vi "输出数据解析.vi"(0 "主板引用":refnum<vi>, 1 "错误代码":i32, 2 "BMU读取结果":refnum<vi>, 3 "命令序号":u8, 4 "输入数组":u8[](array[numeric]), 5 "命令":u8 format="%x", 6 "从板引用":refnum<vi>, 9 "进度引用":refnum<vi>, 10 "板选择":enum16{"主板", "从板"}(ring), 11 "从板个数":refnum<vi>, 12 "二维码信息":refnum<vi>, 13 "从板二维码信息":refnum<vi>, 15 "Socket":dbl) -> (14 "从板数":u8, 17 "写入超时":bool=TRUE, 18 "序号":u8, 19 "状态":bool)   [LabVIEW 2013]
panel:
  in  "从板个数 2":dbl=1.0
  out "子字符串之前":string
  out "从板信息":T1
  out "主板数据 2":T2
  out "充电控制参数":bool
  out "二级故障1 2":bool
  out "一级故障1 6":bool
  out "一级故障1 5":bool
  out "二级故障1":bool
  out "一级故障5":bool
  out "一级故障1 4":bool
  out "一级故障1 3":bool
  out "一级故障1 2":bool
  out "一级故障1":bool
  in  "Ctl引用句柄":refnum<vi>
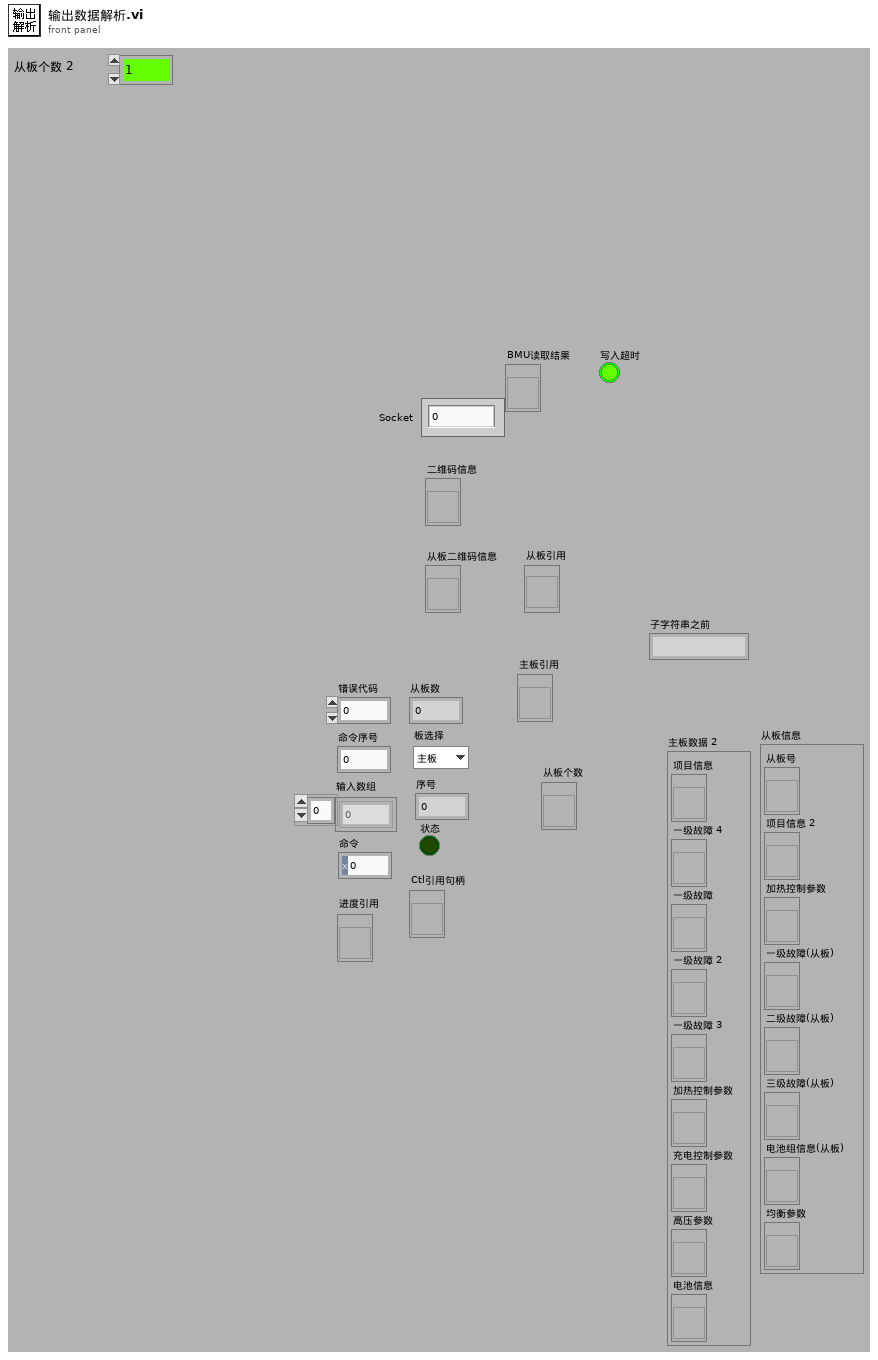
[diagram p1: front panel]
types:
  T1 = cluster{"从板号":refnum<vi>, "项目信息 2":refnum<vi>, "加热控制参数":refnum<vi>, "一级故障(从板)":refnum<vi>, "二级故障(从板)":refnum<vi>, "三级故障(从板)":refnum<vi>, "电池组信息(从板)":refnum<vi>, "均衡参数":refnum<vi>}
  T2 = cluster{"项目信息":refnum<vi>, "一级故障 4":refnum<vi>, "一级故障":refnum<vi>, "一级故障 2":refnum<vi>, "一级故障 3":refnum<vi>, "加热控制参数":refnum<vi>, "充电控制参数":refnum<vi>, "高压参数":refnum<vi>, "电池信息":refnum<vi>}
  T3 = cluster{"电池额定容量":dbl, "使用者":dbl, "电池实际容量":dbl, "车牌号":string, "配置文件版本":string, "SOH":dbl, "SOC":dbl, "产品编号":string, "系统时钟":string}
  T4 = cluster{"电池额定容量(A)":dbl, "使用者":dbl, "电池实际容量(A)":dbl, "车架(牌)号":string, "配置文件版本":string, "SOH(%)":dbl, "SOC(%)":dbl, "产品编号":string, "系统时钟":string}
  T5 = cluster{"总电压过高":dbl, "整组电压不均衡":dbl, "SOC过高":dbl, "单体电压过高":dbl, "总电压过低":dbl, "温度过高":dbl, "温度过低":dbl, "单组电压不均衡":dbl, "整组温度不均衡":dbl, "单组温度不均衡":dbl, "单体电压过低":dbl, "充电电流过高":dbl, "放电电流过高":dbl, "SOC过低":dbl, "内阻过大":dbl, "极柱温度过高":dbl, "SOH过低":dbl}
  T6 = cluster{"风机开启温度":dbl, "风机关闭温度":dbl, "加热开启温度":dbl, "加热关闭温度":dbl, "风机开启温差":dbl, "风机关闭温差":dbl, "加热关闭温差":dbl}
  T7 = cluster{"最大允许单体电压":dbl, "最大允许总电压":dbl, "最小允许单体电压":dbl, "最大允许充电电流":dbl, "最小允许充电电流":dbl, "最大允许充电温度":dbl, "最小允许充电温度":dbl, "电流步长":dbl}
  T8 = cluster{"充电能量阀值":dbl, "放电能量阀值":dbl, "电流增益":dbl, "平均电流":dbl, "电压增益":dbl, "平均电压":dbl}
  T9 = cluster{"电池串联":dbl, "电池并联":dbl, "累计放电总安时":dbl, "电池包额定容量":dbl, "电池包额定能量":dbl, "电池包额定总电压":dbl, "累计充电总安时":dbl, "电池充满次数":dbl, "电池放空次数":dbl, "电池充电次数":dbl, "电池生产日期":string, "电池厂家":string, "电池类型":string, "电池包组号":string, "电池包产权标识":string, "电池应用车型":string, "实际容量":dbl}
  T10 = cluster{"从板号":bool, "电压起始值":bool, "通道电压数":bool, "保险位置":bool, "温度起始值":bool, "一级故障":bool, "二级故障":bool, "三级故障":bool}
  T11 = cluster{"电压过高":dbl, "电压过低":dbl, "温度过高":dbl, "温度过低":dbl, "电压不均衡(V)":dbl, "温度不均衡":dbl, "SOC过低":dbl}
  T12 = cluster{"串联数":dbl, "并联数":dbl, "电池厂家":dbl, "电池类型":dbl, "额定能量":dbl, "额定容量":dbl, "实际容量":dbl, "额定总压":dbl, "产权标识":dbl, "应用车型":dbl, "电池包组号":dbl, "SOC":dbl, "充电总安时":dbl, "放电总这时":dbl, "放空次数":dbl, "充满次数":dbl, "充电次数":dbl, "车牌号":string, "生产日期":string, "最大允许单体电压":dbl, "最大允许总电压":dbl, "最大允许温度":dbl, "最小允许温度":dbl, "最大允许充电电流":dbl, "最小允许充电电流":dbl, "最小允许单体电压":dbl, "电流步长":dbl, "电池包序号":dbl}
  T13 = cluster{"充电结束电压(90%)":sgl, "充电结束电压(91%)":sgl, "充电结束电压(92%)":sgl, "充电结束电压(93%)":sgl, "充电结束电压(94%)":sgl, "均衡计算-电压高阀值1级":sgl, "均衡计算-电压高阀值2级":sgl, "均衡计算-电压低阀值1级":sgl, "均衡计算-电压低阀值2级":sgl, "均衡计算-最低电压阀值":sgl, "均衡停止-最低电压阀值":sgl, "均衡计算-电压极差阀值":sgl, "充电结束电压(95%)":sgl, "充电结束电压(96%)":sgl, "充电结束电压(97%)":sgl, "充电结束电压(98%)":sgl, "充电结束电压(99%)":sgl, "充电结束电压(100%)":sgl}
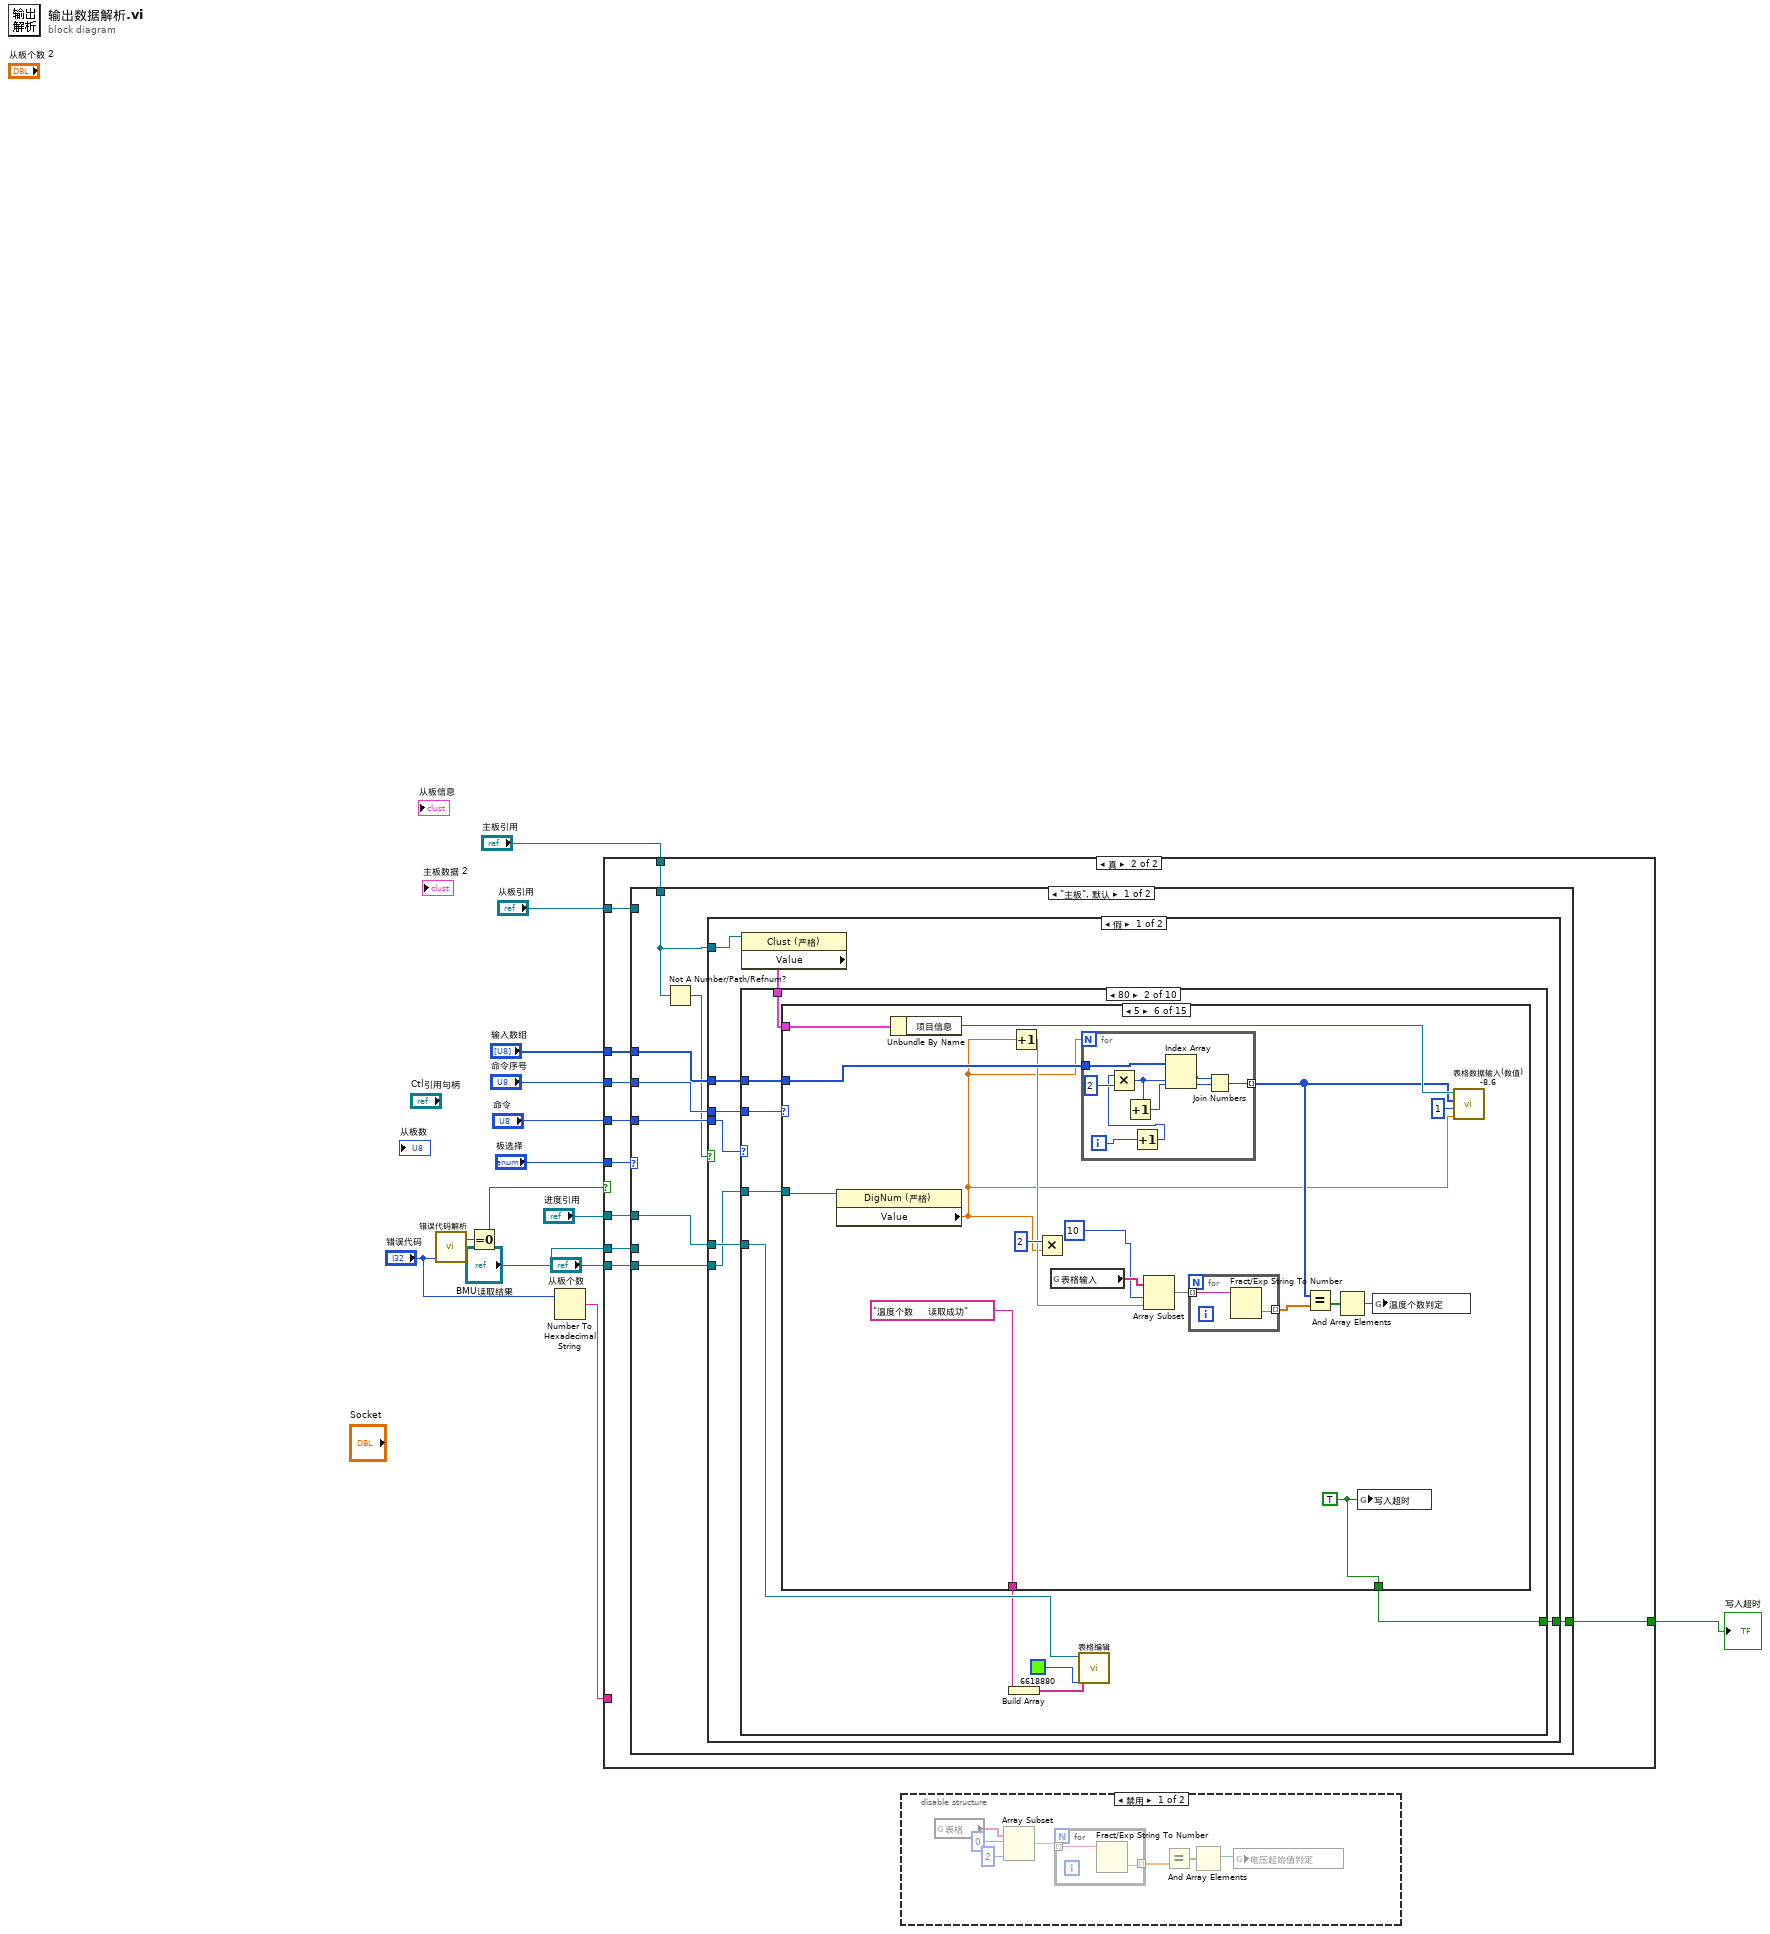
[diagram p0: block diagram]
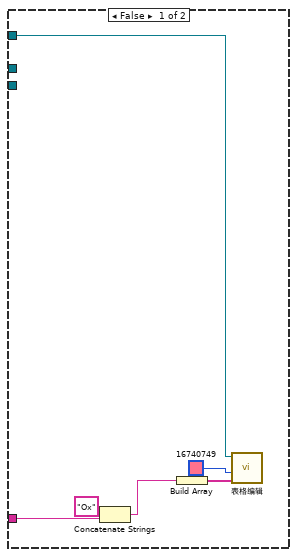
[diagram p3: hidden frame]
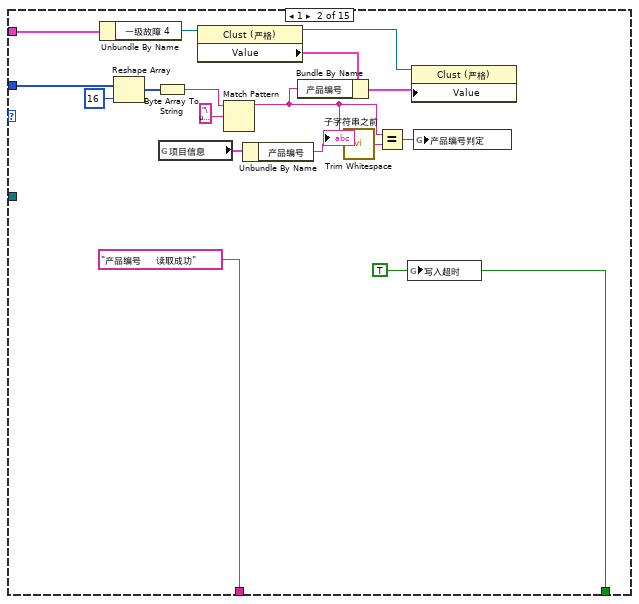
[diagram p6: hidden frame]
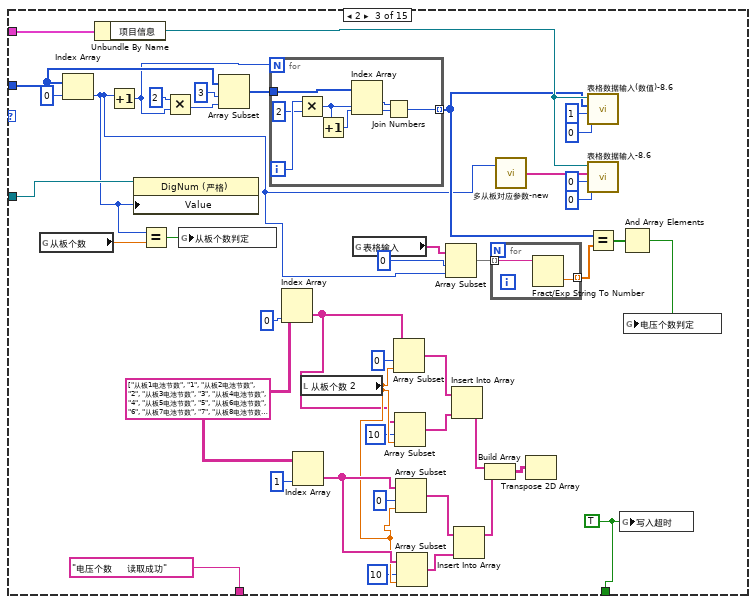
[diagram p7: hidden frame]
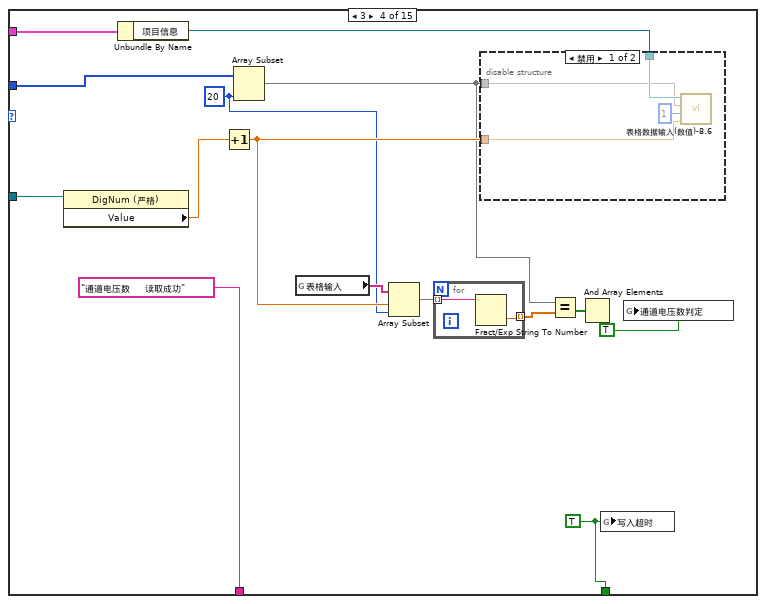
[diagram p8: hidden frame]
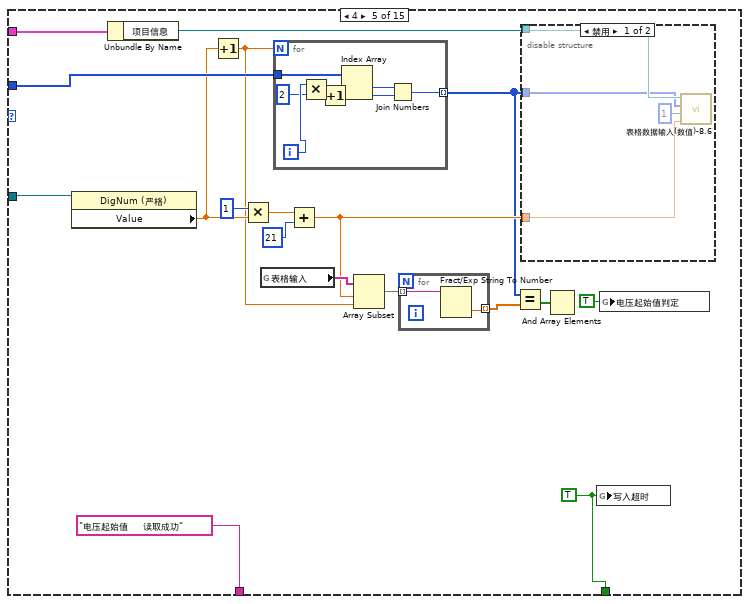
[diagram p10: hidden frame]
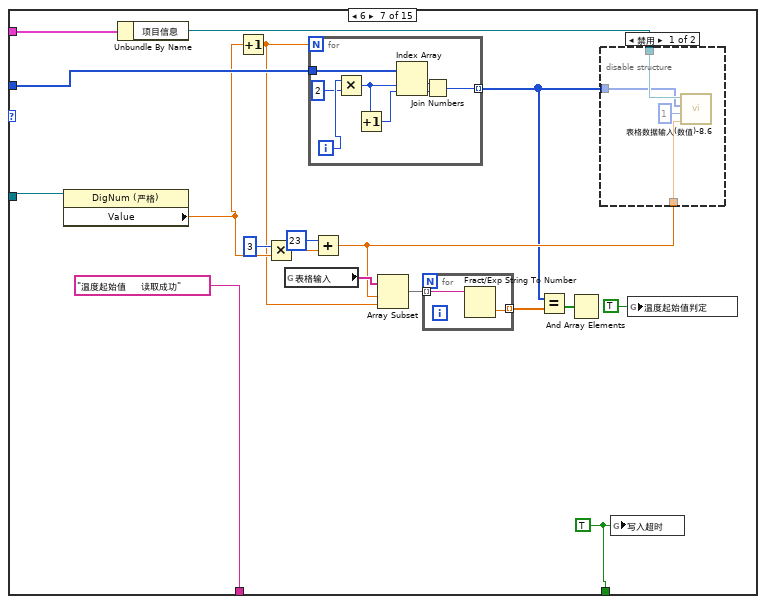
[diagram p12: hidden frame]
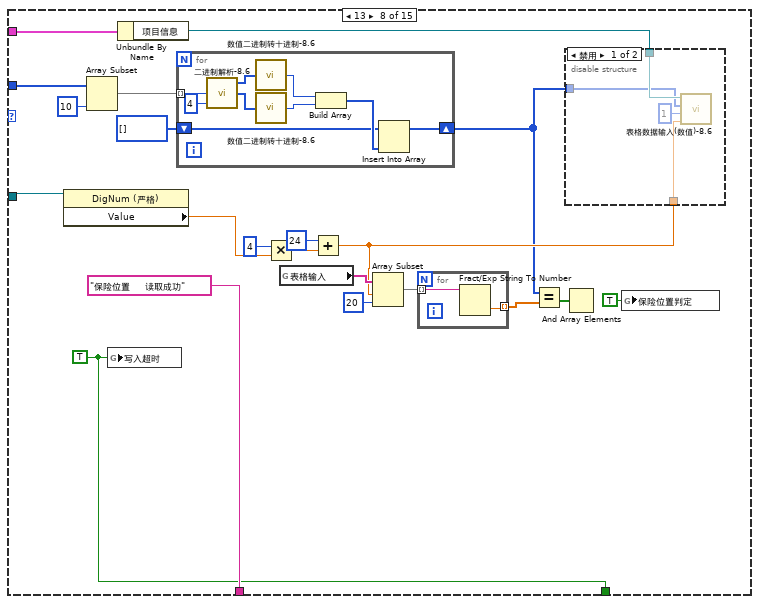
[diagram p14: hidden frame]
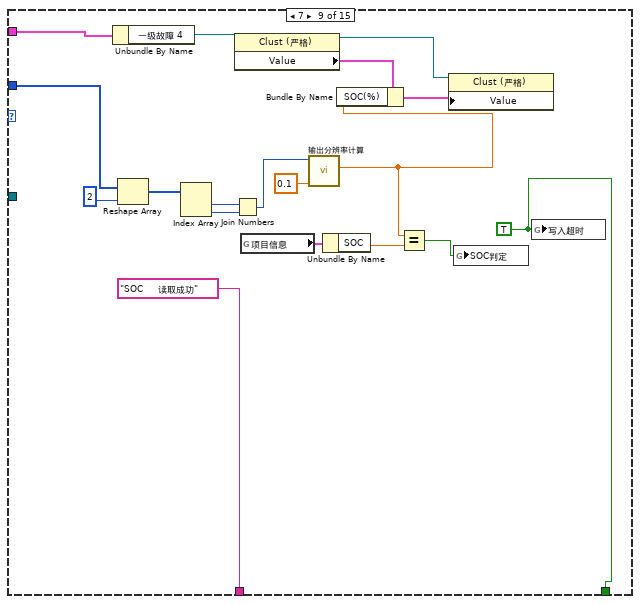
[diagram p16: hidden frame]
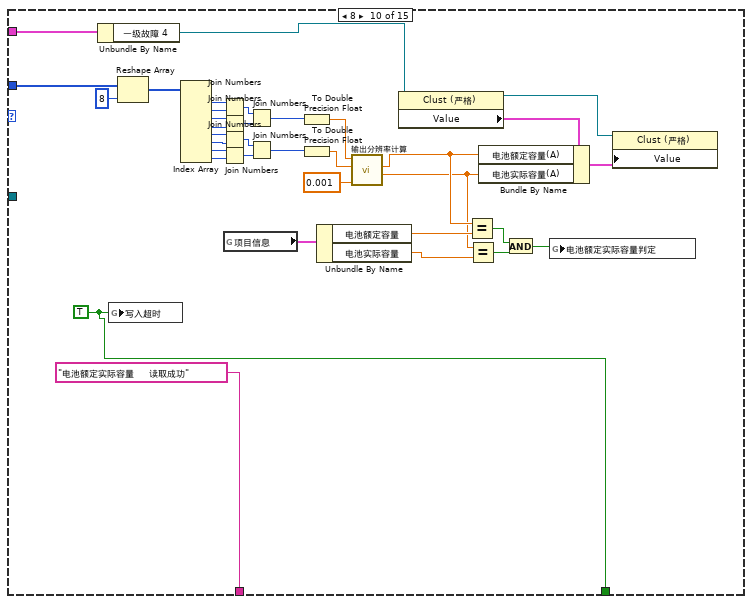
[diagram p17: hidden frame]
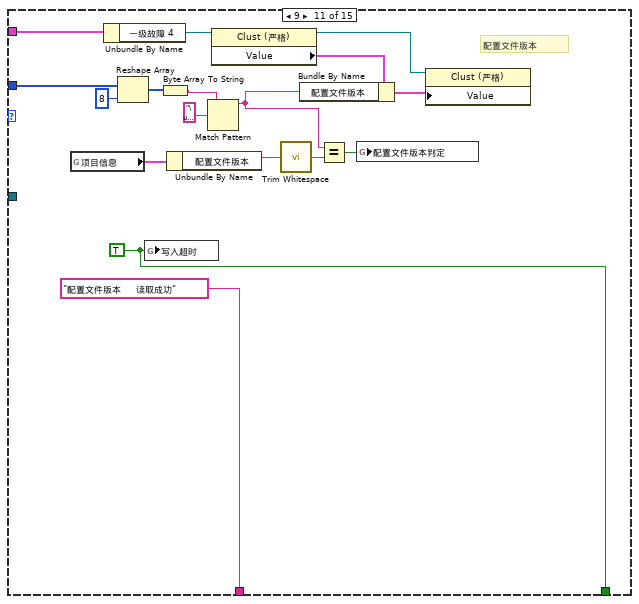
[diagram p18: hidden frame]
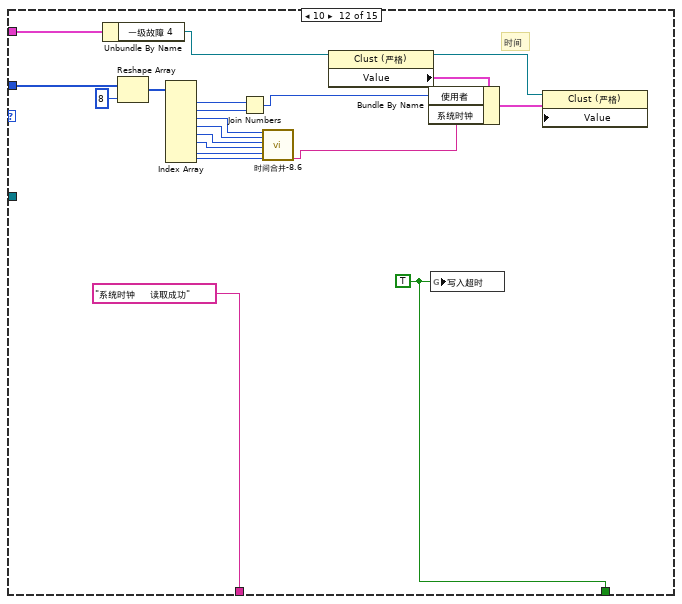
[diagram p19: hidden frame]
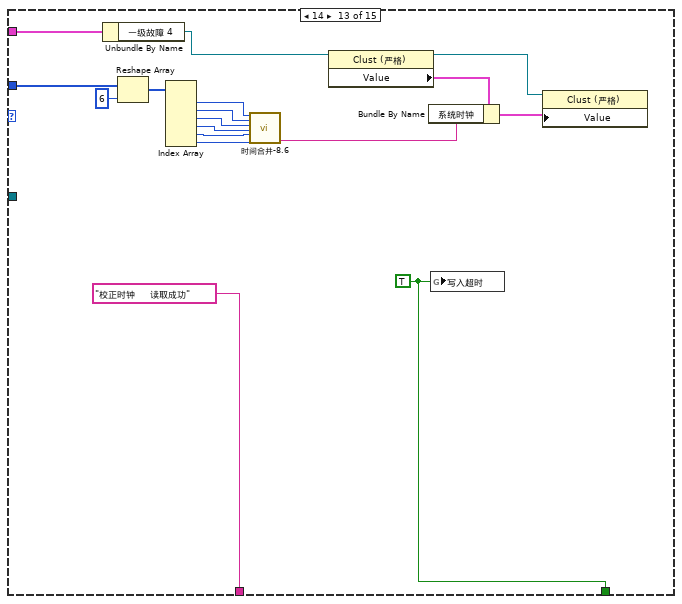
[diagram p20: hidden frame]
diagram:
  n1 = call "错误代码解析.vi"("错误代码"="错误代码") -> ("错误代码"=w14:i32)  [unwired: 2 out]
  n2 = Equal To 0?(x=w14) -> (x = 0?=w13:bool)
  n3 = Number To Hexadecimal String(2:"错误代码") -> (0:w4:string)  [unwired: 1 out]
  n4 = case shown="真" w13 {
    tunnel: "命令" -> [_ w30]
    tunnel: "命令序号" -> [_ w29]
    tunnel: "输入数组" -> [_ w28]
    tunnel: "板选择" -> [_ w27]
    tunnel: "主板引用" -> [_ w26]
    tunnel: "从板引用" -> [_ w25]
    tunnel: "进度引用" -> [w16 w24]
    tunnel: w4 -> [w19 _]
    tunnel: "从板个数" -> [_ w23]
    tunnel: [_ w22] -> w2
    tunnel: "BMU读取结果" -> [_ w21]
    frame False {
      n5 = Concatenate Strings("Ox" ("字符串"), w19) -> (w18:string)
      n6 = Build Array(w18) -> (w17:string[])
      n7 = call "表格编辑.vi"("新元素/子数组"=w17, "活动单元格:单元格背景色"=u32 16740749, "MCListbox引用句柄"=w16) -> ()  [unwired: 9 out]
    }
    frame True {
      n8 = case shown="\"主板\", 默认" w27 {
        tunnel: w30 -> [w38 w1802]
        tunnel: w29 -> [w37 w1801]
        tunnel: w28 -> [w36 w1800]
        tunnel: w26 -> [w33 _]
        tunnel: w25 -> [_ w1798]
        tunnel: w24 -> [w35 w1799]
        tunnel: w23 -> [w32 _]
        tunnel: [w31 w1796] -> w22
        tunnel: w21 -> [_ w1795]
        frame "主板", Default {
          n9 = Not A Number/Path/Refnum?(number/path/refnum=w33) -> (NaN/Path/Refnum?=w34:bool)
          n10 = case shown="假" w34 {
            tunnel: w38 -> [w46 _]
            tunnel: w37 -> [w45 _]
            tunnel: w36 -> [w44 _]
            tunnel: w33 -> [w43 _]
            tunnel: w35 -> [w41 _]
            tunnel: w32 -> [w40 _]
            tunnel: [w39 _] -> w31
            frame False {
              n11 = property class="Clust (严格)"(reference=w43) -> ("Value"=w42:T2)  [unwired: 1 in, 2 out]
              n12 = case shown="80" w46 {
                tunnel: w45 -> [_ w55 w422 w1125 w1311 w1358 w1400 w1573 _ _]
                tunnel: w44 -> [_ w54 w421 w1124 w1310 w1357 w1399 w1572 w1782 w1793]
                tunnel: w42 -> [_ w53 w420 w1123 w1309 w1356 _ w1571 _ _]
                tunnel: w41 -> [_ w51 w419 w1122 w1308 w1355 _ w1568 _ w1787]
                tunnel: w40 -> [_ w49 _ _ _ _ _ _ _ _]
                tunnel: [_ w47 w418 w1121 w1307 w1354 _ w1566 _ w1783] -> w39
                frame 0, Default {
                }
                frame 128 {
                  n13 = case shown="5" w55 {
                    tunnel: w54 -> [_ w72 w108 w141 w160 w192 w220 w252 w293 w328 w345 w365 w382 w399 w415]
                    tunnel: w53 -> [_ w69 w110 w140 w163 w194 w223 w258 w290 w325 w342 w359 w376 w393 w410]
                    tunnel: w49 -> [_ _ w104 w138 w159 w191 w219 w255 _ _ _ _ _ _ _]
                    tunnel: [_ "产品编号     读取成功" ("字符串") "电压个数     读取成功" ("字符串") "通道电压数     读取成功" ("字符串") "电压起始值     读取成功" ("字符串") "温度个数     读取成功" ("字符串") "温度起始值     读取成功" ("字符串") "保险位置     读取成功" ("字符串") "SOC     读取成功" ("字符串") "电池额定实际容量     读取成功" ("字符串") "配置文件版本     读取成功" ("字符串") "系统时钟     读取成功" ("字符串") "校正时钟     读取成功" ("字符串") "车牌号     读取成功" ("字符串") "SOH     读取成功" ("字符串")] -> w48
                    tunnel: [_ w56 w73 w127 w148 w180 w208 w240 w276 w294 w329 w346 w366 w383 w400] -> w47
                    frame 0, Default {
                    }
                    frame 1 {
                      w56 = TRUE ("写入超时")
                      n14 = Unbundle By Name(w69) -> ("一级故障 4"=w68:refnum<vi>)
                      n15 = Reshape Array(w72, 16 ("维数大小")) -> (w71:u8[])
                      n16 = Byte Array To String(unsigned byte array=w71) -> (string=w58:string)
                      n17 = global read "读配置文件全局.vi" "项目信息"() -> (w64:T3)
                      n18 = property class="Clust (严格)"(reference=w68) -> (reference out=w66:refnum<vi>, "Value"=w67:T4)  [unwired: 1 in, 1 out]
                      n19 = Match Pattern(string=w58, regular expression="\u0000" ("trimmed string")) -> (before substring=w57:string)  [unwired: 1 in, 3 out]
                      "子字符串之前" <- w57
                      n20 = Unbundle By Name(w64) -> ("产品编号"=w62:string)
                      n21 = Bundle By Name(cluster=w67, "产品编号"=w57) -> (w63:T4)
                      n22 = call <vilib>:"Trim Whitespace.vi"("string"=w62) -> ("trimmed string"=w60:string)  [unwired: 1 in]
                      n23 = Equal?(x=w57, y=w60) -> (x = y?=w61:bool)
                      n24 = global write "EV05全局变量1.vi" "写入超时"(w56) -> ()
                      n25 = property class="Clust (严格)"(reference=w66, "Value"=w63) -> ()  [unwired: 1 in, 2 out]
                      n26 = global write "读配置文件全局.vi" "产品编号判定"(w61) -> ()
                    }
                    frame 2 {
                      w80 = string[][] [["从板1电池节数", "1"], ["从板2电池节数", "2"], ["从板3电池节数", "3"], ["从板4电池节数", "4"], ["从板5电池节数", "5"], ["从板6电池节数", "6"], ["从板7电池节数", "7"], ["从板8电池节数", "8"], ["从板9电池节数", "9"], ["从板10电池节数", "10"], ["从板1温度个数", "1"], ["从板2温度个数", "2"], ["从板3温度个数", "3"], ["从板4温度个数", "4"], ["从板5温度个数", "5"], ["从板6温度个数", "6"], ["从板7温度个数", "7"], ["从板8温度个数", "8"], ["从板9温度个数", "9"], ["从板10温度个数", "10"]] ("项目信息")
                      w73 = TRUE ("写入超时")
                      n27 = global read "读配置文件全局.vi" "从板个数"() -> (w102:dbl)
                      n28 = Index Array(array=w108, index=0 ("索引")) -> (element=w91:u8)
                      n29 = Unbundle By Name(w110) -> ("项目信息"=w109:refnum<vi>)
                      n30 = Increment(x=w91) -> (x+1=w92:u8)
                      n31 = property class="DigNum (严格)"(reference=w104, "Value"=w91) -> ()  [unwired: 1 in, 2 out]
                      n32 = Equal?(x=w91, y=w102) -> (x = y?=w101:bool)
                      n33 = Multiply(x=u8 2, y=w92) -> (x*y=w93:u8)
                      n34 = global write "读配置文件全局.vi" "从板个数判定"(w101) -> ()
                      n35 = Array Subset(array=w108, index=3 ("索引"), length=w93) -> (w106:u8[])
                      n36 = for {
                        N: w92 -> [_]
                        tunnel: w106 -> [w126]
                        tunnel: [w119] -> w96 mode=indexing
                        i -> [w125]
                        n37 = Multiply(x=w125, y=2) -> (x*y=w123:i32)
                        n38 = Increment(x=w123) -> (x+1=w122:i32)
                        n39 = Index Array(array=w126, index #1=w123, index #2=w122) -> (element #1=w120:u8, element #2=w121:u8)
                        n40 = Join Numbers(hi=w120, lo=w121) -> ((hi.lo)=w119:u16)
                      }
                      n41 = Index Array(array=w80, index (col)=0 ("索引 (行)")) -> (element=w77:string[])  [unwired: 1 in]
                      n42 = Index Array(array=w80, index (col)=1 ("禁用的索引 (列)")) -> (element=w87:string[])  [unwired: 1 in]
                      n43 = local read "从板个数 2"() -> (w85:dbl)
                      n44 = global read "读配置文件全局.vi" "表格输入"() -> (w100:string[])
                      n45 = Array Subset(array=w77, index=0 ("索引"), length=w85) -> (w78:string[])
                      n46 = Array Subset(array=w77, index=10 ("索引"), length=w85) -> (w79:string[])
                      n47 = Array Subset(array=w87, index=0 ("索引"), length=w85) -> (w81:string[])
                      n48 = Array Subset(array=w87, index=10 ("索引"), length=w85) -> (w86:string[])
                      n49 = Array Subset(array=w100, index=0 ("索引"), length=w91) -> (w98:string[])
                      n50 = Insert Into Array(array=w78, new element=w79) -> (w88:string[])  [unwired: 1 in]
                      n51 = Insert Into Array(array=w81, new element=w86) -> (w89:string[])  [unwired: 1 in]
                      n52 = Build Array(w88, w89) -> (w90:string[][])
                      n53 = for {
                        tunnel: w98 -> [w118] mode=indexing
                        tunnel: [w117] -> w97 mode=indexing
                        n54 = Fract/Exp String To Number(string=w118) -> (number=w117:dbl)  [unwired: 4 out]
                      }
                      n55 = call "多从板对应参数-new.vi"("从板个数"=w91) -> ("输出数组"=w113:string[])  [unwired: 1 in]
                      n56 = Transpose 2D Array(2D array=w90) -> ()  [unwired: 1 out]
                      n57 = call "表格数据输入(数值)-8.6.vi"("行数"=u32 0, "列数"=u32 1, "数值数组"=w96, "表格引用"=w109) -> ()  [unwired: 8 out]
                      n58 = call "表格数据输入-8.6.vi"("行数"=u32 0, "列数"=u32 0, "字符串数组"=w113, "表格引用"=w109) -> ()  [unwired: 8 out]
                      n59 = Equal?(x=w96, y=w97) -> (x = y?=w95:bool[])
                      n60 = global write "EV05全局变量1.vi" "写入超时"(w73) -> ()
                      n61 = And Array Elements(Boolean array=w95) -> (logical AND=w94:bool)
                      n62 = global write "读配置文件全局.vi" "电压个数判定"(w94) -> ()
                    }
                    frame 3 {
                      w127 = TRUE ("写入超时")
                      w132 = 20 ("长度")
                      n63 = property class="DigNum (严格)"(reference=w138) -> ("Value"=w137:dbl)  [unwired: 1 in, 2 out]
                      n64 = Unbundle By Name(w140) -> ("项目信息"=w139:refnum<vi>)
                      n65 = Increment(x=w137) -> (x+1=w133:dbl)
                      n66 = Array Subset(array=w141, length=w132) -> (w130:u8[])  [unwired: 1 in]
                      n67 = global read "读配置文件全局.vi" "表格输入"() -> (w135:string[])
                      n68 = Array Subset(array=w135, index=w133, length=w132) -> (w134:string[])
                      n69 = for {
                        tunnel: w134 -> [w147] mode=indexing
                        tunnel: [w146] -> w131 mode=indexing
                        n70 = Fract/Exp String To Number(string=w147) -> (number=w146:dbl)  [unwired: 4 out]
                      }
                      n71 = disable-structure shown="禁用" {
                        disable-tunnel: w139 -> [w144 _]
                        disable-tunnel: w133 -> [w143 _]
                        disable-tunnel: w130 -> [w142 _]
                        frame Disabled {
                          n72 = call "表格数据输入(数值)-8.6.vi"("行数"=w143, "列数"=u32 1, "数值数组"=w142, "表格引用"=w144) -> ()  [unwired: 8 out]
                        }
                        frame Enabled {
                        }
                      }
                      n73 = Equal?(x=w130, y=w131) -> (x = y?=w129:bool[])
                      n74 = And Array Elements(Boolean array=w129) -> ()  [unwired: 1 out]
                      n75 = global write "EV05全局变量1.vi" "写入超时"(w127) -> ()
                      n76 = global write "读配置文件全局.vi" "通道电压数判定"(TRUE ("通道电压数判定")) -> ()
                    }
                    frame 4 {
                      w148 = TRUE ("写入超时")
                      n77 = property class="DigNum (严格)"(reference=w159) -> ("Value"=w158:dbl)  [unwired: 1 in, 2 out]
                      n78 = Unbundle By Name(w163) -> ("项目信息"=w162:refnum<vi>)
                      n79 = Increment(x=w158) -> (x+1=w151:dbl)
                      n80 = Multiply(x=u8 1, y=w158) -> (x*y=w164:dbl)
                      n81 = global read "读配置文件全局.vi" "表格输入"() -> (w156:string[])
                      n82 = for {
                        N: w151 -> [_]
                        tunnel: w160 -> [w179]
                        tunnel: [w172] -> w150 mode=indexing
                        i -> [w178]
                        n83 = Multiply(x=w178, y=2) -> (x*y=w176:i32)
                        n84 = Increment(x=w176) -> (x+1=w175:i32)
                        n85 = Index Array(array=w179, index #1=w176, index #2=w175) -> (element #1=w173:u8, element #2=w174:u8)
                        n86 = Join Numbers(hi=w173, lo=w174) -> ((hi.lo)=w172:u16)
                      }
                      n87 = Add(x=w164, y=u8 21) -> (x+y=w152:dbl)
                      n88 = Array Subset(array=w156, index=w152, length=w151) -> (w155:string[])
                      n89 = for {
                        tunnel: w155 -> [w171] mode=indexing
                        tunnel: [w170] -> w154 mode=indexing
                        n90 = Fract/Exp String To Number(string=w171) -> (number=w170:dbl)  [unwired: 4 out]
                      }
                      n91 = Equal?(x=w150, y=w154) -> (x = y?=w153:bool[])
                      n92 = disable-structure shown="禁用" {
                        disable-tunnel: w162 -> [w168 _]
                        disable-tunnel: w152 -> [w167 _]
                        disable-tunnel: w150 -> [w166 _]
                        frame Disabled {
                          n93 = call "表格数据输入(数值)-8.6.vi"("行数"=w167, "列数"=u32 1, "数值数组"=w166, "表格引用"=w168) -> ()  [unwired: 8 out]
                        }
                        frame Enabled {
                        }
                      }
                      n94 = And Array Elements(Boolean array=w153) -> ()  [unwired: 1 out]
                      n95 = global write "EV05全局变量1.vi" "写入超时"(w148) -> ()
                      n96 = global write "读配置文件全局.vi" "电压起始值判定"(TRUE ("电压起始值判定")) -> ()
                    }
                    frame 5 {
                      w180 = TRUE ("写入超时")
                      n97 = property class="DigNum (严格)"(reference=w191) -> ("Value"=w182:dbl)  [unwired: 1 in, 2 out]
                      n98 = Unbundle By Name(w194) -> ("项目信息"=w193:refnum<vi>)
                      n99 = Increment(x=w182) -> (x+1=w184:dbl)
                      n100 = Multiply(x=u8 2, y=w182) -> ()  [unwired: 1 out]
                      n101 = global read "读配置文件全局.vi" "表格输入"() -> (w189:string[])
                      n102 = for {
                        N: w182 -> [_]
                        tunnel: w192 -> [w207]
                        tunnel: [w201] -> w183 mode=indexing
                        i -> [w200]
                        n103 = Increment(x=w200) -> (x+1=w199:i32)
                        n104 = Multiply(x=w199, y=2) -> (x*y=w205:i32)
                        n105 = Increment(x=w205) -> (x+1=w204:i32)
                        n106 = Index Array(array=w207, index #1=w205, index #2=w204) -> (element #1=w202:u8, element #2=w203:u8)
                        n107 = Join Numbers(hi=w202, lo=w203) -> ((hi.lo)=w201:u16)
                      }
                      n108 = Array Subset(array=w189, index=u8 10 ("x"), length=w184) -> (w188:string[])
                      n109 = for {
                        tunnel: w188 -> [w198] mode=indexing
                        tunnel: [w197] -> w187 mode=indexing
                        n110 = Fract/Exp String To Number(string=w198) -> (number=w197:dbl)  [unwired: 4 out]
                      }
                      n111 = Equal?(x=w183, y=w187) -> (x = y?=w186:bool[])
                      n112 = And Array Elements(Boolean array=w186) -> (logical AND=w185:bool)
                      n113 = global write "EV05全局变量1.vi" "写入超时"(w180) -> ()
                      n114 = global write "读配置文件全局.vi" "温度个数判定"(w185) -> ()
                      n115 = call "表格数据输入(数值)-8.6.vi"("行数"=w182, "列数"=u32 1, "数值数组"=w183, "表格引用"=w193) -> ()  [unwired: 8 out]
                    }
                    frame 6 {
                      w208 = TRUE ("写入超时")
                      n116 = property class="DigNum (严格)"(reference=w219) -> ("Value"=w218:dbl)  [unwired: 1 in, 2 out]
                      n117 = Unbundle By Name(w223) -> ("项目信息"=w222:refnum<vi>)
                      n118 = Increment(x=w218) -> (x+1=w211:dbl)
                      n119 = Multiply(x=u8 3, y=w218) -> (x*y=w224:dbl)
                      n120 = global read "读配置文件全局.vi" "表格输入"() -> (w216:string[])
                      n121 = for {
                        N: w211 -> [_]
                        tunnel: w220 -> [w239]
                        tunnel: [w232] -> w210 mode=indexing
                        i -> [w238]
                        n122 = Multiply(x=w238, y=2) -> (x*y=w236:i32)
                        n123 = Increment(x=w236) -> (x+1=w235:i32)
                        n124 = Index Array(array=w239, index #1=w236, index #2=w235) -> (element #1=w233:u8, element #2=w234:u8)
                        n125 = Join Numbers(hi=w233, lo=w234) -> ((hi.lo)=w232:u16)
                      }
                      n126 = Add(x=u8 23, y=w224) -> (x+y=w212:dbl)
                      n127 = Array Subset(array=w216, index=w212, length=w211) -> (w215:string[])
                      n128 = for {
                        tunnel: w215 -> [w231] mode=indexing
                        tunnel: [w230] -> w214 mode=indexing
                        n129 = Fract/Exp String To Number(string=w231) -> (number=w230:dbl)  [unwired: 4 out]
                      }
                      n130 = Equal?(x=w210, y=w214) -> (x = y?=w213:bool[])
                      n131 = And Array Elements(Boolean array=w213) -> ()  [unwired: 1 out]
                      n132 = disable-structure shown="禁用" {
                        disable-tunnel: w222 -> [w228 _]
                        disable-tunnel: w212 -> [w227 _]
                        disable-tunnel: w210 -> [w226 _]
                        frame Disabled {
                          n133 = call "表格数据输入(数值)-8.6.vi"("行数"=w227, "列数"=u32 1, "数值数组"=w226, "表格引用"=w228) -> ()  [unwired: 8 out]
                        }
                        frame Enabled {
                        }
                      }
                      n134 = global write "EV05全局变量1.vi" "写入超时"(w208) -> ()
                      n135 = global write "读配置文件全局.vi" "温度起始值判定"(TRUE ("温度起始值判定")) -> ()
                    }
                    frame 13 {
                      w240 = TRUE ("写入超时")
                      n136 = property class="DigNum (严格)"(reference=w255) -> ("Value"=w254:dbl)  [unwired: 1 in, 2 out]
                      n137 = Array Subset(array=w252, length=10 ("长度")) -> (w244:u8[])  [unwired: 1 in]
                      n138 = global write "EV05全局变量1.vi" "写入超时"(w240) -> ()
                      n139 = Unbundle By Name(w258) -> ("项目信息"=w257:refnum<vi>)
                      n140 = for {
                        tunnel: w244 -> [w273] mode=indexing
                        shift-right: [w266] -> w243
                        shift-left: i32[] [] -> [w265]
                        n141 = call "二进制解析-8.6.vi"("索引"=4, "数值"=w273) -> ("低位子数组"=w271:i32[], "高位子数组"=w270:i32[])  [unwired: 1 in, 1 out]
                        n142 = call "数值二进制转十进制-8.6.vi"("子数组"=w270) -> ("十进制数值"=w269:i32)  [unwired: 4 in]
                        n143 = call "数值二进制转十进制-8.6.vi"("子数组"=w271) -> ("十进制数值"=w268:i32)  [unwired: 4 in]
                        n144 = Build Array(w269, w268) -> (w267:i32[])
                        n145 = Insert Into Array(array=w265, new element=w267) -> (w266:i32[])  [unwired: 1 in]
                      }
                      n146 = Multiply(x=u8 4, y=w254) -> (x*y=w259:dbl)
                      n147 = global read "读配置文件全局.vi" "表格输入"() -> (w250:string[])
                      n148 = Add(x=u8 24, y=w259) -> (x+y=w246:dbl)
                      n149 = Array Subset(array=w250, index=w246, length=20 ("长度")) -> (w249:string[])
                      n150 = for {
                        tunnel: w249 -> [w275] mode=indexing
                        tunnel: [w274] -> w248 mode=indexing
                        n151 = Fract/Exp String To Number(string=w275) -> (number=w274:dbl)  [unwired: 4 out]
                      }
                      n152 = Equal?(x=w243, y=w248) -> (x = y?=w247:bool[])
                      n153 = disable-structure shown="禁用" {
                        disable-tunnel: w257 -> [w263 _]
                        disable-tunnel: w246 -> [w262 _]
                        disable-tunnel: w243 -> [w261 _]
                        frame Disabled {
                          n154 = call "表格数据输入(数值)-8.6.vi"("行数"=w262, "列数"=u32 1, "数值数组"=w261, "表格引用"=w263) -> ()  [unwired: 8 out]
                        }
                        frame Enabled {
                        }
                      }
                      n155 = And Array Elements(Boolean array=w247) -> ()  [unwired: 1 out]
                      n156 = global write "读配置文件全局.vi" "保险位置判定"(TRUE ("保险位置判定")) -> ()
                    }
                    frame 7 {
                      w276 = TRUE ("写入超时")
                      n157 = Unbundle By Name(w290) -> ("一级故障 4"=w286:refnum<vi>)
                      n158 = Reshape Array(w293, 2 ("维数大小")) -> (w291:u8[])
                      n159 = Index Array(array=w291) -> (element #1=w283:u8, element #2=w282:u8)  [unwired: 2 in]
                      n160 = Join Numbers(hi=w283, lo=w282) -> ((hi.lo)=w281:u16)
                      n161 = property class="Clust (严格)"(reference=w286) -> (reference out=w288:refnum<vi>, "Value"=w289:T4)  [unwired: 1 in, 1 out]
                      n162 = global read "读配置文件全局.vi" "项目信息"() -> (w280:T3)
                      n163 = call "输出分辨率计算.vi"("分辨率"=0.1, "数值 2"=w281) -> ("输出2"=w278:dbl)  [unwired: 4 in, 5 out]
                      n164 = Unbundle By Name(w280) -> ("SOC"=w279:dbl)
                      n165 = Bundle By Name(cluster=w289, "SOC(%)"=w278) -> (w287:T4)
                      n166 = Equal?(x=w278, y=w279) -> (x = y?=w277:bool)
                      n167 = property class="Clust (严格)"(reference=w288, "Value"=w287) -> ()  [unwired: 1 in, 2 out]
                      n168 = global write "读配置文件全局.vi" "SOC判定"(w277) -> ()
                      n169 = global write "EV05全局变量1.vi" "写入超时"(w276) -> ()
                    }
                    frame 8 {
                      w294 = TRUE ("写入超时")
                      n170 = Unbundle By Name(w325) -> ("一级故障 4"=w321:refnum<vi>)
                      n171 = global write "EV05全局变量1.vi" "写入超时"(w294) -> ()
                      n172 = Reshape Array(w328, 8 ("维数大小")) -> (w326:u8[])
                      n173 = Index Array(array=w326) -> (element #1=w316:u8, element #2=w317:u8, element #3=w315:u8, element #4=w314:u8, element #5=w307:u8, element #6=w306:u8, element #7=w305:u8, element #8=w304:u8)  [unwired: 8 in]
                      n174 = Join Numbers(hi=w316, lo=w317) -> ((hi.lo)=w312:u16)
                      n175 = Join Numbers(hi=w315, lo=w314) -> ((hi.lo)=w313:u16)
                      n176 = Join Numbers(hi=w307, lo=w306) -> ((hi.lo)=w309:u16)
                      n177 = Join Numbers(hi=w305, lo=w304) -> ((hi.lo)=w308:u16)
                      n178 = global read "读配置文件全局.vi" "项目信息"() -> (w302:T3)
                      n179 = Join Numbers(hi=w312, lo=w313) -> ((hi.lo)=w311:u32)
                      n180 = Join Numbers(hi=w309, lo=w308) -> ((hi.lo)=w310:u32)
                      n181 = To Double Precision Float(number=w311) -> (double precision float=w318:dbl)
                      n182 = To Double Precision Float(number=w310) -> (double precision float=w303:dbl)
                      n183 = Unbundle By Name(w302) -> ("电池额定容量"=w300:dbl, "电池实际容量"=w298:dbl)
                      n184 = call "输出分辨率计算.vi"("分辨率"=0.001, "数值 3"=w303, "数值 2"=w318) -> ("输出3"=w299:dbl, "输出2"=w301:dbl)  [unwired: 3 in, 4 out]
                      n185 = property class="Clust (严格)"(reference=w321) -> (reference out=w323:refnum<vi>, "Value"=w324:T4)  [unwired: 1 in, 1 out]
                      n186 = Equal?(x=w301, y=w300) -> (x = y?=w296:bool)
                      n187 = Equal?(x=w299, y=w298) -> (x = y?=w297:bool)
                      n188 = Bundle By Name(cluster=w324, "电池额定容量(A)"=w301, "电池实际容量(A)"=w299) -> (w322:T4)
                      n189 = And(x=w296, y=w297) -> (x .and. y?=w295:bool)
                      n190 = global write "读配置文件全局.vi" "电池额定实际容量判定"(w295) -> ()
                      n191 = property class="Clust (严格)"(reference=w323, "Value"=w322) -> ()  [unwired: 1 in, 2 out]
                    }
                    frame 9 {
                      w329 = TRUE ("写入超时")
                      # "配置文件版本"
                      n192 = global read "读配置文件全局.vi" "项目信息"() -> (w336:T3)
                      n193 = Unbundle By Name(w342) -> ("一级故障 4"=w338:refnum<vi>)
                      n194 = Reshape Array(w345, 8 ("维数大小")) -> (w343:u8[])
                      n195 = global write "EV05全局变量1.vi" "写入超时"(w329) -> ()
                      n196 = Byte Array To String(unsigned byte array=w343) -> (string=w331:string)
                      n197 = Unbundle By Name(w336) -> ("配置文件版本"=w335:string)
                      n198 = Match Pattern(string=w331, regular expression="\u0000" ("trimmed string")) -> (before substring=w330:string)  [unwired: 1 in, 3 out]
                      n199 = property class="Clust (严格)"(reference=w338) -> (reference out=w340:refnum<vi>, "Value"=w341:T4)  [unwired: 1 in, 1 out]
                      n200 = call <vilib>:"Trim Whitespace.vi"("string"=w335) -> ("trimmed string"=w334:string)  [unwired: 1 in]
                      n201 = Bundle By Name(cluster=w341, "配置文件版本"=w330) -> (w339:T4)
                      n202 = Equal?(x=w330, y=w334) -> (x = y?=w333:bool)
                      n203 = global write "读配置文件全局.vi" "配置文件版本判定"(w333) -> ()
                      n204 = property class="Clust (严格)"(reference=w340, "Value"=w339) -> ()  [unwired: 1 in, 2 out]
                    }
                    frame 10 {
                      w346 = TRUE ("写入超时")
                      # "时间"
                      n205 = Unbundle By Name(w359) -> ("一级故障 4"=w358:refnum<vi>)
                      n206 = Reshape Array(w365, 8 ("维数大小")) -> (w363:u8[])
                      n207 = Index Array(array=w363) -> (element #1=w349:u8, element #2=w350:u8, element #3=w351:u8, element #4=w352:u8, element #5=w353:u8, element #6=w354:u8, element #7=w355:u8, element #8=w356:u8)  [unwired: 8 in]
                      n208 = Join Numbers(hi=w349, lo=w350) -> ((hi.lo)=w348:u16)
                      n209 = call "时间合并-8.6.vi"("年"=w351, "月"=w352, "日"=w353, "时"=w354, "分"=w355, "秒"=w356) -> ("时间"=w357:string)  [unwired: 13 out]
                      n210 = property class="Clust (严格)"(reference=w358) -> (reference out=w361:refnum<vi>, "Value"=w362:T4)  [unwired: 1 in, 1 out]
                      n211 = Bundle By Name(cluster=w362, "使用者"=w348, "系统时钟"=w357) -> (w360:T4)
                      n212 = global write "EV05全局变量1.vi" "写入超时"(w346) -> ()
                      n213 = property class="Clust (严格)"(reference=w361, "Value"=w360) -> ()  [unwired: 1 in, 2 out]
                    }
                    frame 14 {
                      w366 = TRUE ("写入超时")
                      n214 = Unbundle By Name(w376) -> ("一级故障 4"=w375:refnum<vi>)
                      n215 = Reshape Array(w382, 6 ("维数大小")) -> (w380:u8[])
                      n216 = Index Array(array=w380) -> (element #1=w372:u8, element #2=w371:u8, element #3=w370:u8, element #4=w369:u8, element #5=w368:u8, element #6=w367:u8)  [unwired: 6 in]
                      n217 = call "时间合并-8.6.vi"("年"=w372, "月"=w371, "日"=w370, "时"=w369, "分"=w368, "秒"=w367) -> ("时间"=w374:string)  [unwired: 13 out]
                      n218 = property class="Clust (严格)"(reference=w375) -> (reference out=w378:refnum<vi>, "Value"=w379:T4)  [unwired: 1 in, 1 out]
                      n219 = Bundle By Name(cluster=w379, "系统时钟"=w374) -> (w377:T4)
                      n220 = global write "EV05全局变量1.vi" "写入超时"(w366) -> ()
                      n221 = property class="Clust (严格)"(reference=w378, "Value"=w377) -> ()  [unwired: 1 in, 2 out]
                    }
                    frame 11 {
                      w383 = TRUE ("写入超时")
                      # "车牌号"
                      n222 = Unbundle By Name(w393) -> ("一级故障 4"=w392:refnum<vi>)
                      n223 = Reshape Array(w399, 8 ("维数大小")) -> (w397:u8[])
                      n224 = global read "读配置文件全局.vi" "项目信息"() -> (w390:T3)
                      n225 = Byte Array To String(unsigned byte array=w397) -> (string=w385:string)
                      n226 = property class="Clust (严格)"(reference=w392) -> (reference out=w395:refnum<vi>, "Value"=w396:T4)  [unwired: 1 in, 1 out]
                      n227 = Unbundle By Name(w390) -> ("车牌号"=w389:string)
                      n228 = Match Pattern(string=w385, regular expression="\u0000" ("trimmed string")) -> (before substring=w384:string)  [unwired: 1 in, 3 out]
                      n229 = call <vilib>:"Trim Whitespace.vi"("string"=w389) -> ("trimmed string"=w388:string)  [unwired: 1 in]
                      n230 = Bundle By Name(cluster=w396, "车架(牌)号"=w384) -> (w394:T4)
                      n231 = Equal?(x=w384, y=w388) -> (x = y?=w387:bool)
                      n232 = global write "读配置文件全局.vi" "车牌号判定"(w387) -> ()
                      n233 = global write "EV05全局变量1.vi" "写入超时"(w383) -> ()
                      n234 = property class="Clust (严格)"(reference=w395, "Value"=w394) -> ()  [unwired: 1 in, 2 out]
                    }
                    frame 12 {
                      w400 = TRUE ("写入超时")
                      # "SOH"
                      n235 = Unbundle By Name(w410) -> ("一级故障 4"=w409:refnum<vi>)
                      n236 = Reshape Array(w415, 2 ("维数大小")) -> (w416:u8[])
                      n237 = Index Array(array=w416) -> (element #1=w407:u8, element #2=w408:u8)  [unwired: 2 in]
                      n238 = Join Numbers(hi=w407, lo=w408) -> ((hi.lo)=w406:u16)
                      n239 = property class="Clust (严格)"(reference=w409) -> (reference out=w412:refnum<vi>, "Value"=w413:T4)  [unwired: 1 in, 1 out]
                      n240 = global read "读配置文件全局.vi" "项目信息"() -> (w404:T3)
                      n241 = Unbundle By Name(w404) -> ("SOH"=w402:dbl)
                      n242 = call "输出分辨率计算.vi"("分辨率"=0.1, "数值 2"=w406) -> ("输出2"=w403:dbl)  [unwired: 4 in, 5 out]
                      n243 = Equal?(x=w403, y=w402) -> (x = y?=w401:bool)
                      n244 = Bundle By Name(cluster=w413, "SOH(%)"=w403) -> (w411:T4)
                      n245 = global write "读配置文件全局.vi" "SOH判定"(w401) -> ()
                      n246 = property class="Clust (严格)"(reference=w412, "Value"=w411) -> ()  [unwired: 1 in, 2 out]
                      n247 = global write "EV05全局变量1.vi" "写入超时"(w400) -> ()
                    }
                  }
                  n248 = Build Array(w48) -> (w52:string[])
                  n249 = call "表格编辑.vi"("新元素/子数组"=w52, "活动单元格:单元格背景色"=u32 6618880, "MCListbox引用句柄"=w51) -> ()  [unwired: 9 out]
                }
                frame 129 {
                  n250 = case shown="1" w422 {
                    tunnel: w421 -> [_ w433 w667 w899]
                    tunnel: w420 -> [_ w429 w663 w895]
                    tunnel: w419 -> [_ w424 w659 w890]
                    tunnel: [_ w423 w657 w889] -> w418
                    frame 0, Default {
                    }
                    frame 1 {
                      w423 = TRUE ("写入超时")
                      n251 = Unbundle By Name(w429) -> ("一级故障"=w428:refnum<vi>)
                      n252 = Reshape Array(w433, 28 ("维数大小")) -> (w430:u8[])
                      n253 = for {
                        N: 4 -> [_]
                        tunnel: w430 -> [w455]
                        tunnel: w428 -> [w438]
                        i -> [w452]
                        n254 = case shown="0, 默认" w452 {
                          tunnel: [0 7 15 24] -> w451
                          tunnel: [1 8 16 25] -> w450
                          tunnel: [2 9 17 26] -> w449
                          tunnel: [3 10 18 27] -> w448
                          tunnel: [4 11 19 _] -> w447
                          tunnel: [5 12 20 27] -> w446
                          tunnel: [6 13 21 _] -> w445
                          tunnel: [w456 w464 22 _] -> w437
                          tunnel: [w456 w464 23 _] -> w436
                          frame 0, Default {
                            w456 = 0
                          }
                          frame 1 {
                            w464 = 14
                          }
                          frame 2 {
                          }
                          frame 3 {
                          }
                        }
                        n255 = global write "EV05全局变量1.vi" "写入超时"(TRUE ("写入超时")) -> ()
                        n256 = Index Array(array=w455, index #1=w451, index #2=w450, index #3=w449, index #4=w448, index #5=w447, index #6=w446, index #7=w445, index #8=w437, index #9=w436) -> (element #1=w454:u8, element #2=w453:u8, element #3=w444:u8, element #4=w443:u8, element #5=w442:u8, element #6=w441:u8, element #7=w440:u8, element #8=w439:u8, element #9=w435:u8)
                        n257 = case shown="0, 默认" w452 {
                          tunnel: w454 -> [w528 w572 w619 w645]
                          tunnel: w453 -> [w525 w571 w618 w651]
                          tunnel: w444 -> [w524 w569 w617 w648]
                          tunnel: w443 -> [w523 w568 w616 w647]
                          tunnel: w442 -> [w519 w567 w582 _]
                          tunnel: w441 -> [w518 w566 w609 _]
                          tunnel: w440 -> [w496 w565 w608 _]
                          tunnel: w439 -> [_ w564 w607 _]
                          tunnel: w438 -> [w514 w558 w612 w652]
                          tunnel: w435 -> [_ _ w606 _]
                          frame 0, Default {
                            n258 = global read "读配置文件全局.vi" "一级故障"() -> (w513:sgl[])
                            n259 = Join Numbers(hi=w528, lo=w525) -> ((hi.lo)=w527:u16)
                            n260 = Join Numbers(hi=w524, lo=w523) -> ((hi.lo)=w522:u16)
                            n261 = call "输出分辨率计算.vi"("偏移量"=sgl -40.0, "分辨率"=1.0, "数值 3"=w518, "数值 2"=w519) -> ("输出3"=w505:dbl, "输出2"=w507:dbl)  [unwired: 2 in, 4 out]
                            n262 = call "输出分辨率计算.vi"("分辨率"=0.1, "数值 3"=w522, "数值 2"=w527) -> ("输出3"=w509:dbl, "输出2"=w511:dbl)  [unwired: 3 in, 4 out]
                            n263 = Index Array(array=w513, index #5=6 ("索引")) -> (element #1=w510:sgl, element #2=w508:sgl, element #3=w506:sgl, element #4=w504:sgl, element #5=w503:sgl)  [unwired: 4 in]
                            n264 = To Single Precision Float(number=w511) -> (single precision float=w487:sgl)
                            n265 = To Single Precision Float(number=w510) -> (single precision float=w488:sgl)
                            n266 = To Single Precision Float(number=w509) -> (single precision float=w489:sgl)
                            n267 = To Single Precision Float(number=w508) -> (single precision float=w490:sgl)
                            n268 = To Single Precision Float(number=w507) -> (single precision float=w491:sgl)
                            n269 = To Single Precision Float(number=w506) -> (single precision float=w492:sgl)
                            n270 = To Single Precision Float(number=w505) -> (single precision float=w493:sgl)
                            n271 = To Single Precision Float(number=w504) -> (single precision float=w494:sgl)
                            n272 = To Single Precision Float(number=w496) -> (single precision float=w486:sgl)
                            n273 = To Single Precision Float(number=w503) -> (single precision float=w495:sgl)
                            n274 = property class="Clust (严格)"(reference=w514) -> (reference out=w516:refnum<vi>, "Value"=w517:T5)  [unwired: 1 in, 1 out]
                            n275 = Bundle By Name(cluster=w517, "总电压过高"=w511, "总电压过低"=w509, "温度过高"=w507, "温度过低"=w505, "整组温度不均衡"=w496) -> (w515:T5)
                            n276 = Equal?(x=w487, y=w488) -> (x = y?=w502:bool)
                            n277 = Equal?(x=w489, y=w490) -> (x = y?=w501:bool)
                            n278 = Equal?(x=w491, y=w492) -> (x = y?=w500:bool)
                            n279 = Equal?(x=w493, y=w494) -> (x = y?=w499:bool)
                            n280 = Equal?(x=w486, y=w495) -> (x = y?=w498:bool)
                            n281 = Compound Arithmetic op=AND(w502, w501, w500, w499, w498) -> (→"一级故障1":bool)
                            n282 = property class="Clust (严格)"(reference=w516, "Value"=w515) -> ()  [unwired: 1 in, 2 out]
                          }
                          frame 1 {
                            n283 = Join Numbers(hi=w572, lo=w571) -> ((hi.lo)=w557:u16)
                            n284 = Join Numbers(hi=w569, lo=w568) -> ((hi.lo)=w556:u16)
                            n285 = Join Numbers(hi=w567, lo=w566) -> ((hi.lo)=w563:u16)
                            n286 = Join Numbers(hi=w565, lo=w564) -> ((hi.lo)=w562:u16)
                            n287 = global read "读配置文件全局.vi" "一级故障"() -> (w554:sgl[])
                            n288 = call "输出分辨率计算.vi"("分辨率"=0.001, "数值 3"=w562, "数值 2"=w563) -> ("输出3"=w538:dbl, "输出2"=w539:dbl)  [unwired: 3 in, 4 out]
                            n289 = call "输出分辨率计算.vi"("分辨率"=0.001, "数值 3"=w556, "数值 2"=w557) -> ("输出3"=w540:dbl, "输出2"=w541:dbl)  [unwired: 3 in, 4 out]
                            n290 = Index Array(array=w554, index #1=4 ("索引"), index #2=5 ("索引"), index #3=8 ("索引"), index #4=9 ("索引")) -> (element #1=w553:sgl, element #2=w552:sgl, element #3=w551:sgl, element #4=w550:sgl)
                            n291 = property class="Clust (严格)"(reference=w558) -> (reference out=w560:refnum<vi>, "Value"=w561:T5)  [unwired: 1 in, 1 out]
                            n292 = Bundle By Name(cluster=w561, "单组电压不均衡"=w541, "整组电压不均衡"=w540, "单体电压过高"=w539, "单体电压过低"=w538) -> (w559:T5)
                            n293 = To Single Precision Float(number=w539) -> (single precision float=w533:sgl)
                            n294 = To Single Precision Float(number=w538) -> (single precision float=w535:sgl)
                            n295 = To Single Precision Float(number=w551) -> (single precision float=w534:sgl)
                            n296 = To Single Precision Float(number=w550) -> (single precision float=w536:sgl)
                            n297 = To Single Precision Float(number=w552) -> (single precision float=w532:sgl)
                            n298 = To Single Precision Float(number=w540) -> (single precision float=w531:sgl)
                            n299 = To Single Precision Float(number=w541) -> (single precision float=w529:sgl)
                            n300 = To Single Precision Float(number=w553) -> (single precision float=w530:sgl)
                            n301 = property class="Clust (严格)"(reference=w560, "Value"=w559) -> ()  [unwired: 1 in, 2 out]
                            n302 = Equal?(x=w529, y=w530) -> (x = y?=w549:bool)
                            n303 = Equal?(x=w531, y=w532) -> (x = y?=w548:bool)
                            n304 = Equal?(x=w533, y=w534) -> (x = y?=w547:bool)
                            n305 = Equal?(x=w535, y=w536) -> (x = y?=w546:bool)
                            n306 = Compound Arithmetic op=AND(w549, w548, w547, w546) -> (→"一级故障1 2":bool)
                          }
                          frame 2 {
                            n307 = Join Numbers(hi=w619, lo=w618) -> ((hi.lo)=w611:u16)
                            n308 = Join Numbers(hi=w617, lo=w616) -> ((hi.lo)=w610:u16)
                            n309 = global read "读配置文件全局.vi" "一级故障"() -> (w603:sgl[])
                            n310 = Join Numbers(hi=w609, lo=w608) -> ((hi.lo)=w605:u16)
                            n311 = Join Numbers(hi=w607, lo=w606) -> ((hi.lo)=w604:u16)
                            n312 = Index Array(array=w603, index #1=10 ("索引"), index #2=11 ("索引"), index #3=7 ("索引"), index #4=12 ("索引"), index #5=13 ("索引")) -> (element #1=w602:sgl, element #2=w601:sgl, element #3=w600:sgl, element #4=w599:sgl, element #5=w586:sgl)
                            n313 = call "输出分辨率计算.vi"("偏移量"=sgl 0.0, "数值1"=w611, "分辨率"=0.1, "数值 4"=w604, "数值 3"=w605, "数值 2"=w610) -> ("输出4"=w585:dbl, "输出3"=w587:dbl, "输出2"=w588:dbl, "输出1"=w589:dbl)  [unwired: 2 out]
                            n314 = To Single Precision Float(number=w586) -> (single precision float=w581:sgl)
                            n315 = To Single Precision Float(number=w599) -> (single precision float=w579:sgl)
                            n316 = To Single Precision Float(number=w585) -> (single precision float=w580:sgl)
                            n317 = To Single Precision Float(number=w587) -> (single precision float=w578:sgl)
                            n318 = To Single Precision Float(number=w600) -> (single precision float=w577:sgl)
                            n319 = To Single Precision Float(number=w601) -> (single precision float=w576:sgl)
                            n320 = To Single Precision Float(number=w602) -> (single precision float=w574:sgl)
                            n321 = To Single Precision Float(number=w588) -> (single precision float=w575:sgl)
                            n322 = To Single Precision Float(number=w589) -> (single precision float=w573:sgl)
                            n323 = property class="Clust (严格)"(reference=w612) -> (reference out=w614:refnum<vi>, "Value"=w615:T5)  [unwired: 1 in, 1 out]
                            n324 = Bundle By Name(cluster=w615, "充电电流过高"=w589, "放电电流过高"=w588, "单组温度不均衡"=w582, "SOC过高"=w587, "SOC过低"=w585) -> (w613:T5)
                            n325 = Equal?(x=w573, y=w574) -> (x = y?=w598:bool)
                            n326 = Equal?(x=w575, y=w576) -> (x = y?=w597:bool)
                            n327 = Equal?(x=w582, y=w577) -> (x = y?=w596:bool)
                            n328 = Equal?(x=w578, y=w579) -> (x = y?=w595:bool)
                            n329 = Equal?(x=w581, y=w580) -> (x = y?=w584:bool)
                            n330 = property class="Clust (严格)"(reference=w614, "Value"=w613) -> ()  [unwired: 1 in, 2 out]
                            n331 = Compound Arithmetic op=AND(w598, w597, w596, w595, w584) -> (→"一级故障5":bool)
                          }
                          frame 3 {
                            n332 = Join Numbers(hi=w648, lo=w647) -> ((hi.lo)=w646:u16)
                            n333 = global read "读配置文件全局.vi" "一级故障"() -> (w644:sgl[])
                            n334 = local read "一级故障1 2"() -> (w630:bool)
                            n335 = local read "一级故障1"() -> (w631:bool)
                            n336 = local read "一级故障5"() -> (w629:bool)
                            n337 = Index Array(array=w644, index #1=14 ("索引"), index #2=15 ("索引"), index #3=16 ("索引")) -> (element #1=w640:sgl, element #2=w639:sgl, element #3=w638:sgl)
                            n338 = call "输出分辨率计算.vi"("偏移量"=sgl -40.0, "分辨率"=1.0, "数值 3"=w651) -> ("输出3"=w636:dbl)  [unwired: 3 in, 5 out]
                            n339 = call "输出分辨率计算.vi"("数值1"=w645, "分辨率"=0.1, "数值 2"=w646) -> ("输出2"=w635:dbl, "输出1"=w637:dbl)  [unwired: 3 in, 4 out]
                            n340 = To Single Precision Float(number=w635) -> (single precision float=w627:sgl)
                            n341 = To Single Precision Float(number=w638) -> (single precision float=w626:sgl)
                            n342 = To Single Precision Float(number=w636) -> (single precision float=w625:sgl)
                            n343 = To Single Precision Float(number=w639) -> (single precision float=w624:sgl)
                            n344 = To Single Precision Float(number=w637) -> (single precision float=w623:sgl)
                            n345 = To Single Precision Float(number=w640) -> (single precision float=w622:sgl)
                            n346 = property class="Clust (严格)"(reference=w652) -> (reference out=w654:refnum<vi>, "Value"=w655:T5)  [unwired: 1 in, 1 out]
                            n347 = Equal?(x=w622, y=w623) -> (x = y?=w634:bool)
                            n348 = Equal?(x=w624, y=w625) -> (x = y?=w633:bool)
                            n349 = Equal?(x=w626, y=w627) -> (x = y?=w632:bool)
                            n350 = Bundle By Name(cluster=w655, "内阻过大"=w637, "极柱温度过高"=w636, "SOH过低"=w635) -> (w653:T5)
                            n351 = Compound Arithmetic op=AND(w634, w633, w632, w631, w630, w629) -> (w628:bool)
                            n352 = property class="Clust (严格)"(reference=w654, "Value"=w653) -> ()  [unwired: 1 in, 2 out]
                            n353 = global write "读配置文件全局.vi" "一级故障判定"(w628) -> ()
                          }
                        }
                      }
                      n354 = Build Array("一级故障阀值     读取成功" ("字符串")) -> (w427:string[])
                      n355 = call "表格编辑.vi"("新元素/子数组"=w427, "活动单元格:单元格背景色"=u32 6618880, "MCListbox引用句柄"=w424) -> ()  [unwired: 9 out]
                      n356 = global write "EV05全局变量1.vi" "写入超时"(w423) -> ()
                    }
                    frame 2 {
                      w657 = TRUE ("写入超时")
                      n357 = Unbundle By Name(w663) -> ("一级故障 2"=w662:refnum<vi>)
                      n358 = Reshape Array(w667, 28 ("维数大小")) -> (w664:u8[])
                      n359 = for {
                        N: 4 -> [_]
                        tunnel: w664 -> [w689]
                        tunnel: w662 -> [w671]
                        i -> [w686]
                        n360 = case shown="2" w686 {
                          tunnel: [0 7 15 24] -> w685
                          tunnel: [1 8 16 25] -> w684
                          tunnel: [2 9 17 26] -> w683
                          tunnel: [3 10 18 27] -> w682
                          tunnel: [4 11 19 _] -> w681
                          tunnel: [5 12 20 _] -> w680
                          tunnel: [6 13 21 _] -> w679
                          tunnel: [0 14 22 _] -> w678
                          tunnel: [_ _ 23 _] -> w670
                          frame 0, Default {
                          }
                          frame 1 {
                          }
                          frame 2 {
                          }
                          frame 3 {
                          }
                        }
                        n361 = global write "EV05全局变量1.vi" "写入超时"(TRUE ("写入超时")) -> ()
                        n362 = Index Array(array=w689, index #1=w685, index #2=w684, index #3=w683, index #4=w682, index #5=w681, index #6=w680, index #7=w679, index #8=w678, index #9=w670) -> (element #1=w688:u8, element #2=w687:u8, element #3=w677:u8, element #4=w676:u8, element #5=w675:u8, element #6=w674:u8, element #7=w673:u8, element #8=w672:u8, element #9=w669:u8)
                        n363 = case shown="2" w686 {
                          tunnel: w688 -> [w760 w804 w851 w877]
                          tunnel: w687 -> [w757 w803 w850 w883]
                          tunnel: w677 -> [w756 w801 w849 w879]
                          tunnel: w676 -> [w755 w800 w848 w880]
                          tunnel: w675 -> [w751 w799 w814 _]
                          tunnel: w674 -> [w750 w798 w841 _]
                          tunnel: w673 -> [w729 w797 w840 _]
                          tunnel: w672 -> [_ w796 w839 _]
                          tunnel: w671 -> [w746 w790 w844 w884]
                          tunnel: w669 -> [_ _ w838 _]
                          frame 0, Default {
                            n364 = global read "读配置文件全局.vi" "二级故障"() -> (w745:sgl[])
                            n365 = Join Numbers(hi=w760, lo=w757) -> ((hi.lo)=w759:u16)
                            n366 = Join Numbers(hi=w756, lo=w755) -> ((hi.lo)=w754:u16)
                            n367 = call "输出分辨率计算.vi"("偏移量"=sgl -40.0, "分辨率"=1.0, "数值 3"=w750, "数值 2"=w751) -> ("输出3"=w730:dbl, "输出2"=w731:dbl)  [unwired: 2 in, 4 out]
                            n368 = call "输出分辨率计算.vi"("分辨率"=0.1, "数值 3"=w754, "数值 2"=w759) -> ("输出3"=w732:dbl, "输出2"=w733:dbl)  [unwired: 3 in, 4 out]
                            n369 = Index Array(array=w745, index #5=6 ("索引")) -> (element #1=w743:sgl, element #2=w742:sgl, element #3=w741:sgl, element #4=w740:sgl, element #5=w720:sgl)  [unwired: 4 in]
                            n370 = To Single Precision Float(number=w729) -> (single precision float=w719:sgl)
                            n371 = To Single Precision Float(number=w740) -> (single precision float=w728:sgl)
                            n372 = To Single Precision Float(number=w741) -> (single precision float=w726:sgl)
                            n373 = To Single Precision Float(number=w731) -> (single precision float=w725:sgl)
                            n374 = To Single Precision Float(number=w743) -> (single precision float=w722:sgl)
                            n375 = To Single Precision Float(number=w730) -> (single precision float=w727:sgl)
                            n376 = To Single Precision Float(number=w732) -> (single precision float=w723:sgl)
                            n377 = To Single Precision Float(number=w742) -> (single precision float=w724:sgl)
                            n378 = To Single Precision Float(number=w733) -> (single precision float=w721:sgl)
                            n379 = property class="Clust (严格)"(reference=w746) -> (reference out=w748:refnum<vi>, "Value"=w749:T5)  [unwired: 1 in, 1 out]
                            n380 = Bundle By Name(cluster=w749, "总电压过高"=w733, "总电压过低"=w732, "温度过高"=w731, "温度过低"=w730, "整组温度不均衡"=w729) -> (w747:T5)
                            n381 = Equal?(x=w721, y=w722) -> (x = y?=w739:bool)
                            n382 = Equal?(x=w723, y=w724) -> (x = y?=w738:bool)
                            n383 = Equal?(x=w725, y=w726) -> (x = y?=w737:bool)
                            n384 = Equal?(x=w727, y=w728) -> (x = y?=w736:bool)
                            n385 = Equal?(x=w719, y=w720) -> (x = y?=w735:bool)
                            n386 = property class="Clust (严格)"(reference=w748, "Value"=w747) -> ()  [unwired: 1 in, 2 out]
                            n387 = Compound Arithmetic op=AND(w739, w738, w737, w736, w735) -> (→"一级故障1 3":bool)
                          }
                          frame 1 {
                            n388 = global read "读配置文件全局.vi" "二级故障"() -> (w786:sgl[])
                            n389 = Join Numbers(hi=w804, lo=w803) -> ((hi.lo)=w789:u16)
                            n390 = Join Numbers(hi=w801, lo=w800) -> ((hi.lo)=w788:u16)
                            n391 = Join Numbers(hi=w799, lo=w798) -> ((hi.lo)=w795:u16)
                            n392 = Join Numbers(hi=w797, lo=w796) -> ((hi.lo)=w794:u16)
                            n393 = call "输出分辨率计算.vi"("分辨率"=0.001, "数值 3"=w794, "数值 2"=w795) -> ("输出3"=w771:dbl, "输出2"=w774:dbl)  [unwired: 3 in, 4 out]
                            n394 = call "输出分辨率计算.vi"("分辨率"=0.001, "数值 3"=w788, "数值 2"=w789) -> ("输出3"=w775:dbl, "输出2"=w776:dbl)  [unwired: 3 in, 4 out]
                            n395 = Index Array(array=w786, index #1=4 ("索引"), index #2=5 ("索引"), index #3=8 ("索引"), index #4=9 ("索引")) -> (element #1=w785:sgl, element #2=w784:sgl, element #3=w767:sgl, element #4=w770:sgl)
                            n396 = To Single Precision Float(number=w785) -> (single precision float=w763:sgl)
                            n397 = To Single Precision Float(number=w784) -> (single precision float=w764:sgl)
                            n398 = To Single Precision Float(number=w770) -> (single precision float=w768:sgl)
                            n399 = To Single Precision Float(number=w771) -> (single precision float=w769:sgl)
                            n400 = To Single Precision Float(number=w767) -> (single precision float=w765:sgl)
                            n401 = To Single Precision Float(number=w774) -> (single precision float=w766:sgl)
                            n402 = To Single Precision Float(number=w775) -> (single precision float=w762:sgl)
                            n403 = To Single Precision Float(number=w776) -> (single precision float=w761:sgl)
                            n404 = property class="Clust (严格)"(reference=w790) -> (reference out=w792:refnum<vi>, "Value"=w793:T5)  [unwired: 1 in, 1 out]
                            n405 = Bundle By Name(cluster=w793, "单组电压不均衡"=w776, "整组电压不均衡"=w775, "单体电压过高"=w774, "单体电压过低"=w771) -> (w791:T5)
                            n406 = Equal?(x=w761, y=w763) -> (x = y?=w783:bool)
                            n407 = Equal?(x=w762, y=w764) -> (x = y?=w782:bool)
                            n408 = Equal?(x=w766, y=w765) -> (x = y?=w773:bool)
                            n409 = Equal?(x=w769, y=w768) -> (x = y?=w772:bool)
                            n410 = property class="Clust (严格)"(reference=w792, "Value"=w791) -> ()  [unwired: 1 in, 2 out]
                            n411 = Compound Arithmetic op=AND(w783, w782, w773, w772) -> (→"一级故障1 4":bool)
                          }
                          frame 2 {
                            n412 = global read "读配置文件全局.vi" "二级故障"() -> (w835:sgl[])
                            n413 = Join Numbers(hi=w851, lo=w850) -> ((hi.lo)=w843:u16)
                            n414 = Join Numbers(hi=w849, lo=w848) -> ((hi.lo)=w842:u16)
                            n415 = Join Numbers(hi=w841, lo=w840) -> ((hi.lo)=w836:u16)
                            n416 = Join Numbers(hi=w839, lo=w838) -> ((hi.lo)=w837:u16)
                            n417 = Index Array(array=w835, index #1=10 ("索引"), index #2=11 ("索引"), index #3=7 ("索引"), index #4=12 ("索引"), index #5=13 ("索引")) -> (element #1=w834:sgl, element #2=w833:sgl, element #3=w832:sgl, element #4=w831:sgl, element #5=w821:sgl)
                            n418 = call "输出分辨率计算.vi"("偏移量"=sgl 0.0, "数值1"=w843, "分辨率"=0.1, "数值 4"=w837, "数值 3"=w836, "数值 2"=w842) -> ("输出4"=w817:dbl, "输出3"=w818:dbl, "输出2"=w819:dbl, "输出1"=w820:dbl)  [unwired: 2 out]
                            n419 = To Single Precision Float(number=w817) -> (single precision float=w813:sgl)
                            n420 = To Single Precision Float(number=w821) -> (single precision float=w812:sgl)
                            n421 = To Single Precision Float(number=w820) -> (single precision float=w805:sgl)
                            n422 = To Single Precision Float(number=w818) -> (single precision float=w810:sgl)
                            n423 = To Single Precision Float(number=w831) -> (single precision float=w811:sgl)
                            n424 = To Single Precision Float(number=w834) -> (single precision float=w806:sgl)
                            n425 = To Single Precision Float(number=w819) -> (single precision float=w807:sgl)
                            n426 = To Single Precision Float(number=w833) -> (single precision float=w808:sgl)
                            n427 = To Single Precision Float(number=w832) -> (single precision float=w809:sgl)
                            n428 = property class="Clust (严格)"(reference=w844) -> (reference out=w846:refnum<vi>, "Value"=w847:T5)  [unwired: 1 in, 1 out]
                            n429 = Bundle By Name(cluster=w847, "充电电流过高"=w820, "放电电流过高"=w819, "单组温度不均衡"=w814, "SOC过高"=w818, "SOC过低"=w817) -> (w845:T5)
                            n430 = Equal?(x=w805, y=w806) -> (x = y?=w830:bool)
                            n431 = Equal?(x=w807, y=w808) -> (x = y?=w829:bool)
                            n432 = Equal?(x=w814, y=w809) -> (x = y?=w828:bool)
                            n433 = Equal?(x=w810, y=w811) -> (x = y?=w827:bool)
                            n434 = Equal?(x=w812, y=w813) -> (x = y?=w816:bool)
                            n435 = property class="Clust (严格)"(reference=w846, "Value"=w845) -> ()  [unwired: 1 in, 2 out]
                            n436 = Compound Arithmetic op=AND(w830, w829, w828, w827, w816) -> (→"二级故障1":bool)
                          }
                          frame 3 {
                            n437 = Join Numbers(hi=w879, lo=w880) -> ((hi.lo)=w878:u16)
                            n438 = global read "读配置文件全局.vi" "二级故障"() -> (w876:sgl[])
                            n439 = local read "一级故障1 3"() -> (w863:bool)
                            n440 = local read "一级故障1 4"() -> (w862:bool)
                            n441 = local read "二级故障1"() -> (w861:bool)
                            n442 = call "输出分辨率计算.vi"("数值1"=w877, "分辨率"=0.1, "数值 2"=w878) -> ("输出2"=w864:dbl, "输出1"=w866:dbl)  [unwired: 3 in, 4 out]
                            n443 = Index Array(array=w876, index #1=14 ("索引"), index #2=15 ("索引"), index #3=16 ("索引")) -> (element #1=w872:sgl, element #2=w871:sgl, element #3=w870:sgl)
                            n444 = call "输出分辨率计算.vi"("偏移量"=sgl -40.0, "分辨率"=1.0, "数值 3"=w883) -> ("输出3"=w865:dbl)  [unwired: 3 in, 5 out]
                            n445 = To Single Precision Float(number=w870) -> (single precision float=w858:sgl)
                            n446 = To Single Precision Float(number=w865) -> (single precision float=w857:sgl)
                            n447 = To Single Precision Float(number=w871) -> (single precision float=w856:sgl)
                            n448 = To Single Precision Float(number=w864) -> (single precision float=w859:sgl)
                            n449 = To Single Precision Float(number=w872) -> (single precision float=w854:sgl)
                            n450 = To Single Precision Float(number=w866) -> (single precision float=w855:sgl)
                            n451 = Equal?(x=w854, y=w855) -> (x = y?=w869:bool)
                            n452 = Equal?(x=w856, y=w857) -> (x = y?=w868:bool)
                            n453 = Equal?(x=w858, y=w859) -> (x = y?=w867:bool)
                            n454 = property class="Clust (严格)"(reference=w884) -> (reference out=w886:refnum<vi>, "Value"=w887:T5)  [unwired: 1 in, 1 out]
                            n455 = Bundle By Name(cluster=w887, "内阻过大"=w866, "极柱温度过高"=w865, "SOH过低"=w864) -> (w885:T5)
                            n456 = Compound Arithmetic op=AND(w869, w868, w867, w863, w862, w861) -> (w860:bool)
                            n457 = property class="Clust (严格)"(reference=w886, "Value"=w885) -> ()  [unwired: 1 in, 2 out]
                            n458 = global write "读配置文件全局.vi" "二级故障判定"(w860) -> ()
                          }
                        }
                      }
                      n459 = Build Array("二级故障阀值     读取成功" ("字符串")) -> (w661:string[])
                      n460 = call "表格编辑.vi"("新元素/子数组"=w661, "活动单元格:单元格背景色"=u32 6618880, "MCListbox引用句柄"=w659) -> ()  [unwired: 9 out]
                      n461 = global write "EV05全局变量1.vi" "写入超时"(w657) -> ()
                    }
                    frame 3 {
                      w889 = TRUE ("写入超时")
                      n462 = Unbundle By Name(w895) -> ("一级故障 3"=w894:refnum<vi>)
                      n463 = Reshape Array(w899, 28 ("维数大小")) -> (w896:u8[])
                      n464 = for {
                        N: 4 -> [_]
                        tunnel: w896 -> [w920]
                        tunnel: w894 -> [w902]
                        i -> [w917]
                        n465 = case shown="0, 默认" w917 {
                          tunnel: [0 7 15 24] -> w916
                          tunnel: [1 8 16 25] -> w915
                          tunnel: [2 9 17 26] -> w914
                          tunnel: [3 10 18 27] -> w913
                          tunnel: [4 11 19 _] -> w912
                          tunnel: [5 12 20 _] -> w911
                          tunnel: [6 13 21 _] -> w910
                          tunnel: [0 14 22 _] -> w909
                          tunnel: [_ _ 23 _] -> w901
                          frame 0, Default {
                          }
                          frame 1 {
                          }
                          frame 2 {
                          }
                          frame 3 {
                          }
                        }
                        n466 = Index Array(array=w920, index #1=w916, index #2=w915, index #3=w914, index #4=w913, index #5=w912, index #6=w911, index #7=w910, index #8=w909, index #9=w901) -> (element #1=w919:u8, element #2=w918:u8, element #3=w908:u8, element #4=w907:u8, element #5=w906:u8, element #6=w905:u8, element #7=w904:u8, element #8=w903:u8, element #9=w900:u8)
                        n467 = case shown="0, 默认" w917 {
                          tunnel: w919 -> [w992 w1036 w1083 w1109]
                          tunnel: w918 -> [w989 w1035 w1082 w1115]
                          tunnel: w908 -> [w988 w1033 w1081 w1112]
                          tunnel: w907 -> [w987 w1032 w1080 w1111]
                          tunnel: w906 -> [w983 w1031 w1046 _]
                          tunnel: w905 -> [w982 w1030 w1071 _]
                          tunnel: w904 -> [w960 w1029 w1070 _]
                          tunnel: w903 -> [_ w1028 w1073 _]
                          tunnel: w902 -> [w978 w1022 w1076 w1116]
                          tunnel: w900 -> [_ _ w1072 _]
                          frame 0, Default {
                            n468 = global read "读配置文件全局.vi" "三级故障"() -> (w977:sgl[])
                            n469 = Join Numbers(hi=w992, lo=w989) -> ((hi.lo)=w991:u16)
                            n470 = Join Numbers(hi=w988, lo=w987) -> ((hi.lo)=w986:u16)
                            n471 = call "输出分辨率计算.vi"("偏移量"=sgl -40.0, "分辨率"=1.0, "数值 3"=w982, "数值 2"=w983) -> ("输出3"=w962:dbl, "输出2"=w963:dbl)  [unwired: 2 in, 4 out]
                            n472 = call "输出分辨率计算.vi"("分辨率"=0.1, "数值 3"=w986, "数值 2"=w991) -> ("输出3"=w964:dbl, "输出2"=w965:dbl)  [unwired: 3 in, 4 out]
                            n473 = Index Array(array=w977, index #5=6 ("索引")) -> (element #1=w975:sgl, element #2=w974:sgl, element #3=w973:sgl, element #4=w972:sgl, element #5=w961:sgl)  [unwired: 4 in]
                            n474 = To Single Precision Float(number=w962) -> (single precision float=w957:sgl)
                            n475 = To Single Precision Float(number=w972) -> (single precision float=w958:sgl)
                            n476 = To Single Precision Float(number=w965) -> (single precision float=w951:sgl)
                            n477 = To Single Precision Float(number=w973) -> (single precision float=w956:sgl)
                            n478 = To Single Precision Float(number=w960) -> (single precision float=w950:sgl)
                            n479 = To Single Precision Float(number=w974) -> (single precision float=w954:sgl)
                            n480 = To Single Precision Float(number=w963) -> (single precision float=w955:sgl)
                            n481 = To Single Precision Float(number=w961) -> (single precision float=w959:sgl)
                            n482 = To Single Precision Float(number=w975) -> (single precision float=w952:sgl)
                            n483 = To Single Precision Float(number=w964) -> (single precision float=w953:sgl)
                            n484 = property class="Clust (严格)"(reference=w978) -> (reference out=w980:refnum<vi>, "Value"=w981:T5)  [unwired: 1 in, 1 out]
                            n485 = Bundle By Name(cluster=w981, "总电压过高"=w965, "总电压过低"=w964, "温度过高"=w963, "温度过低"=w962, "整组温度不均衡"=w960) -> (w979:T5)
                            n486 = Equal?(x=w951, y=w952) -> (x = y?=w971:bool)
                            n487 = Equal?(x=w953, y=w954) -> (x = y?=w970:bool)
                            n488 = Equal?(x=w955, y=w956) -> (x = y?=w969:bool)
                            n489 = Equal?(x=w957, y=w958) -> (x = y?=w968:bool)
                            n490 = Equal?(x=w950, y=w959) -> (x = y?=w967:bool)
                            n491 = property class="Clust (严格)"(reference=w980, "Value"=w979) -> ()  [unwired: 1 in, 2 out]
                            n492 = Compound Arithmetic op=AND(w971, w970, w969, w968, w967) -> (→"一级故障1 5":bool)
                          }
                          frame 1 {
                            n493 = global read "读配置文件全局.vi" "三级故障"() -> (w1018:sgl[])
                            n494 = Join Numbers(hi=w1036, lo=w1035) -> ((hi.lo)=w1021:u16)
                            n495 = Join Numbers(hi=w1033, lo=w1032) -> ((hi.lo)=w1020:u16)
                            n496 = Join Numbers(hi=w1031, lo=w1030) -> ((hi.lo)=w1027:u16)
                            n497 = Join Numbers(hi=w1029, lo=w1028) -> ((hi.lo)=w1026:u16)
                            n498 = call "输出分辨率计算.vi"("分辨率"=0.001, "数值 3"=w1026, "数值 2"=w1027) -> ("输出3"=w1001:dbl, "输出2"=w1002:dbl)  [unwired: 3 in, 4 out]
                            n499 = call "输出分辨率计算.vi"("分辨率"=0.001, "数值 3"=w1020, "数值 2"=w1021) -> ("输出3"=w1003:dbl, "输出2"=w1004:dbl)  [unwired: 3 in, 4 out]
                            n500 = Index Array(array=w1018, index #1=4 ("索引"), index #2=5 ("索引"), index #3=8 ("索引"), index #4=9 ("索引")) -> (element #1=w1017:sgl, element #2=w1016:sgl, element #3=w1015:sgl, element #4=w1014:sgl)
                            n501 = To Single Precision Float(number=w1015) -> (single precision float=w995:sgl)
                            n502 = To Single Precision Float(number=w1002) -> (single precision float=w996:sgl)
                            n503 = To Single Precision Float(number=w1014) -> (single precision float=w993:sgl)
                            n504 = property class="Clust (严格)"(reference=w1022) -> (reference out=w1024:refnum<vi>, "Value"=w1025:T5)  [unwired: 1 in, 1 out]
                            n505 = Bundle By Name(cluster=w1025, "单组电压不均衡"=w1004, "整组电压不均衡"=w1003, "单体电压过高"=w1002, "单体电压过低"=w1001) -> (w1023:T5)
                            n506 = To Single Precision Float(number=w1001) -> (single precision float=w994:sgl)
                            n507 = To Single Precision Float(number=w1016) -> (single precision float=w997:sgl)
                            n508 = To Single Precision Float(number=w1004) -> (single precision float=w1000:sgl)
                            n509 = To Single Precision Float(number=w1017) -> (single precision float=w999:sgl)
                            n510 = To Single Precision Float(number=w1003) -> (single precision float=w998:sgl)
                            n511 = Equal?(x=w1000, y=w999) -> (x = y?=w1013:bool)
                            n512 = Equal?(x=w998, y=w997) -> (x = y?=w1012:bool)
                            n513 = Equal?(x=w996, y=w995) -> (x = y?=w1011:bool)
                            n514 = Equal?(x=w994, y=w993) -> (x = y?=w1010:bool)
                            n515 = property class="Clust (严格)"(reference=w1024, "Value"=w1023) -> ()  [unwired: 1 in, 2 out]
                            n516 = Compound Arithmetic op=AND(w1013, w1012, w1011, w1010) -> (→"一级故障1 6":bool)
                          }
                          frame 2 {
                            n517 = Join Numbers(hi=w1083, lo=w1082) -> ((hi.lo)=w1075:u16)
                            n518 = Join Numbers(hi=w1081, lo=w1080) -> ((hi.lo)=w1074:u16)
                            n519 = Join Numbers(hi=w1071, lo=w1070) -> ((hi.lo)=w1069:u16)
                            n520 = Join Numbers(hi=w1073, lo=w1072) -> ((hi.lo)=w1068:u16)
                            n521 = global read "读配置文件全局.vi" "三级故障"() -> (w1067:sgl[])
                            n522 = Index Array(array=w1067, index #1=10 ("索引"), index #2=11 ("索引"), index #3=7 ("索引"), index #4=12 ("索引"), index #5=13 ("索引")) -> (element #1=w1066:sgl, element #2=w1065:sgl, element #3=w1064:sgl, element #4=w1063:sgl, element #5=w1053:sgl)
                            n523 = call "输出分辨率计算.vi"("偏移量"=sgl 0.0, "数值1"=w1075, "分辨率"=0.1, "数值 4"=w1068, "数值 3"=w1069, "数值 2"=w1074) -> ("输出4"=w1047:dbl, "输出3"=w1048:dbl, "输出2"=w1049:dbl, "输出1"=w1050:dbl)  [unwired: 2 out]
                            n524 = To Single Precision Float(number=w1063) -> (single precision float=w1043:sgl)
                            n525 = To Single Precision Float(number=w1053) -> (single precision float=w1045:sgl)
                            n526 = To Single Precision Float(number=w1064) -> (single precision float=w1041:sgl)
                            n527 = To Single Precision Float(number=w1065) -> (single precision float=w1040:sgl)
                            n528 = To Single Precision Float(number=w1048) -> (single precision float=w1042:sgl)
                            n529 = To Single Precision Float(number=w1047) -> (single precision float=w1044:sgl)
                            n530 = To Single Precision Float(number=w1049) -> (single precision float=w1039:sgl)
                            n531 = To Single Precision Float(number=w1066) -> (single precision float=w1038:sgl)
                            n532 = To Single Precision Float(number=w1050) -> (single precision float=w1037:sgl)
                            n533 = Equal?(x=w1037, y=w1038) -> (x = y?=w1062:bool)
                            n534 = Equal?(x=w1039, y=w1040) -> (x = y?=w1061:bool)
                            n535 = Equal?(x=w1046, y=w1041) -> (x = y?=w1060:bool)
                            n536 = Equal?(x=w1042, y=w1043) -> (x = y?=w1059:bool)
                            n537 = Equal?(x=w1045, y=w1044) -> (x = y?=w1052:bool)
                            n538 = property class="Clust (严格)"(reference=w1076) -> (reference out=w1078:refnum<vi>, "Value"=w1079:T5)  [unwired: 1 in, 1 out]
                            n539 = Bundle By Name(cluster=w1079, "充电电流过高"=w1050, "放电电流过高"=w1049, "单组温度不均衡"=w1046, "SOC过高"=w1048, "SOC过低"=w1047) -> (w1077:T5)
                            n540 = Compound Arithmetic op=AND(w1062, w1061, w1060, w1059, w1052) -> (→"二级故障1 2":bool)
                            n541 = property class="Clust (严格)"(reference=w1078, "Value"=w1077) -> ()  [unwired: 1 in, 2 out]
                          }
                          frame 3 {
                            n542 = global read "读配置文件全局.vi" "三级故障"() -> (w1108:sgl[])
                            n543 = local read "二级故障1 2"() -> (w1092:bool)
                            n544 = local read "一级故障1 5"() -> (w1094:bool)
                            n545 = local read "一级故障1 6"() -> (w1093:bool)
                            n546 = Join Numbers(hi=w1112, lo=w1111) -> ((hi.lo)=w1110:u16)
                            n547 = Index Array(array=w1108, index #1=14 ("索引"), index #2=15 ("索引"), index #3=16 ("索引")) -> (element #1=w1104:sgl, element #2=w1103:sgl, element #3=w1097:sgl)
                            n548 = call "输出分辨率计算.vi"("偏移量"=sgl -40.0, "分辨率"=1.0, "数值 3"=w1115) -> ("输出3"=w1098:dbl)  [unwired: 3 in, 5 out]
                            n549 = call "输出分辨率计算.vi"("数值1"=w1109, "分辨率"=0.1, "数值 2"=w1110) -> ("输出2"=w1096:dbl, "输出1"=w1099:dbl)  [unwired: 3 in, 4 out]
                            n550 = To Single Precision Float(number=w1103) -> (single precision float=w1089:sgl)
                            n551 = To Single Precision Float(number=w1098) -> (single precision float=w1088:sgl)
                            n552 = To Single Precision Float(number=w1097) -> (single precision float=w1087:sgl)
                            n553 = To Single Precision Float(number=w1096) -> (single precision float=w1086:sgl)
                            n554 = To Single Precision Float(number=w1099) -> (single precision float=w1090:sgl)
                            n555 = To Single Precision Float(number=w1104) -> (single precision float=w1091:sgl)
                            n556 = Equal?(x=w1091, y=w1090) -> (x = y?=w1102:bool)
                            n557 = Equal?(x=w1089, y=w1088) -> (x = y?=w1101:bool)
                            n558 = Equal?(x=w1087, y=w1086) -> (x = y?=w1100:bool)
                            n559 = property class="Clust (严格)"(reference=w1116) -> (reference out=w1118:refnum<vi>, "Value"=w1119:T5)  [unwired: 1 in, 1 out]
                            n560 = Bundle By Name(cluster=w1119, "内阻过大"=w1099, "极柱温度过高"=w1098, "SOH过低"=w1096) -> (w1117:T5)
                            n561 = Compound Arithmetic op=AND(w1102, w1101, w1100, w1094, w1093, w1092) -> (w1095:bool)
                            n562 = property class="Clust (严格)"(reference=w1118, "Value"=w1117) -> ()  [unwired: 1 in, 2 out]
                            n563 = global write "读配置文件全局.vi" "三级故障判定"(w1095) -> ()
                          }
                        }
                      }
                      n564 = Build Array("三级故障阀值     读取成功" ("字符串")) -> (w891:string[])
                      n565 = call "表格编辑.vi"("新元素/子数组"=w891, "活动单元格:单元格背景色"=u32 6618880, "MCListbox引用句柄"=w890) -> ()  [unwired: 9 out]
                      n566 = global write "EV05全局变量1.vi" "写入超时"(w889) -> ()
                    }
                  }
                }
                frame 130 {
                  n567 = case shown="0, 默认" w1125 {
                    tunnel: w1124 -> [_ w1167 w1178]
                    tunnel: w1123 -> [_ w1162 w1174]
                    tunnel: w1122 -> [_ w1152 w1170]
                    tunnel: [_ w1126 w1168] -> w1121
                    frame 0, Default {
                    }
                    frame 1 {
                      w1126 = TRUE ("写入超时")
                      n568 = Unbundle By Name(w1162) -> ("加热控制参数"=w1161:refnum<vi>)
                      n569 = global read "读配置文件全局.vi" "加热控制参数"() -> (w1151:dbl[])
                      n570 = Reshape Array(w1167, 7 ("维数大小")) -> (w1158:u8[])
                      n571 = Index Array(array=w1158) -> (element #1=w1157:u8, element #2=w1156:u8, element #3=w1131:u8, element #4=w1130:u8, element #5=w1133:u8, element #6=w1132:u8, element #7=w1127:u8)  [unwired: 7 in]
                      n572 = Index Array(array=w1151) -> (element #1=w1150:dbl, element #2=w1149:dbl, element #3=w1148:dbl, element #4=w1147:dbl, element #5=w1141:dbl, element #6=w1146:dbl, element #7=w1129:dbl)  [unwired: 7 in]
                      n573 = call "输出分辨率计算.vi"("偏移量"=sgl -40.0, "数值1"=w1157, "分辨率"=1.0, "数值 4"=w1132, "数值 3"=w1133, "数值 2"=w1156) -> ("输出4"=w1142:dbl, "输出3"=w1143:dbl, "输出2"=w1144:dbl, "输出1"=w1145:dbl)  [unwired: 2 out]
                      n574 = Equal?(x=w1127, y=w1129) -> (x = y?=w1128:bool)
                      n575 = Equal?(x=w1150, y=w1145) -> (x = y?=w1140:bool)
                      n576 = Equal?(x=w1149, y=w1144) -> (x = y?=w1139:bool)
                      n577 = Equal?(x=w1148, y=w1143) -> (x = y?=w1138:bool)
                      n578 = Equal?(x=w1147, y=w1142) -> (x = y?=w1137:bool)
                      n579 = Equal?(x=w1141, y=w1131) -> (x = y?=w1136:bool)
                      n580 = Equal?(x=w1146, y=w1130) -> (x = y?=w1135:bool)
                      n581 = Build Array("加热控制参数     读取成功" ("字符串")) -> (w1155:string[])
                      n582 = Compound Arithmetic op=AND(w1140, w1139, w1138, w1137, w1136, w1135, w1128) -> (w1134:bool)
                      n583 = global write "读配置文件全局.vi" "加热控制参数判定"(w1134) -> ()
                      n584 = call "表格编辑.vi"("新元素/子数组"=w1155, "活动单元格:单元格背景色"=u32 6618880, "MCListbox引用句柄"=w1152) -> ()  [unwired: 9 out]
                      n585 = property class="Clust (严格)"(reference=w1161) -> (reference out=w1164:refnum<vi>, "Value"=w1165:T6)  [unwired: 1 in, 1 out]
                      n586 = Bundle By Name(cluster=w1165, "风机开启温度"=w1145, "风机关闭温度"=w1144, "加热开启温度"=w1143, "加热关闭温度"=w1142, "风机开启温差"=w1131, "风机关闭温差"=w1130, "加热关闭温差"=w1127) -> (w1163:T6)
                      n587 = global write "EV05全局变量1.vi" "写入超时"(w1126) -> ()
                      n588 = property class="Clust (严格)"(reference=w1164, "Value"=w1163) -> ()  [unwired: 1 in, 2 out]
                    }
                    frame 2 {
                      w1168 = TRUE ("写入超时")
                      n589 = Unbundle By Name(w1174) -> ("充电控制参数"=w1173:refnum<vi>)
                      n590 = Reshape Array(w1178, 14 ("维数大小")) -> (w1175:u8[])
                      n591 = for {
                        N: 2 -> [_]
                        tunnel: w1175 -> [w1195]
                        tunnel: w1173 -> [w1179]
                        i -> [w1187]
                        n592 = case shown="0, 默认" w1187 {
                          tunnel: [0 7 14] -> w1194
                          tunnel: [1 8 15] -> w1193
                          tunnel: [2 9 16] -> w1192
                          tunnel: [3 10 10] -> w1191
                          tunnel: [4 11 11] -> w1190
                          tunnel: [5 12 12] -> w1189
                          tunnel: [6 13 13] -> w1188
                          frame 0, Default {
                          }
                          frame 1 {
                          }
                          frame 2 {
                          }
                        }
                        n593 = Index Array(array=w1195, index #1=w1194, index #2=w1193, index #3=w1192, index #4=w1191, index #5=w1190, index #6=w1189, index #7=w1188) -> (element #1=w1185:u8, element #2=w1186:u8, element #3=w1184:u8, element #4=w1183:u8, element #5=w1182:u8, element #6=w1181:u8, element #7=w1180:u8)
                        n594 = case shown="1" w1187 {
                          tunnel: w1186 -> [w1239 w1285]
                          tunnel: w1185 -> [w1238 w1284]
                          tunnel: w1184 -> [w1237 w1283]
                          tunnel: w1183 -> [w1236 w1282]
                          tunnel: w1182 -> [w1235 w1281]
                          tunnel: w1181 -> [w1234 w1280]
                          tunnel: w1180 -> [w1226 w1274]
                          tunnel: w1179 -> [w1220 w1268]
                          frame 0, Default {
                            n595 = Join Numbers(hi=w1235, lo=w1234) -> ((hi.lo)=w1231:u16)
                            n596 = Join Numbers(hi=w1238, lo=w1239) -> ((hi.lo)=w1233:u16)
                            n597 = Join Numbers(hi=w1237, lo=w1236) -> ((hi.lo)=w1232:u16)
                            n598 = global read "读配置文件全局.vi" "充电控制参数"() -> (w1219:dbl[])
                            n599 = call "输出分辨率计算.vi"("分辨率"=0.1, "数值 2"=w1232) -> ("输出2"=w1211:dbl)  [unwired: 4 in, 5 out]
                            n600 = call "输出分辨率计算.vi"("偏移量"=sgl 0.0, "分辨率"=0.1, "数值 2"=w1231) -> ("输出2"=w1210:dbl)  [unwired: 3 in, 5 out]
                            n601 = call "输出分辨率计算.vi"("分辨率"=0.001, "数值 2"=w1233) -> ("输出2"=w1212:dbl)  [unwired: 4 in, 5 out]
                            n602 = call "输出分辨率计算.vi"("偏移量"=sgl -40.0, "分辨率"=1.0, "数值 2"=w1226) -> ("输出2"=w1209:dbl)  [unwired: 3 in, 5 out]
                            n603 = Index Array(array=w1219, index #3=3 ("索引"), index #4=6 ("索引")) -> (element #1=w1216:dbl, element #2=w1215:dbl, element #3=w1214:dbl, element #4=w1213:dbl)  [unwired: 2 in]
                            n604 = To Single Precision Float(number=w1212) -> (single precision float=w1202:sgl)
                            n605 = To Single Precision Float(number=w1216) -> (single precision float=w1203:sgl)
                            n606 = To Single Precision Float(number=w1213) -> (single precision float=w1197:sgl)
                            n607 = To Single Precision Float(number=w1209) -> (single precision float=w1196:sgl)
                            n608 = To Single Precision Float(number=w1211) -> (single precision float=w1200:sgl)
                            n609 = To Single Precision Float(number=w1210) -> (single precision float=w1198:sgl)
                            n610 = To Single Precision Float(number=w1214) -> (single precision float=w1199:sgl)
                            n611 = To Single Precision Float(number=w1215) -> (single precision float=w1201:sgl)
                            n612 = property class="Clust (严格)"(reference=w1220) -> (reference out=w1222:refnum<vi>, "Value"=w1223:T7)  [unwired: 1 in, 1 out]
                            n613 = Bundle By Name(cluster=w1223, "最大允许单体电压"=w1212, "最大允许总电压"=w1211, "最大允许充电电流"=w1210, "最小允许充电温度"=w1209) -> (w1221:T7)
                            n614 = Equal?(x=w1203, y=w1202) -> (x = y?=w1208:bool)
                            n615 = Equal?(x=w1201, y=w1200) -> (x = y?=w1207:bool)
                            n616 = Equal?(x=w1199, y=w1198) -> (x = y?=w1206:bool)
                            n617 = Equal?(x=w1197, y=w1196) -> (x = y?=w1205:bool)
                            n618 = Compound Arithmetic op=AND(w1208, w1207, w1206, w1205) -> (→"充电控制参数":bool)
                            n619 = property class="Clust (严格)"(reference=w1222, "Value"=w1221) -> ()  [unwired: 1 in, 2 out]
                          }
                          frame 1 {
                            n620 = Join Numbers(hi=w1281, lo=w1280) -> ((hi.lo)=w1278:u16)
                            n621 = Join Numbers(hi=w1284, lo=w1285) -> ((hi.lo)=w1279:u16)
                            n622 = Join Numbers(hi=w1283, lo=w1282) -> ((hi.lo)=w1247:u16)
                            n623 = global read "读配置文件全局.vi" "充电控制参数"() -> (w1267:dbl[])
                            n624 = call "输出分辨率计算.vi"("偏移量"=sgl 0.0, "分辨率"=0.1, "数值 3"=w1247, "数值 2"=w1279) -> ("输出3"=w1246:dbl, "输出2"=w1259:dbl)  [unwired: 2 in, 4 out]
                            n625 = call "输出分辨率计算.vi"("分辨率"=0.001, "数值 2"=w1278) -> ("输出2"=w1252:dbl)  [unwired: 4 in, 5 out]
                            n626 = call "输出分辨率计算.vi"("偏移量"=sgl -40.0, "分辨率"=1.0, "数值 2"=w1274) -> ("输出2"=w1258:dbl)  [unwired: 3 in, 5 out]
                            n627 = Index Array(array=w1267, index #1=4 ("索引"), index #2=7 ("索引"), index #3=2 ("索引"), index #4=5 ("索引")) -> (element #1=w1266:dbl, element #2=w1265:dbl, element #3=w1251:dbl, element #4=w1264:dbl)
                            n628 = local read "充电控制参数"() -> (w1257:bool)
                            n629 = To Single Precision Float(number=w1264) -> (single precision float=w1241:sgl)
                            n630 = To Single Precision Float(number=w1258) -> (single precision float=w1240:sgl)
                            n631 = To Single Precision Float(number=w1265) -> (single precision float=w1243:sgl)
                            n632 = property class="Clust (严格)"(reference=w1268) -> (reference out=w1270:refnum<vi>, "Value"=w1271:T7)  [unwired: 1 in, 1 out]
                            n633 = Bundle By Name(cluster=w1271, "最小允许充电电流"=w1259, "电流步长"=w1246, "最小允许单体电压"=w1252, "最大允许充电温度"=w1258) -> (w1269:T7)
                            n634 = To Single Precision Float(number=w1246) -> (single precision float=w1242:sgl)
                            n635 = To Single Precision Float(number=w1259) -> (single precision float=w1244:sgl)
                            n636 = To Single Precision Float(number=w1252) -> (single precision float=w1249:sgl)
                            n637 = To Single Precision Float(number=w1266) -> (single precision float=w1245:sgl)
                            n638 = To Single Precision Float(number=w1251) -> (single precision float=w1248:sgl)
                            n639 = Equal?(x=w1241, y=w1240) -> (x = y?=w1254:bool)
                            n640 = Equal?(x=w1245, y=w1244) -> (x = y?=w1256:bool)
                            n641 = Equal?(x=w1243, y=w1242) -> (x = y?=w1255:bool)
                            n642 = Equal?(x=w1249, y=w1248) -> (x = y?=w1250:bool)
                            n643 = property class="Clust (严格)"(reference=w1270, "Value"=w1269) -> ()  [unwired: 1 in, 2 out]
                            n644 = Compound Arithmetic op=AND(w1256, w1255, w1250, w1254, w1257) -> (w1253:bool)
                            n645 = global write "读配置文件全局.vi" "充电控制参数判定"(w1253) -> ()
                          }
                        }
                      }
                      n646 = Build Array("充电控制参数     读取成功" ("字符串")) -> (w1172:string[])
                      n647 = call "表格编辑.vi"("新元素/子数组"=w1172, "活动单元格:单元格背景色"=u32 6618880, "MCListbox引用句柄"=w1170) -> ()  [unwired: 9 out]
                      n648 = global write "EV05全局变量1.vi" "写入超时"(w1168) -> ()
                    }
                  }
                }
                frame 98 {
                  n649 = case shown="0, 默认" w1311 {
                    tunnel: w1310 -> [_ w1332 w1353]
                    tunnel: w1309 -> [_ w1327 w1348]
                    tunnel: w1308 -> [_ w1320 w1341]
                    tunnel: [_ w1312 w1333] -> w1307
                    frame 0, Default {
                    }
                    frame 5 {
                      w1312 = TRUE ("写入超时")
                      n650 = Reshape Array(w1332, 4 ("维数大小")) -> (w1324:u8[])
                      n651 = Unbundle By Name(w1327) -> ("高压参数"=w1326:refnum<vi>)
                      n652 = Index Array(array=w1324) -> (element #1=w1318:u8, element #2=w1319:u8, element #3=w1315:u8, element #4=w1316:u8)  [unwired: 4 in]
                      n653 = Join Numbers(hi=w1315, lo=w1316) -> ((hi.lo)=w1314:u16)
                      n654 = Join Numbers(hi=w1318, lo=w1319) -> ((hi.lo)=w1317:u16)
                      n655 = call "输出分辨率计算.vi"("分辨率"=0.1, "数值 2"=w1314) -> ("输出2"=w1313:dbl)  [unwired: 4 in, 5 out]
                      n656 = Build Array("电流增益     读取成功" ("字符串")) -> (w1323:string[])
                      n657 = call "表格编辑.vi"("新元素/子数组"=w1323, "活动单元格:单元格背景色"=u32 6618880, "MCListbox引用句柄"=w1320) -> ()  [unwired: 9 out]
                      n658 = property class="Clust (严格)"(reference=w1326) -> (reference out=w1329:refnum<vi>, "Value"=w1330:T8)  [unwired: 1 in, 1 out]
                      n659 = Bundle By Name(cluster=w1330, "电流增益"=w1317, "平均电流"=w1313) -> (w1328:T8)
                      n660 = global write "EV05全局变量1.vi" "写入超时"(w1312) -> ()
                      n661 = property class="Clust (严格)"(reference=w1329, "Value"=w1328) -> ()  [unwired: 1 in, 2 out]
                    }
                    frame 6 {
                      w1333 = TRUE ("写入超时")
                      n662 = Reshape Array(w1353, 4 ("维数大小")) -> (w1345:u8[])
                      n663 = Unbundle By Name(w1348) -> ("高压参数"=w1347:refnum<vi>)
                      n664 = Index Array(array=w1345) -> (element #1=w1339:u8, element #2=w1340:u8, element #3=w1336:u8, element #4=w1337:u8)  [unwired: 4 in]
                      n665 = Join Numbers(hi=w1336, lo=w1337) -> ((hi.lo)=w1335:u16)
                      n666 = Join Numbers(hi=w1339, lo=w1340) -> ((hi.lo)=w1338:u16)
                      n667 = call "输出分辨率计算.vi"("分辨率"=0.1, "数值 2"=w1335) -> ("输出2"=w1334:dbl)  [unwired: 4 in, 5 out]
                      n668 = Build Array("电压增益     读取成功" ("字符串")) -> (w1344:string[])
                      n669 = call "表格编辑.vi"("新元素/子数组"=w1344, "活动单元格:单元格背景色"=u32 6618880, "MCListbox引用句柄"=w1341) -> ()  [unwired: 9 out]
                      n670 = property class="Clust (严格)"(reference=w1347) -> (reference out=w1350:refnum<vi>, "Value"=w1351:T8)  [unwired: 1 in, 1 out]
                      n671 = Bundle By Name(cluster=w1351, "电压增益"=w1338, "平均电压"=w1334) -> (w1349:T8)
                      n672 = global write "EV05全局变量1.vi" "写入超时"(w1333) -> ()
                      n673 = property class="Clust (严格)"(reference=w1350, "Value"=w1349) -> ()  [unwired: 1 in, 2 out]
                    }
                  }
                }
                frame 99 {
                  n674 = case shown="0, 默认" w1358 {
                    tunnel: w1357 -> [_ w1378 w1398]
                    tunnel: w1356 -> [_ w1373 w1393]
                    tunnel: w1355 -> [_ w1367 w1387]
                    tunnel: [_ w1359 w1379] -> w1354
                    frame 0, Default {
                    }
                    frame 4 {
                      w1359 = TRUE ("写入超时")
                      n675 = Reshape Array(w1378, 4 ("维数大小")) -> (w1371:u8[])
                      n676 = Unbundle By Name(w1373) -> ("高压参数"=w1372:refnum<vi>)
                      n677 = Index Array(array=w1371) -> (element #1=w1365:u8, element #2=w1366:u8, element #3=w1363:u8, element #4=w1364:u8)  [unwired: 4 in]
                      n678 = Join Numbers(hi=w1363, lo=w1364) -> ((hi.lo)=w1361:u16)
                      n679 = Join Numbers(hi=w1365, lo=w1366) -> ((hi.lo)=w1362:u16)
                      n680 = Join Numbers(hi=w1362, lo=w1361) -> ((hi.lo)=w1360:u32)
                      n681 = Build Array("充电能量阀值     读取成功" ("字符串")) -> (w1370:string[])
                      n682 = call "表格编辑.vi"("新元素/子数组"=w1370, "活动单元格:单元格背景色"=u32 6618880, "MCListbox引用句柄"=w1367) -> ()  [unwired: 9 out]
                      n683 = property class="Clust (严格)"(reference=w1372) -> (reference out=w1375:refnum<vi>, "Value"=w1376:T8)  [unwired: 1 in, 1 out]
                      n684 = Bundle By Name(cluster=w1376, "充电能量阀值"=w1360) -> (w1374:T8)
                      n685 = global write "EV05全局变量1.vi" "写入超时"(w1359) -> ()
                      n686 = property class="Clust (严格)"(reference=w1375, "Value"=w1374) -> ()  [unwired: 1 in, 2 out]
                    }
                    frame 5 {
                      w1379 = TRUE ("写入超时")
                      n687 = Reshape Array(w1398, 4 ("维数大小")) -> (w1391:u8[])
                      n688 = Unbundle By Name(w1393) -> ("高压参数"=w1392:refnum<vi>)
                      n689 = Index Array(array=w1391) -> (element #1=w1385:u8, element #2=w1386:u8, element #3=w1383:u8, element #4=w1384:u8)  [unwired: 4 in]
                      n690 = Join Numbers(hi=w1383, lo=w1384) -> ((hi.lo)=w1381:u16)
                      n691 = Join Numbers(hi=w1385, lo=w1386) -> ((hi.lo)=w1382:u16)
                      n692 = Join Numbers(hi=w1382, lo=w1381) -> ((hi.lo)=w1380:u32)
                      n693 = Build Array("放电能量阀值     读取成功" ("字符串")) -> (w1390:string[])
                      n694 = call "表格编辑.vi"("新元素/子数组"=w1390, "活动单元格:单元格背景色"=u32 6618880, "MCListbox引用句柄"=w1387) -> ()  [unwired: 9 out]
                      n695 = property class="Clust (严格)"(reference=w1392) -> (reference out=w1395:refnum<vi>, "Value"=w1396:T8)  [unwired: 1 in, 1 out]
                      n696 = Bundle By Name(cluster=w1396, "放电能量阀值"=w1380) -> (w1394:T8)
                      n697 = global write "EV05全局变量1.vi" "写入超时"(w1379) -> ()
                      n698 = property class="Clust (严格)"(reference=w1395, "Value"=w1394) -> ()  [unwired: 1 in, 2 out]
                    }
                  }
                }
                frame 131 {
                  n699 = disable-structure shown="禁用" {
                    disable-tunnel: w1400 -> [w1403 _]
                    disable-tunnel: w1399 -> [w1402 _]
                    disable-tunnel: _ -> [w1401 _]
                    frame Disabled {
                      n700 = case shown="2" w1403 {
                        tunnel: w1402 -> [_ w1416 w1460 w1502 w1539]
                        tunnel: w1401 -> [_ w1415 w1459 w1501 w1538]
                        tunnel: _ -> [_ w1411 w1455 w1497 w1534]
                        frame 0, Default {
                        }
                        frame 1 {
                          n701 = Reshape Array(w1416, 14 ("维数大小")) -> (w1405:u8[])
                          n702 = for {
                            N: 7 ("维数大小") -> [_]
                            tunnel: w1415 -> [w1447]
                            tunnel: [w1447] -> w1408 mode=indexing
                          }
                          n703 = for {
                            N: 7 -> [_]
                            tunnel: w1405 -> [w1425]
                            tunnel: [w1417] -> w1404 mode=indexing
                            i -> [w1421]
                            n704 = Multiply(x=w1421, y=2) -> (x*y=w1423:i32)
                            n705 = Increment(x=w1423) -> (x+1=w1422:i32)
                            n706 = Index Array(array=w1425, index #1=w1423, index #2=w1422) -> (element #1=w1420:u8, element #2=w1419:u8)
                            n707 = Join Numbers(hi=w1420, lo=w1419) -> ((hi.lo)=w1418:u16)
                            n708 = case shown="6" w1421 {
                              tunnel: w1418 -> [w1428 w1431 w1434 w1437 w1440 w1443 w1446]
                              tunnel: [w1426 w1429 w1432 w1435 w1438 w1441 w1444] -> w1417
                              frame 0, Default {
                                n709 = call "输出分辨率计算.vi"("分辨率"=0.001, "数值 2"=w1428) -> ("输出2"=w1426:dbl)  [unwired: 4 in, 5 out]
                              }
                              frame 1 {
                                n710 = call "输出分辨率计算.vi"("分辨率"=0.001, "数值 2"=w1431) -> ("输出2"=w1429:dbl)  [unwired: 4 in, 5 out]
                              }
                              frame 2 {
                                n711 = call "输出分辨率计算.vi"("分辨率"=1.0, "数值 2"=w1434) -> ("输出2"=w1432:dbl)  [unwired: 4 in, 5 out]
                              }
                              frame 3 {
                                n712 = call "输出分辨率计算.vi"("分辨率"=0.001, "数值 2"=w1437) -> ("输出2"=w1435:dbl)  [unwired: 4 in, 5 out]
                              }
                              frame 4 {
                                n713 = call "输出分辨率计算.vi"("分辨率"=0.001, "数值 2"=w1440) -> ("输出2"=w1438:dbl)  [unwired: 4 in, 5 out]
                              }
                              frame 5 {
                                n714 = call "输出分辨率计算.vi"("分辨率"=0.1, "数值 2"=w1443) -> ("输出2"=w1441:dbl)  [unwired: 4 in, 5 out]
                              }
                              frame 6 {
                                n715 = call "输出分辨率计算.vi"("分辨率"=0.1, "数值 2"=w1446) -> ("输出2"=w1444:dbl)  [unwired: 4 in, 5 out]
                              }
                            }
                          }
                          n716 = call "表格数据输入(数值)-8.6.vi"("行数"=u32 1, "列数"=u32 17, "数值数组"=w1404, "表格引用"=w1411) -> ()  [unwired: 8 out]
                          n717 = call "表格颜色-8.6.vi"("颜色类型"=w1408, "列数"=17, "行数"=1, "表格引用"=w1411) -> ()  [unwired: 1 in, 7 out]
                        }
                        frame 3 {
                          n718 = Reshape Array(w1460, 12 ("维数大小")) -> (w1449:u8[])
                          n719 = for {
                            N: 6 ("维数大小") -> [_]
                            tunnel: w1459 -> [w1489]
                            tunnel: [w1489] -> w1452 mode=indexing
                          }
                          n720 = for {
                            N: 6 -> [_]
                            tunnel: w1449 -> [w1469]
                            tunnel: [w1461] -> w1448 mode=indexing
                            i -> [w1465]
                            n721 = Multiply(x=w1465, y=2) -> (x*y=w1467:i32)
                            n722 = Increment(x=w1467) -> (x+1=w1466:i32)
                            n723 = Index Array(array=w1469, index #1=w1467, index #2=w1466) -> (element #1=w1464:u8, element #2=w1463:u8)
                            n724 = Join Numbers(hi=w1464, lo=w1463) -> ((hi.lo)=w1462:u16)
                            n725 = case shown="4, 5" w1465 {
                              tunnel: w1462 -> [w1473 w1477 w1481 w1485 w1488]
                              tunnel: [w1471 w1475 w1479 w1483 w1486] -> w1461
                              frame 0, Default {
                                n726 = call "输出分辨率计算.vi"("偏移量"=sgl -300.0, "分辨率"=0.01, "数值 2"=w1473) -> ("输出2"=w1471:dbl)  [unwired: 3 in, 5 out]
                              }
                              frame 1 {
                                n727 = call "输出分辨率计算.vi"("偏移量"=sgl -300.0, "分辨率"=0.01, "数值 2"=w1477) -> ("输出2"=w1475:dbl)  [unwired: 3 in, 5 out]
                              }
                              frame 2 {
                                n728 = call "输出分辨率计算.vi"("偏移量"=sgl -3000.0, "分辨率"=0.1, "数值 2"=w1481) -> ("输出2"=w1479:dbl)  [unwired: 3 in, 5 out]
                              }
                              frame 3 {
                                n729 = call "输出分辨率计算.vi"("偏移量"=sgl -3000.0, "分辨率"=0.1, "数值 2"=w1485) -> ("输出2"=w1483:dbl)  [unwired: 3 in, 5 out]
                              }
                              frame 4, 5 {
                                n730 = call "输出分辨率计算.vi"("分辨率"=1.0, "数值 2"=w1488) -> ("输出2"=w1486:dbl)  [unwired: 4 in, 5 out]
                              }
                            }
                          }
                          n731 = call "表格数据输入(数值)-8.6.vi"("行数"=u32 17, "列数"=u32 17, "数值数组"=w1448, "表格引用"=w1455) -> ()  [unwired: 8 out]
                          n732 = call "表格颜色-8.6.vi"("颜色类型"=w1452, "列数"=17, "行数"=17, "表格引用"=w1455) -> ()  [unwired: 1 in, 7 out]
                        }
                        frame 4 {
                          n733 = Reshape Array(w1502, 12 ("维数大小")) -> (w1491:u8[])
                          n734 = for {
                            N: 3 ("维数大小") -> [_]
                            tunnel: w1501 -> [w1527]
                            tunnel: [w1527] -> w1494 mode=indexing
                          }
                          n735 = for {
                            N: 3 -> [_]
                            tunnel: w1491 -> [w1517]
                            tunnel: [w1511] -> w1490 mode=indexing
                            i -> [w1514]
                            n736 = Multiply(x=w1514, y=4) -> (x*y=w1515:i32)
                            n737 = Increment(x=w1515) -> (x+1=w1510:i32)
                            n738 = Increment(x=w1510) -> (x+1=w1509:i32)
                            n739 = Increment(x=w1509) -> (x+1=w1508:i32)
                            n740 = Index Array(array=w1517, index #1=w1515, index #2=w1510, index #3=w1509, index #4=w1508) -> (element #1=w1513:u8, element #2=w1512:u8, element #3=w1507:u8, element #4=w1506:u8)
                            n741 = Join Numbers(hi=w1513, lo=w1512) -> ((hi.lo)=w1504:u16)
                            n742 = Join Numbers(hi=w1507, lo=w1506) -> ((hi.lo)=w1505:u16)
                            n743 = Join Numbers(hi=w1504, lo=w1505) -> ((hi.lo)=w1503:u32)
                            n744 = case shown="0, 默认" w1514 {
                              tunnel: w1503 -> [w1520 w1523 w1526]
                              tunnel: [w1518 w1521 w1524] -> w1511
                              frame 0, Default {
                                n745 = call "输出分辨率计算.vi"("分辨率"=0.001, "数值 2"=w1520) -> ("输出2"=w1518:dbl)  [unwired: 4 in, 5 out]
                              }
                              frame 1 {
                                n746 = call "输出分辨率计算.vi"("分辨率"=0.001, "数值 2"=w1523) -> ("输出2"=w1521:dbl)  [unwired: 4 in, 5 out]
                              }
                              frame 2 {
                                n747 = call "输出分辨率计算.vi"("分辨率"=0.1, "数值 2"=w1526) -> ("输出2"=w1524:dbl)  [unwired: 4 in, 5 out]
                              }
                            }
                          }
                          n748 = call "表格数据输入(数值)-8.6.vi"("行数"=u32 23, "列数"=u32 17, "数值数组"=w1490, "表格引用"=w1497) -> ()  [unwired: 8 out]
                          n749 = call "表格颜色-8.6.vi"("颜色类型"=w1494, "列数"=17, "行数"=23, "表格引用"=w1497) -> ()  [unwired: 1 in, 7 out]
                        }
                        frame 2 {
                          n750 = Reshape Array(w1539, 9 ("维数大小")) -> (w1529:u8[])
                          n751 = for {
                            N: 9 ("维数大小") -> [_]
                            tunnel: w1538 -> [w1565]
                            tunnel: [w1565] -> w1531 mode=indexing
                          }
                          n752 = for {
                            tunnel: w1529 -> [w1540] mode=indexing
                            tunnel: [w1541] -> w1528 mode=indexing
                            i -> [w1542]
                            n753 = case shown="5..8" w1542 {
                              tunnel: w1540 -> [w1546 w1550 w1553 w1557 w1561 w1564]
                              tunnel: [w1544 w1548 w1551 w1555 w1559 w1562] -> w1541
                              frame 0, Default {
                                n754 = call "输出分辨率计算.vi"("偏移量"=sgl -40.0, "分辨率"=1.0, "数值 2"=w1546) -> ("输出2"=w1544:dbl)  [unwired: 3 in, 5 out]
                              }
                              frame 1 {
                                n755 = call "输出分辨率计算.vi"("偏移量"=sgl -40.0, "分辨率"=1.0, "数值 2"=w1550) -> ("输出2"=w1548:dbl)  [unwired: 3 in, 5 out]
                              }
                              frame 2 {
                                n756 = call "输出分辨率计算.vi"("分辨率"=1.0, "数值 2"=w1553) -> ("输出2"=w1551:dbl)  [unwired: 4 in, 5 out]
                              }
                              frame 3 {
                                n757 = call "输出分辨率计算.vi"("偏移量"=sgl -40.0, "分辨率"=1.0, "数值 2"=w1557) -> ("输出2"=w1555:dbl)  [unwired: 3 in, 5 out]
                              }
                              frame 4 {
                                n758 = call "输出分辨率计算.vi"("偏移量"=sgl -40.0, "分辨率"=1.0, "数值 2"=w1561) -> ("输出2"=w1559:dbl)  [unwired: 3 in, 5 out]
                              }
                              frame 5..8 {
                                n759 = call "输出分辨率计算.vi"("分辨率"=1.0, "数值 2"=w1564) -> ("输出2"=w1562:dbl)  [unwired: 4 in, 5 out]
                              }
                            }
                          }
                          n760 = call "表格数据输入(数值)-8.6.vi"("行数"=u32 8, "列数"=u32 17, "数值数组"=w1528, "表格引用"=w1534) -> ()  [unwired: 8 out]
                          n761 = call "表格颜色-8.6.vi"("颜色类型"=w1531, "列数"=17, "行数"=8, "表格引用"=w1534) -> ()  [unwired: 1 in, 7 out]
                        }
                      }
                    }
                    frame Enabled {
                    }
                  }
                }
                frame 132 {
                  n762 = case shown="2" w1573 {
                    tunnel: w1572 -> [_ w1665 w1715 w1735 w1778]
                    tunnel: w1571 -> [_ w1662 w1709 w1728 w1766]
                    tunnel: [_ "电池信息1     读取成功" ("字符串") "电池包组号     读取成功" ("字符串") "充放电安时     读取成功" ("字符串") "电池充放电次数     读取成功" ("字符串")] -> w1567
                    tunnel: [_ w1574 w1693 w1716 w1752] -> w1566
                    frame 0, Default {
                    }
                    frame 1 {
                      w1646 = ":" ("字符串")
                      w1574 = TRUE ("写入超时")
                      w1652 = "-" ("字符串")
                      n763 = Reshape Array(w1665, 30 ("维数大小")) -> (w1663:u8[])
                      n764 = Unbundle By Name(w1662) -> ("电池信息"=w1661:refnum<vi>)
                      n765 = global read "读配置文件全局.vi" "电池信息"() -> (w1615:T9)
                      n766 = Index Array(array=w1663) -> (element #1=w1658:u8, element #2=w1659:u8, element #3=w1611:u8, element #4=w1578:u8, element #5=w1577:u8, element #6=w1641:u8, element #7=w1640:u8, element #8=w1639:u8, element #9=w1638:u8, element #10=w1637:u8, element #11=w1636:u8, element #12=w1630:u8, element #13=w1629:u8, element #14=w1628:u8, element #15=w1627:u8, element #16=w1624:u8, element #17=w1623:u8, element #21=w1621:u8, element #22=w1620:u8, element #23=w1619:u8, element #24=w1618:u8, element #25=w1617:u8, element #26=w1616:u8)  [unwired: 26 in, 3 out]
                      n767 = Join Numbers(hi=w1637, lo=w1636) -> ((hi.lo)=w1635:u16)
                      n768 = Join Numbers(hi=w1658, lo=w1659) -> ((hi.lo)=w1613:u16)
                      n769 = Join Numbers(hi=w1628, lo=w1627) -> ((hi.lo)=w1631:u16)
                      n770 = Join Numbers(hi=w1624, lo=w1623) -> ((hi.lo)=w1622:u16)
                      n771 = Join Numbers(hi=w1639, lo=w1638) -> ((hi.lo)=w1634:u16)
                      n772 = Join Numbers(hi=w1641, lo=w1640) -> ((hi.lo)=w1596:u16)
                      n773 = Join Numbers(hi=w1630, lo=w1629) -> ((hi.lo)=w1626:u16)
                      n774 = Unbundle By Name(w1615) -> ("电池串联"=w1614:dbl, "电池并联"=w1612:dbl, "电池厂家"=w1590:string, "电池类型"=w1588:string, "电池包额定能量"=w1610:dbl, "电池包额定容量"=w1608:dbl, "实际容量"=w1607:dbl, "电池包额定总电压"=w1606:dbl)
                      n775 = Join Numbers(hi=w1634, lo=w1635) -> ((hi.lo)=w1633:u32)
                      n776 = Join Numbers(hi=w1626, lo=w1631) -> ((hi.lo)=w1632:u32)
                      n777 = To Double Precision Float(number=w1633) -> (double precision float=w1595:dbl)
                      n778 = To Double Precision Float(number=w1632) -> (double precision float=w1594:dbl)
                      n779 = Number To Decimal String(number=w1578) -> (decimal integer string=w1576:string)  [unwired: 1 in]
                      n780 = Number To Decimal String(number=w1577) -> (decimal integer string=w1575:string)  [unwired: 1 in]
                      n781 = call "输出分辨率计算.vi"("数值1"=w1596, "分辨率"=0.1, "数值 4"=w1622) -> ("输出4"=w1605:dbl, "输出1"=w1609:dbl)  [unwired: 3 in, 4 out]
                      n782 = case shown="1" w1577 {
                        tunnel: [_ "磷酸铁锂" "锰酸锂" "三元材料" "铅酸" "镍氢" "钴酸锂" "聚合物锂离子" "钛酸锂" "其他电池"] -> w1587
                        frame 0, Default {
                        }
                        frame 1 {
                        }
                        frame 2 {
                        }
                        frame 3 {
                        }
                        frame 4 {
                        }
                        frame 5 {
                        }
                        frame 6 {
                        }
                        frame 7 {
                        }
                        frame 8 {
                        }
                        frame 9 {
                        }
                      }
                      n783 = case shown="1" w1578 {
                        tunnel: [_ "普莱德" "盟固利"] -> w1589
                        frame 0, Default {
                        }
                        frame 1 {
                        }
                        frame 2 {
                        }
                      }
                      n784 = Number To Decimal String(number=w1621) -> (decimal integer string=w1653:string)  [unwired: 1 in]
                      n785 = Number To Decimal String(number=w1620) -> (decimal integer string=w1651:string)  [unwired: 1 in]
                      n786 = Number To Decimal String(number=w1618) -> (decimal integer string=w1647:string)  [unwired: 1 in]
                      n787 = Number To Decimal String(number=w1619) -> (decimal integer string=w1650:string)  [unwired: 1 in]
                      n788 = Number To Decimal String(number=w1617) -> (decimal integer string=w1648:string)  [unwired: 1 in]
                      n789 = Number To Decimal String(number=w1616) -> (decimal integer string=w1649:string)  [unwired: 1 in]
                      n790 = call "输出分辨率计算.vi"("分辨率"=0.001, "数值 3"=w1594, "数值 2"=w1595) -> ("输出3"=w1591:dbl, "输出2"=w1592:dbl)  [unwired: 3 in, 4 out]
                      n791 = To Single Precision Float(number=w1607) -> (single precision float=w1584:sgl)
                      n792 = To Single Precision Float(number=w1606) -> (single precision float=w1583:sgl)
                      n793 = To Single Precision Float(number=w1610) -> (single precision float=w1586:sgl)
                      n794 = To Single Precision Float(number=w1608) -> (single precision float=w1585:sgl)
                      n795 = Concatenate Strings("20" ("字符串"), w1653, w1652, w1651, w1652, w1650) -> (w1645:string)
                      n796 = Concatenate Strings(w1647, w1646, w1648, w1646, w1649) -> (w1644:string)
                      n797 = call <vilib>:"Space Constant.vi"() -> ("String"=w1643:string)
                      n798 = To Single Precision Float(number=w1605) -> (single precision float=w1579:sgl)
                      n799 = To Single Precision Float(number=w1591) -> (single precision float=w1580:sgl)
                      n800 = Concatenate Strings(w1645, w1643, w1644) -> (w1642:string)
                      n801 = To Single Precision Float(number=w1609) -> (single precision float=w1582:sgl)
                      n802 = To Single Precision Float(number=w1592) -> (single precision float=w1581:sgl)
                      n803 = stacked-sequence {
                        seq-local: [w1666 _] -> [_ w1677]
                        seq-local: [w1667 _] -> [_ w1674]
                        tunnel: [_ w1673] -> _
                        tunnel: [_ w1672] -> w1604
                        tunnel: w1590 -> [w1671 w1681]
                        tunnel: w1589 -> [w1670 _]
                        tunnel: w1588 -> [w1669 w1680]
                        tunnel: w1587 -> [w1668 _]
                        tunnel: w1576 -> [_ w1679]
                        tunnel: w1575 -> [_ w1678]
                        frame #0 {
                          n804 = Equal?(x=w1670, y=w1671) -> (x = y?=w1667:bool)
                          n805 = Equal?(x=w1668, y=w1669) -> (x = y?=w1666:bool)
                        }
                        frame #1 {
                          n806 = Equal?(x=w1678, y=w1680) -> (x = y?=w1676:bool)
                          n807 = Equal?(x=w1679, y=w1681) -> (x = y?=w1675:bool)
                          n808 = Or(x=w1674, y=w1675) -> (x .or. y?=w1673:bool)
                          n809 = Or(x=w1676, y=w1677) -> (x .or. y?=w1672:bool)
                        }
                      }
                      n810 = Equal?(x=w1614, y=w1613) -> (x = y?=w1603:bool)
                      n811 = Equal?(x=w1612, y=w1611) -> (x = y?=w1602:bool)
                      n812 = property class="Clust (严格)"(reference=w1661) -> (reference out=w1656:refnum<vi>, "Value"=w1657:T9)  [unwired: 1 in, 1 out]
                      n813 = Bundle By Name(cluster=w1657, "电池串联"=w1613, "电池并联"=w1611, "电池厂家"=w1589, "电池类型"=w1587, "电池包额定能量"=w1609, "电池包额定容量"=w1592, "实际容量"=w1591, "电池包额定总电压"=w1605, "电池生产日期"=w1642) -> (w1655:T9)
                      n814 = Equal?(x=w1586, y=w1582) -> (x = y?=w1601:bool)
                      n815 = Equal?(x=w1581, y=w1585) -> (x = y?=w1600:bool)
                      n816 = Equal?(x=w1584, y=w1580) -> (x = y?=w1599:bool)
                      n817 = Equal?(x=w1583, y=w1579) -> (x = y?=w1598:bool)
                      n818 = property class="Clust (严格)"(reference=w1656, "Value"=w1655) -> ()  [unwired: 1 in, 2 out]
                      n819 = global write "EV05全局变量1.vi" "写入超时"(w1574) -> ()
                      n820 = Compound Arithmetic op=AND(w1604, w1603, w1602, w1601, w1600, w1599, w1598) -> (w1597:bool)
                      n821 = global write "读配置文件全局.vi" "电池信息1判定"(w1597) -> ()
                    }
                    frame 2 {
                      w1693 = TRUE ("写入超时")
                      n822 = Reshape Array(w1715, 4 ("维数大小")) -> (w1713:u8[])
                      n823 = Unbundle By Name(w1709) -> ("电池信息"=w1708:refnum<vi>)
                      n824 = global read "读配置文件全局.vi" "电池信息"() -> (w1702:T9)
                      n825 = Index Array(array=w1713) -> (element #1=w1706:u8, element #2=w1707:u8, element #3=w1704:u8, element #4=w1705:u8)  [unwired: 4 in]
                      n826 = Join Numbers(hi=w1706, lo=w1707) -> ((hi.lo)=w1700:u16)
                      n827 = Join Numbers(hi=w1704, lo=w1705) -> ((hi.lo)=w1699:u16)
                      n828 = Unbundle By Name(w1702) -> ("电池包组号"=w1696:string)
                      n829 = Join Numbers(hi=w1700, lo=w1699) -> ((hi.lo)=w1698:u32)
                      n830 = Number To Decimal String(number=w1698) -> (decimal integer string=w1697:string)  [unwired: 1 in]
                      n831 = Match Pattern(string=w1696, regular expression="-" ("正则表达式")) -> (before substring=w1695:string)  [unwired: 1 in, 3 out]
                      n832 = Equal?(x=w1697, y=w1695) -> (x = y?=w1701:bool)
                      n833 = global write "读配置文件全局.vi" "电池包组号判定"(w1701) -> ()
                      n834 = property class="Clust (严格)"(reference=w1708) -> (reference out=w1711:refnum<vi>, "Value"=w1712:T9)  [unwired: 1 in, 1 out]
                      n835 = Bundle By Name(cluster=w1712, "电池包组号"=w1697) -> (w1710:T9)
                      n836 = global write "EV05全局变量1.vi" "写入超时"(w1693) -> ()
                      n837 = property class="Clust (严格)"(reference=w1711, "Value"=w1710) -> ()  [unwired: 1 in, 2 out]
                    }
                    frame 3 {
                      w1716 = TRUE ("写入超时")
                      n838 = Reshape Array(w1735, 8 ("维数大小")) -> (w1733:u8[])
                      n839 = Unbundle By Name(w1728) -> ("电池信息"=w1727:refnum<vi>)
                      n840 = for {
                        N: 2 -> [_]
                        tunnel: w1733 -> [w1751]
                        tunnel: [w1736] -> w1726 mode=indexing
                        i -> [w1748]
                        n841 = Multiply(x=w1748, y=4) -> (x*y=w1749:i32)
                        n842 = Increment(x=w1749) -> (x+1=w1745:i32)
                        n843 = Increment(x=w1745) -> (x+1=w1744:i32)
                        n844 = Increment(x=w1744) -> (x+1=w1743:i32)
                        n845 = Index Array(array=w1751, index #1=w1749, index #2=w1745, index #3=w1744, index #4=w1743) -> (element #1=w1747:u8, element #2=w1746:u8, element #3=w1742:u8, element #4=w1741:u8)
                        n846 = Join Numbers(hi=w1747, lo=w1746) -> ((hi.lo)=w1739:u16)
                        n847 = Join Numbers(hi=w1742, lo=w1741) -> ((hi.lo)=w1740:u16)
                        n848 = Join Numbers(hi=w1739, lo=w1740) -> ((hi.lo)=w1737:u32)
                        n849 = call "输出分辨率计算.vi"("分辨率"=0.001, "数值 2"=w1737) -> ("输出2"=w1736:dbl)  [unwired: 4 in, 5 out]
                      }
                      n850 = global read "读配置文件全局.vi" "电池信息"() -> (w1724:T9)
                      n851 = Unbundle By Name(w1724) -> ("累计充电总安时"=w1723:dbl, "累计放电总安时"=w1722:dbl)
                      n852 = Index Array(array=w1726) -> (element #1=w1720:dbl, element #2=w1721:dbl)  [unwired: 2 in]
                      n853 = Equal?(x=w1720, y=w1723) -> (x = y?=w1718:bool)
                      n854 = Equal?(x=w1722, y=w1721) -> (x = y?=w1719:bool)
                      n855 = global write "EV05全局变量1.vi" "写入超时"(w1716) -> ()
                      n856 = And(x=w1718, y=w1719) -> (x .and. y?=w1717:bool)
                      n857 = property class="Clust (严格)"(reference=w1727) -> (reference out=w1730:refnum<vi>, "Value"=w1731:T9)  [unwired: 1 in, 1 out]
                      n858 = Bundle By Name(cluster=w1731, "累计充电总安时"=w1720, "累计放电总安时"=w1721) -> (w1729:T9)
                      n859 = global write "读配置文件全局.vi" "充放电安时判定"(w1717) -> ()
                      n860 = property class="Clust (严格)"(reference=w1730, "Value"=w1729) -> ()  [unwired: 1 in, 2 out]
                    }
                    frame 4 {
                      w1752 = TRUE ("写入超时")
                      n861 = global read "读配置文件全局.vi" "电池信息"() -> (w1763:T9)
                      n862 = Reshape Array(w1778, 6 ("维数大小")) -> (w1776:u8[])
                      n863 = Unbundle By Name(w1766) -> ("电池信息"=w1765:refnum<vi>)
                      n864 = Index Array(array=w1776) -> (element #1=w1774:u8, element #2=w1775:u8, element #3=w1773:u8, element #4=w1772:u8, element #5=w1771:u8, element #6=w1770:u8)  [unwired: 6 in]
                      n865 = Unbundle By Name(w1763) -> ("电池放空次数"=w1762:dbl, "电池充满次数"=w1761:dbl, "电池充电次数"=w1758:dbl)
                      n866 = Join Numbers(hi=w1774, lo=w1775) -> ((hi.lo)=w1760:u16)
                      n867 = Join Numbers(hi=w1773, lo=w1772) -> ((hi.lo)=w1759:u16)
                      n868 = Join Numbers(hi=w1771, lo=w1770) -> ((hi.lo)=w1757:u16)
                      n869 = Equal?(x=w1760, y=w1762) -> (x = y?=w1756:bool)
                      n870 = Equal?(x=w1761, y=w1759) -> (x = y?=w1755:bool)
                      n871 = Equal?(x=w1758, y=w1757) -> (x = y?=w1754:bool)
                      n872 = property class="Clust (严格)"(reference=w1765) -> (reference out=w1768:refnum<vi>, "Value"=w1769:T9)  [unwired: 1 in, 1 out]
                      n873 = Bundle By Name(cluster=w1769, "电池放空次数"=w1760, "电池充满次数"=w1759, "电池充电次数"=w1757) -> (w1767:T9)
                      n874 = Compound Arithmetic op=AND(w1756, w1755, w1754) -> (w1753:bool)
                      n875 = global write "读配置文件全局.vi" "电池充放电次数判定"(w1753) -> ()
                      n876 = property class="Clust (严格)"(reference=w1768, "Value"=w1767) -> ()  [unwired: 1 in, 2 out]
                      n877 = global write "EV05全局变量1.vi" "写入超时"(w1752) -> ()
                    }
                  }
                  n878 = Build Array(w1567) -> (w1570:string[])
                  n879 = call "表格编辑.vi"("新元素/子数组"=w1570, "活动单元格:单元格背景色"=u32 6618880, "MCListbox引用句柄"=w1568) -> ()  [unwired: 9 out]
                }
                frame 192 {
                  n880 = Index Array(array=w1782) -> (element #1=→"序号":u8, element #2=w1780:u8)  [unwired: 2 in]
                  n881 = Not Equal To 0?(x=w1780) -> (x != 0?=→"状态":bool)
                }
                frame 140 {
                  w1783 = TRUE ("写入超时")
                  n882 = Array Subset(array=w1793, length=30 ("长度")) -> (w1791:u8[])  [unwired: 1 in]
                  n883 = Byte Array To String(unsigned byte array=w1791) -> (string=w1786:string)
                  n884 = Concatenate Strings("BNET" ("字符串"), w1786) -> (w1785:string)
                  n885 = property class="Str"(reference="二维码信息", "Text.Text"=w1785) -> ()  [unwired: 1 in, 2 out]
                  n886 = global write "EV05全局变量1.vi" "写入超时"(w1783) -> ()
                  n887 = Build Array("二维码     读取成功" ("字符串")) -> (w1790:string[])
                  n888 = call "表格编辑.vi"("新元素/子数组"=w1790, "活动单元格:单元格背景色"=u32 6618880, "MCListbox引用句柄"=w1787) -> ()  [unwired: 9 out]
                }
              }
            }
            frame True {
            }
          }
        }
        frame "从板" {
          n889 = Not A Number/Path/Refnum?(number/path/refnum=w1798) -> (NaN/Path/Refnum?=w1797:bool)
          n890 = case shown="假" w1797 {
            tunnel: w1802 -> [w1810 _]
            tunnel: w1801 -> [w1809 _]
            tunnel: w1800 -> [w1808 _]
            tunnel: w1798 -> [w1806 _]
            tunnel: w1799 -> [w1805 _]
            tunnel: [w1804 _] -> w1796
            tunnel: w1795 -> [w1803 _]
            frame False {
              n891 = property class="Clust (严格)"(reference=w1806) -> ("Value"=w1807:T1)  [unwired: 1 in, 2 out]
              n892 = case shown="2" w1810 {
                tunnel: w1809 -> [_ w1819 w2017 w2252 _ w2468]
                tunnel: w1807 -> [_ w1818 w2015 w2250 _ w2466]
                tunnel: w1808 -> [_ w1817 w2016 w2251 w2451 w2467]
                tunnel: w1805 -> [_ w1814 w2014 w2247 w2450 w2463]
                tunnel: [_ w1812 w2013 w2245 w2449 w2461] -> w1804
                tunnel: w1803 -> [_ w1811 w2012 _ _ _]
                frame 153, Default {
                }
                frame 0 {
                  n893 = case shown="6" w1819 {
                    tunnel: w1818 -> [_ w1848 w1876 w1905 w1947 w1991 w2009]
                    tunnel: w1817 -> [_ w1846 w1873 w1902 w1944 w1993 w2011]
                    tunnel: [_ "电压起始值     读取成功" ("字符串") "通道电压节数     读取成功" ("字符串") "保险位置     读取成功" ("字符串") "温度起始值     读取成功" ("字符串") "加热控制参数     读取成功" ("字符串") "从板号     读取成功" ("字符串")] -> w1813
                    tunnel: [_ w1825 w1858 w1885 w1923 w1951 w1999] -> w1812
                    tunnel: w1811 -> [_ w1823 w1853 w1880 w1918 _ w1994]
                    frame 0, Default {
                    }
                    frame 1 {
                      w1825 = TRUE ("写入超时")
                      n894 = Unbundle By Name(w1848) -> ("项目信息 2"=w1847:refnum<vi>)
                      n895 = global read "读配置文件全局2.vi" "表格"() -> (w1837:string[])
                      n896 = Array Subset(array=w1846, length=4 ("长度")) -> (w1844:u8[])  [unwired: 1 in]
                      n897 = Array Subset(array=w1837, index=0 ("索引"), length=1 ("长度")) -> (w1834:string[])
                      n898 = Index Array(array=w1844) -> (element #1=w1842:u8, element #2=w1843:u8, element #3=w1841:u8, element #4=w1840:u8)  [unwired: 4 in]
                      n899 = for {
                        tunnel: w1834 -> [w1852] mode=indexing
                        tunnel: [w1851] -> w1833 mode=indexing
                        n900 = Fract/Exp String To Number(string=w1852) -> (number=w1851:dbl)  [unwired: 4 out]
                      }
                      n901 = Join Numbers(hi=w1842, lo=w1843) -> ((hi.lo)=w1839:u16)
                      n902 = Join Numbers(hi=w1841, lo=w1840) -> ()  [unwired: 1 out]
                      n903 = Build Array(w1839) -> (w1832:u16[])
                      n904 = global read "EV05全局变量1.vi" "写入超时Array"() -> (w1828:bool[])
                      n905 = Equal?(x=w1832, y=w1833) -> (x = y?=w1831:bool[])
                      n906 = local read "Socket"() -> (w1827:dbl)
                      n907 = And Array Elements(Boolean array=w1831) -> (logical AND=w1830:bool)
                      n908 = global write "读配置文件全局2.vi" "电压起始值判定"(w1830) -> ()
                      n909 = property class="Clust (严格)"(reference=w1823) -> (reference out=w1821:refnum<vi>, "Value"=w1824:T10)  [unwired: 1 in, 1 out]
                      n910 = Replace Array Subset(array=w1828, new element=TRUE ("写入超时"), index=w1827) -> (w1829:bool[])
                      n911 = global write "EV05全局变量1.vi" "写入超时Array"(w1829) -> ()
                      n912 = global write "EV05全局变量1.vi" "写入超时"(w1825) -> ()
                      n913 = Bundle By Name(cluster=w1824, "电压起始值"=TRUE ("从板号")) -> (w1822:T10)
                      n914 = call "表格数据输入(数值)-8.6.vi"("行数"=u32 0, "列数"=u32 1, "数值数组"=w1832, "表格引用"=w1847) -> ()  [unwired: 8 out]
                      n915 = property class="Clust (严格)"(reference=w1821, "Value"=w1822) -> ()  [unwired: 1 in, 2 out]
                    }
                    frame 2 {
                      w1858 = TRUE ("写入超时")
                      n916 = Unbundle By Name(w1876) -> ("项目信息 2"=w1875:refnum<vi>)
                      n917 = Array Subset(array=w1873, length=5 ("长度")) -> (w1863:u8[])  [unwired: 1 in]
                      n918 = global read "读配置文件全局2.vi" "表格"() -> (w1870:string[])
                      n919 = Array Subset(array=w1870, index=22 ("索引"), length=5 ("长度")) -> (w1867:string[])
                      n920 = global read "EV05全局变量1.vi" "写入超时Array"() -> (w1861:bool[])
                      n921 = for {
                        tunnel: w1867 -> [w1879] mode=indexing
                        tunnel: [w1878] -> w1866 mode=indexing
                        n922 = Fract/Exp String To Number(string=w1879) -> (number=w1878:dbl)  [unwired: 4 out]
                      }
                      n923 = local read "Socket"() -> (w1860:dbl)
                      n924 = Replace Array Subset(array=w1861, new element=TRUE ("写入超时"), index=w1860) -> (w1862:bool[])
                      n925 = Equal?(x=w1863, y=w1866) -> (x = y?=w1865:bool[])
                      n926 = property class="Clust (严格)"(reference=w1853) -> (reference out=w1855:refnum<vi>, "Value"=w1857:T10)  [unwired: 1 in, 1 out]
                      n927 = global write "EV05全局变量1.vi" "写入超时Array"(w1862) -> ()
                      n928 = And Array Elements(Boolean array=w1865) -> (logical AND=w1864:bool)
                      n929 = global write "EV05全局变量1.vi" "写入超时"(w1858) -> ()
                      n930 = global write "读配置文件全局2.vi" "通道电压判定"(w1864) -> ()
                      n931 = Bundle By Name(cluster=w1857, "通道电压数"=TRUE ("从板号")) -> (w1856:T10)
                      n932 = property class="Clust (严格)"(reference=w1855, "Value"=w1856) -> ()  [unwired: 1 in, 2 out]
                      n933 = call "表格数据输入(数值)-8.6.vi"("行数"=u32 22, "列数"=u32 1, "数值数组"=w1863, "表格引用"=w1875) -> ()  [unwired: 8 out]
                    }
                    frame 3 {
                      w1885 = TRUE ("写入超时")
                      n934 = Unbundle By Name(w1905) -> ("项目信息 2"=w1904:refnum<vi>)
                      n935 = Array Subset(array=w1902, length=10 ("长度")) -> (w1892:u8[])  [unwired: 1 in]
                      n936 = for {
                        tunnel: w1892 -> [w1915] mode=indexing
                        shift-right: [w1908] -> w1890
                        shift-left: i32[] [] -> [w1907]
                        n937 = call "二进制解析-8.6.vi"("索引"=4, "数值"=w1915) -> ("低位子数组"=w1913:i32[], "高位子数组"=w1912:i32[])  [unwired: 1 in, 1 out]
                        n938 = call "数值二进制转十进制-8.6.vi"("子数组"=w1912) -> ("十进制数值"=w1911:i32)  [unwired: 4 in]
                        n939 = call "数值二进制转十进制-8.6.vi"("子数组"=w1913) -> ("十进制数值"=w1910:i32)  [unwired: 4 in]
                        n940 = Build Array(w1911, w1910) -> (w1909:i32[])
                        n941 = Insert Into Array(array=w1907, new element=w1909) -> (w1908:i32[])  [unwired: 1 in]
                      }
                      n942 = global read "EV05全局变量1.vi" "写入超时Array"() -> (w1888:bool[])
                      n943 = global read "读配置文件全局2.vi" "表格"() -> (w1899:string[])
                      n944 = local read "Socket"() -> (w1887:dbl)
                      n945 = Array Subset(array=w1899, index=2 ("索引"), length=20 ("长度")) -> (w1896:string[])
                      n946 = Replace Array Subset(array=w1888, new element=TRUE ("写入超时"), index=w1887) -> (w1889:bool[])
                      n947 = for {
                        tunnel: w1896 -> [w1917] mode=indexing
                        tunnel: [w1916] -> w1895 mode=indexing
                        n948 = Fract/Exp String To Number(string=w1917) -> (number=w1916:dbl)  [unwired: 4 out]
                      }
                      n949 = property class="Clust (严格)"(reference=w1880) -> (reference out=w1882:refnum<vi>, "Value"=w1884:T10)  [unwired: 1 in, 1 out]
                      n950 = global write "EV05全局变量1.vi" "写入超时"(w1885) -> ()
                      n951 = global write "EV05全局变量1.vi" "写入超时Array"(w1889) -> ()
                      n952 = Equal?(x=w1890, y=w1895) -> (x = y?=w1894:bool[])
                      n953 = And Array Elements(Boolean array=w1894) -> (logical AND=w1893:bool)
                      n954 = Bundle By Name(cluster=w1884, "保险位置"=TRUE ("从板号")) -> (w1883:T10)
                      n955 = global write "读配置文件全局2.vi" "保险位置判定"(w1893) -> ()
                      n956 = property class="Clust (严格)"(reference=w1882, "Value"=w1883) -> ()  [unwired: 1 in, 2 out]
                      n957 = call "表格数据输入(数值)-8.6.vi"("行数"=u32 2, "列数"=u32 1, "数值数组"=w1890, "表格引用"=w1904) -> ()  [unwired: 8 out]
                    }
                    frame 4 {
                      w1923 = TRUE ("写入超时")
                      n958 = Unbundle By Name(w1947) -> ("项目信息 2"=w1946:refnum<vi>)
                      n959 = Array Subset(array=w1944, length=4 ("长度")) -> (w1942:u8[])  [unwired: 1 in]
                      n960 = global read "读配置文件全局2.vi" "表格"() -> (w1935:string[])
                      n961 = Index Array(array=w1942) -> (element #1=w1940:u8, element #2=w1941:u8, element #3=w1938:u8, element #4=w1939:u8)  [unwired: 4 in]
                      n962 = Join Numbers(hi=w1938, lo=w1939) -> ()  [unwired: 1 out]
                      n963 = Join Numbers(hi=w1940, lo=w1941) -> ((hi.lo)=w1937:u16)
                      n964 = Array Subset(array=w1935, index=1 ("索引"), length=1 ("长度")) -> (w1932:string[])
                      n965 = global read "EV05全局变量1.vi" "写入超时Array"() -> (w1926:bool[])
                      n966 = Build Array(w1937) -> (w1928:u16[])
                      n967 = for {
                        tunnel: w1932 -> [w1950] mode=indexing
                        tunnel: [w1949] -> w1931 mode=indexing
                        n968 = Fract/Exp String To Number(string=w1950) -> (number=w1949:dbl)  [unwired: 4 out]
                      }
                      n969 = local read "Socket"() -> (w1925:dbl)
                      n970 = Replace Array Subset(array=w1926, new element=TRUE ("写入超时"), index=w1925) -> (w1927:bool[])
                      n971 = Equal?(x=w1928, y=w1931) -> (x = y?=w1930:bool[])
                      n972 = global write "EV05全局变量1.vi" "写入超时Array"(w1927) -> ()
                      n973 = global write "EV05全局变量1.vi" "写入超时"(w1923) -> ()
                      n974 = And Array Elements(Boolean array=w1930) -> (logical AND=w1929:bool)
                      n975 = property class="Clust (严格)"(reference=w1918) -> (reference out=w1920:refnum<vi>, "Value"=w1922:T10)  [unwired: 1 in, 1 out]
                      n976 = global write "读配置文件全局2.vi" "温度起始值判定"(w1929) -> ()
                      n977 = Bundle By Name(cluster=w1922, "温度起始值"=TRUE ("从板号")) -> (w1921:T10)
                      n978 = property class="Clust (严格)"(reference=w1920, "Value"=w1921) -> ()  [unwired: 1 in, 2 out]
                      n979 = call "表格数据输入(数值)-8.6.vi"("行数"=u32 1, "列数"=u32 1, "数值数组"=w1928, "表格引用"=w1946) -> ()  [unwired: 8 out]
                    }
                    frame 5 {
                      w1951 = TRUE ("写入超时")
                      n980 = global read "读配置文件全局2.vi" "加热控制参数"() -> (w1980:dbl[])
                      n981 = Unbundle By Name(w1991) -> ("加热控制参数"=w1987:refnum<vi>)
                      n982 = Array Subset(array=w1993, length=7 ("索引")) -> (w1986:u8[])  [unwired: 1 in]
                      n983 = Index Array(array=w1986) -> (element #1=w1985:u8, element #2=w1984:u8, element #3=w1960:u8, element #4=w1959:u8, element #5=w1962:u8, element #6=w1961:u8, element #7=w1957:u8)  [unwired: 7 in]
                      n984 = Index Array(array=w1980) -> (element #1=w1979:dbl, element #2=w1977:dbl, element #3=w1976:dbl, element #4=w1975:dbl, element #5=w1974:dbl, element #6=w1973:dbl, element #7=w1958:dbl)  [unwired: 7 in]
                      n985 = call "输出分辨率计算.vi"("偏移量"=sgl -40.0, "数值1"=w1985, "分辨率"=1.0, "数值 4"=w1961, "数值 3"=w1962, "数值 2"=w1984) -> ("输出4"=w1970:dbl, "输出3"=w1971:dbl, "输出2"=w1972:dbl, "输出1"=w1978:dbl)  [unwired: 2 out]
                      n986 = property class="Clust (严格)"(reference=w1987) -> (reference out=w1989:refnum<vi>, "Value"=w1990:T6)  [unwired: 1 in, 1 out]
                      n987 = Equal?(x=w1974, y=w1960) -> (x = y?=w1965:bool)
                      n988 = Equal?(x=w1973, y=w1959) -> (x = y?=w1964:bool)
                      n989 = Equal?(x=w1979, y=w1978) -> (x = y?=w1969:bool)
                      n990 = Equal?(x=w1977, y=w1972) -> (x = y?=w1968:bool)
                      n991 = Equal?(x=w1976, y=w1971) -> (x = y?=w1967:bool)
                      n992 = Equal?(x=w1975, y=w1970) -> (x = y?=w1966:bool)
                      n993 = Equal?(x=w1958, y=w1957) -> (x = y?=w1956:bool)
                      n994 = Bundle By Name(cluster=w1990, "风机开启温度"=w1978, "风机关闭温度"=w1972, "加热开启温度"=w1971, "加热关闭温度"=w1970, "风机开启温差"=w1960, "风机关闭温差"=w1959, "加热关闭温差"=w1957) -> (w1988:T6)
                      n995 = Compound Arithmetic op=AND(w1969, w1968, w1967, w1966, w1965, w1964, w1956) -> (w1963:bool)
                      n996 = global read "EV05全局变量1.vi" "写入超时Array"() -> (w1954:bool[])
                      n997 = global write "读配置文件全局2.vi" "加热控制参数判定"(w1963) -> ()
                      n998 = property class="Clust (严格)"(reference=w1989, "Value"=w1988) -> ()  [unwired: 1 in, 2 out]
                      n999 = global write "EV05全局变量1.vi" "写入超时"(w1951) -> ()
                      n1000 = local read "Socket"() -> (w1953:dbl)
                      n1001 = Replace Array Subset(array=w1954, new element=TRUE ("写入超时"), index=w1953) -> (w1955:bool[])
                      n1002 = global write "EV05全局变量1.vi" "写入超时Array"(w1955) -> ()
                    }
                    frame 6 {
                      w1999 = TRUE ("写入超时")
                      n1003 = Index Array(array=w2011, index=0 ("索引")) -> (element=w2005:u8)
                      n1004 = Unbundle By Name(w2009) -> ("从板号"=w2008:refnum<vi>)
                      n1005 = global read "读配置文件全局2.vi" "从板板号"() -> (w2006:dbl)
                      n1006 = Equal?(x=w2005, y=w2006) -> (x = y?=w2004:bool)
                      n1007 = property class="DigNum (严格)"(reference=w2008, "Value"=w2005) -> ()  [unwired: 1 in, 2 out]
                      n1008 = global read "EV05全局变量1.vi" "写入超时Array"() -> (w2002:bool[])
                      n1009 = global write "读配置文件全局2.vi" "从板号判定"(w2004) -> ()
                      n1010 = local read "Socket"() -> (w2001:dbl)
                      n1011 = property class="Clust (严格)"(reference=w1994) -> (reference out=w1996:refnum<vi>, "Value"=w1998:T10)  [unwired: 1 in, 1 out]
                      n1012 = Replace Array Subset(array=w2002, new element=TRUE ("写入超时"), index=w2001) -> (w2003:bool[])
                      n1013 = global write "EV05全局变量1.vi" "写入超时Array"(w2003) -> ()
                      n1014 = global write "EV05全局变量1.vi" "写入超时"(w1999) -> ()
                      n1015 = Bundle By Name(cluster=w1998, "从板号"=TRUE) -> (w1997:T10)
                      n1016 = property class="Clust (严格)"(reference=w1996, "Value"=w1997) -> ()  [unwired: 1 in, 2 out]
                    }
                  }
                  n1017 = Build Array(w1813) -> (w1816:string[])
                  n1018 = call "表格编辑.vi"("新元素/子数组"=w1816, "活动单元格:单元格背景色"=u32 6618880, "MCListbox引用句柄"=w1814) -> ()  [unwired: 9 out]
                }
                frame 2 {
                  n1019 = case shown="1" w2017 {
                    tunnel: w2016 -> [_ w2092 w2169 w2244]
                    tunnel: w2015 -> [_ w2072 w2149 w2224]
                    tunnel: w2014 -> [_ w2067 w2144 w2219]
                    tunnel: [_ w2023 w2098 w2175] -> w2013
                    tunnel: w2012 -> [_ w2018 w2093 w2170]
                    frame 0, Default {
                    }
                    frame 1 {
                      w2023 = TRUE ("写入超时")
                      n1020 = Unbundle By Name(w2072) -> ("一级故障(从板)"=w2071:refnum<vi>)
                      n1021 = global read "读配置文件全局2.vi" "一级故障阀值"() -> (w2063:dbl[])
                      n1022 = Index Array(array=w2092, index #1=0 ("长度")) -> (element #1=w2089:u8, element #2=w2090:u8, element #3=w2088:u8, element #4=w2087:u8, element #5=w2086:u8, element #6=w2085:u8, element #7=w2081:u8, element #8=w2080:u8, element #9=w2050:u8, element #10=w2065:u8, element #11=w2066:u8)  [unwired: 10 in]
                      n1023 = Join Numbers(hi=w2089, lo=w2090) -> ((hi.lo)=w2084:u16)
                      n1024 = Join Numbers(hi=w2088, lo=w2087) -> ((hi.lo)=w2083:u16)
                      n1025 = Join Numbers(hi=w2086, lo=w2085) -> ((hi.lo)=w2077:u16)
                      n1026 = property class="Clust (严格)"(reference=w2018) -> (reference out=w2020:refnum<vi>, "Value"=w2022:T10)  [unwired: 1 in, 1 out]
                      n1027 = Join Numbers(hi=w2065, lo=w2066) -> ((hi.lo)=w2064:u16)
                      n1028 = call "输出分辨率计算.vi"("分辨率"=0.1, "数值 2"=w2064) -> ("输出2"=w2049:dbl)  [unwired: 4 in, 5 out]
                      n1029 = Index Array(array=w2063) -> (element #1=w2062:dbl, element #2=w2061:dbl, element #3=w2060:dbl, element #4=w2059:dbl, element #5=w2058:dbl, element #6=w2057:dbl, element #7=w2056:dbl)  [unwired: 7 in]
                      n1030 = call "输出分辨率计算.vi"("分辨率"=0.001, "数值 4"=w2077, "数值 3"=w2083, "数值 2"=w2084) -> ("输出4"=w2051:dbl, "输出3"=w2054:dbl, "输出2"=w2055:dbl)  [unwired: 2 in, 3 out]
                      n1031 = call "输出分辨率计算.vi"("偏移量"=sgl -40.0, "分辨率"=1.0, "数值 3"=w2080, "数值 2"=w2081) -> ("输出3"=w2052:dbl, "输出2"=w2053:dbl)  [unwired: 2 in, 4 out]
                      n1032 = Bundle By Name(cluster=w2022, "一级故障"=TRUE ("从板号")) -> (w2021:T10)
                      n1033 = To Single Precision Float(number=w2058) -> (single precision float=w2032:sgl)
                      n1034 = To Single Precision Float(number=w2057) -> (single precision float=w2030:sgl)
                      n1035 = To Single Precision Float(number=w2056) -> (single precision float=w2029:sgl)
                      n1036 = To Single Precision Float(number=w2049) -> (single precision float=w2028:sgl)
                      n1037 = To Single Precision Float(number=w2051) -> (single precision float=w2031:sgl)
                      n1038 = To Single Precision Float(number=w2059) -> (single precision float=w2034:sgl)
                      n1039 = To Single Precision Float(number=w2052) -> (single precision float=w2033:sgl)
                      n1040 = To Single Precision Float(number=w2060) -> (single precision float=w2036:sgl)
                      n1041 = To Single Precision Float(number=w2053) -> (single precision float=w2035:sgl)
                      n1042 = To Single Precision Float(number=w2062) -> (single precision float=w2040:sgl)
                      n1043 = To Single Precision Float(number=w2061) -> (single precision float=w2038:sgl)
                      n1044 = To Single Precision Float(number=w2054) -> (single precision float=w2037:sgl)
                      n1045 = To Single Precision Float(number=w2055) -> (single precision float=w2039:sgl)
                      n1046 = property class="Clust (严格)"(reference=w2020, "Value"=w2021) -> ()  [unwired: 1 in, 2 out]
                      n1047 = global read "EV05全局变量1.vi" "写入超时Array"() -> (w2026:bool[])
                      n1048 = Build Array("一级故障阀值     读取成功" ("字符串")) -> (w2070:string[])
                      n1049 = property class="Clust (严格)"(reference=w2071) -> (reference out=w2074:refnum<vi>, "Value"=w2075:T11)  [unwired: 1 in, 1 out]
                      n1050 = local read "Socket"() -> (w2025:dbl)
                      n1051 = Equal?(x=w2040, y=w2039) -> (x = y?=w2048:bool)
                      n1052 = Equal?(x=w2038, y=w2037) -> (x = y?=w2047:bool)
                      n1053 = Equal?(x=w2036, y=w2035) -> (x = y?=w2046:bool)
                      n1054 = Equal?(x=w2034, y=w2033) -> (x = y?=w2045:bool)
                      n1055 = Equal?(x=w2032, y=w2031) -> (x = y?=w2044:bool)
                      n1056 = Equal?(x=w2030, y=w2050) -> (x = y?=w2043:bool)
                      n1057 = Equal?(x=w2029, y=w2028) -> (x = y?=w2042:bool)
                      n1058 = Bundle By Name(cluster=w2075, "电压过高"=w2055, "电压过低"=w2054, "温度过高"=w2053, "温度过低"=w2052, "电压不均衡(V)"=w2051, "温度不均衡"=w2050, "SOC过低"=w2049) -> (w2073:T11)
                      n1059 = call "表格编辑.vi"("新元素/子数组"=w2070, "活动单元格:单元格背景色"=u32 6618880, "MCListbox引用句柄"=w2067) -> ()  [unwired: 9 out]
                      n1060 = Compound Arithmetic op=AND(w2048, w2047, w2046, w2045, w2044, w2043, w2042) -> (w2041:bool)
                      n1061 = Replace Array Subset(array=w2026, new element=TRUE ("写入超时"), index=w2025) -> (w2027:bool[])
                      n1062 = property class="Clust (严格)"(reference=w2074, "Value"=w2073) -> ()  [unwired: 1 in, 2 out]
                      n1063 = global write "读配置文件全局2.vi" "一级故障判定"(w2041) -> ()
                      n1064 = global write "EV05全局变量1.vi" "写入超时Array"(w2027) -> ()
                      n1065 = global write "EV05全局变量1.vi" "写入超时"(w2023) -> ()
                    }
                    frame 2 {
                      w2098 = TRUE ("写入超时")
                      n1066 = Unbundle By Name(w2149) -> ("二级故障(从板)"=w2148:refnum<vi>)
                      n1067 = Index Array(array=w2169, index #1=0 ("长度")) -> (element #1=w2166:u8, element #2=w2167:u8, element #3=w2165:u8, element #4=w2164:u8, element #5=w2163:u8, element #6=w2162:u8, element #7=w2158:u8, element #8=w2157:u8, element #9=w2119:u8, element #10=w2143:u8, element #11=w2142:u8)  [unwired: 10 in]
                      n1068 = global read "读配置文件全局2.vi" "二级故障阀值"() -> (w2140:dbl[])
                      n1069 = property class="Clust (严格)"(reference=w2093) -> (reference out=w2095:refnum<vi>, "Value"=w2097:T10)  [unwired: 1 in, 1 out]
                      n1070 = Join Numbers(hi=w2166, lo=w2167) -> ((hi.lo)=w2161:u16)
                      n1071 = Join Numbers(hi=w2165, lo=w2164) -> ((hi.lo)=w2160:u16)
                      n1072 = Join Numbers(hi=w2163, lo=w2162) -> ((hi.lo)=w2154:u16)
                      n1073 = Join Numbers(hi=w2143, lo=w2142) -> ((hi.lo)=w2141:u16)
                      n1074 = call "输出分辨率计算.vi"("分辨率"=0.1, "数值 2"=w2141) -> ("输出2"=w2118:dbl)  [unwired: 4 in, 5 out]
                      n1075 = Index Array(array=w2140) -> (element #1=w2139:dbl, element #2=w2138:dbl, element #3=w2137:dbl, element #4=w2136:dbl, element #5=w2135:dbl, element #6=w2134:dbl, element #7=w2133:dbl)  [unwired: 7 in]
                      n1076 = call "输出分辨率计算.vi"("分辨率"=0.001, "数值 4"=w2154, "数值 3"=w2160, "数值 2"=w2161) -> ("输出4"=w2120:dbl, "输出3"=w2123:dbl, "输出2"=w2124:dbl)  [unwired: 2 in, 3 out]
                      n1077 = call "输出分辨率计算.vi"("偏移量"=sgl -40.0, "分辨率"=1.0, "数值 3"=w2157, "数值 2"=w2158) -> ("输出3"=w2121:dbl, "输出2"=w2122:dbl)  [unwired: 2 in, 4 out]
                      n1078 = Bundle By Name(cluster=w2097, "二级故障"=TRUE ("从板号")) -> (w2096:T10)
                      n1079 = To Single Precision Float(number=w2123) -> (single precision float=w2116:sgl)
                      n1080 = To Single Precision Float(number=w2138) -> (single precision float=w2117:sgl)
                      n1081 = Build Array("二级故障阀值     读取成功" ("字符串")) -> (w2147:string[])
                      n1082 = global read "EV05全局变量1.vi" "写入超时Array"() -> (w2101:bool[])
                      n1083 = property class="Clust (严格)"(reference=w2095, "Value"=w2096) -> ()  [unwired: 1 in, 2 out]
                      n1084 = local read "Socket"() -> (w2100:dbl)
                      n1085 = To Single Precision Float(number=w2120) -> (single precision float=w2106:sgl)
                      n1086 = To Single Precision Float(number=w2133) -> (single precision float=w2104:sgl)
                      n1087 = To Single Precision Float(number=w2136) -> (single precision float=w2109:sgl)
                      n1088 = To Single Precision Float(number=w2135) -> (single precision float=w2107:sgl)
                      n1089 = To Single Precision Float(number=w2134) -> (single precision float=w2105:sgl)
                      n1090 = To Single Precision Float(number=w2122) -> (single precision float=w2110:sgl)
                      n1091 = To Single Precision Float(number=w2121) -> (single precision float=w2108:sgl)
                      n1092 = To Single Precision Float(number=w2118) -> (single precision float=w2103:sgl)
                      n1093 = To Single Precision Float(number=w2117) -> (single precision float=w2113:sgl)
                      n1094 = To Single Precision Float(number=w2116) -> (single precision float=w2112:sgl)
                      n1095 = To Single Precision Float(number=w2124) -> (single precision float=w2114:sgl)
                      n1096 = To Single Precision Float(number=w2137) -> (single precision float=w2111:sgl)
                      n1097 = To Single Precision Float(number=w2139) -> (single precision float=w2115:sgl)
                      n1098 = call "表格编辑.vi"("新元素/子数组"=w2147, "活动单元格:单元格背景色"=u32 6618880, "MCListbox引用句柄"=w2144) -> ()  [unwired: 9 out]
                      n1099 = property class="Clust (严格)"(reference=w2148) -> (reference out=w2151:refnum<vi>, "Value"=w2152:T11)  [unwired: 1 in, 1 out]
                      n1100 = Equal?(x=w2115, y=w2114) -> (x = y?=w2132:bool)
                      n1101 = Equal?(x=w2113, y=w2112) -> (x = y?=w2131:bool)
                      n1102 = Equal?(x=w2111, y=w2110) -> (x = y?=w2130:bool)
                      n1103 = Equal?(x=w2109, y=w2108) -> (x = y?=w2129:bool)
                      n1104 = Equal?(x=w2107, y=w2106) -> (x = y?=w2128:bool)
                      n1105 = Equal?(x=w2105, y=w2119) -> (x = y?=w2127:bool)
                      n1106 = Equal?(x=w2104, y=w2103) -> (x = y?=w2126:bool)
                      n1107 = Bundle By Name(cluster=w2152, "电压过高"=w2124, "电压过低"=w2116, "温度过高"=w2122, "温度过低"=w2121, "电压不均衡(V)"=w2120, "温度不均衡"=w2119, "SOC过低"=w2118) -> (w2150:T11)
                      n1108 = Replace Array Subset(array=w2101, new element=TRUE ("写入超时"), index=w2100) -> (w2102:bool[])
                      n1109 = global write "EV05全局变量1.vi" "写入超时Array"(w2102) -> ()
                      n1110 = Compound Arithmetic op=AND(w2132, w2131, w2130, w2129, w2128, w2127, w2126) -> (w2125:bool)
                      n1111 = global write "EV05全局变量1.vi" "写入超时"(w2098) -> ()
                      n1112 = property class="Clust (严格)"(reference=w2151, "Value"=w2150) -> ()  [unwired: 1 in, 2 out]
                      n1113 = global write "读配置文件全局2.vi" "二级故障判定"(w2125) -> ()
                    }
                    frame 3 {
                      w2175 = TRUE ("写入超时")
                      n1114 = Unbundle By Name(w2224) -> ("三级故障(从板)"=w2223:refnum<vi>)
                      n1115 = property class="Clust (严格)"(reference=w2170) -> (reference out=w2172:refnum<vi>, "Value"=w2174:T10)  [unwired: 1 in, 1 out]
                      n1116 = Index Array(array=w2244, index #1=0 ("长度")) -> (element #1=w2241:u8, element #2=w2242:u8, element #3=w2240:u8, element #4=w2239:u8, element #5=w2238:u8, element #6=w2237:u8, element #7=w2233:u8, element #8=w2232:u8, element #9=w2194:u8, element #10=w2218:u8, element #11=w2217:u8)  [unwired: 10 in]
                      n1117 = global read "读配置文件全局2.vi" "三级故障阀值"() -> (w2215:dbl[])
                      n1118 = Join Numbers(hi=w2241, lo=w2242) -> ((hi.lo)=w2236:u16)
                      n1119 = Join Numbers(hi=w2240, lo=w2239) -> ((hi.lo)=w2235:u16)
                      n1120 = Join Numbers(hi=w2238, lo=w2237) -> ((hi.lo)=w2229:u16)
                      n1121 = Join Numbers(hi=w2218, lo=w2217) -> ((hi.lo)=w2216:u16)
                      n1122 = call "输出分辨率计算.vi"("分辨率"=0.1, "数值 2"=w2216) -> ("输出2"=w2193:dbl)  [unwired: 4 in, 5 out]
                      n1123 = Bundle By Name(cluster=w2174, "三级故障"=TRUE ("从板号")) -> (w2173:T10)
                      n1124 = Index Array(array=w2215) -> (element #1=w2214:dbl, element #2=w2213:dbl, element #3=w2212:dbl, element #4=w2211:dbl, element #5=w2210:dbl, element #6=w2209:dbl, element #7=w2208:dbl)  [unwired: 7 in]
                      n1125 = call "输出分辨率计算.vi"("分辨率"=0.001, "数值 4"=w2229, "数值 3"=w2235, "数值 2"=w2236) -> ("输出4"=w2195:dbl, "输出3"=w2198:dbl, "输出2"=w2199:dbl)  [unwired: 2 in, 3 out]
                      n1126 = call "输出分辨率计算.vi"("偏移量"=sgl -40.0, "分辨率"=1.0, "数值 3"=w2232, "数值 2"=w2233) -> ("输出3"=w2196:dbl, "输出2"=w2197:dbl)  [unwired: 2 in, 4 out]
                      n1127 = global read "EV05全局变量1.vi" "写入超时Array"() -> (w2178:bool[])
                      n1128 = property class="Clust (严格)"(reference=w2172, "Value"=w2173) -> ()  [unwired: 1 in, 2 out]
                      n1129 = Build Array("三级故障阀值     读取成功" ("字符串")) -> (w2222:string[])
                      n1130 = local read "Socket"() -> (w2177:dbl)
                      n1131 = To Single Precision Float(number=w2208) -> (single precision float=w2181:sgl)
                      n1132 = To Single Precision Float(number=w2193) -> (single precision float=w2180:sgl)
                      n1133 = To Single Precision Float(number=w2211) -> (single precision float=w2186:sgl)
                      n1134 = To Single Precision Float(number=w2196) -> (single precision float=w2185:sgl)
                      n1135 = To Single Precision Float(number=w2210) -> (single precision float=w2184:sgl)
                      n1136 = To Single Precision Float(number=w2209) -> (single precision float=w2182:sgl)
                      n1137 = To Single Precision Float(number=w2195) -> (single precision float=w2183:sgl)
                      n1138 = To Single Precision Float(number=w2212) -> (single precision float=w2188:sgl)
                      n1139 = To Single Precision Float(number=w2197) -> (single precision float=w2187:sgl)
                      n1140 = To Single Precision Float(number=w2198) -> (single precision float=w2189:sgl)
                      n1141 = To Single Precision Float(number=w2214) -> (single precision float=w2192:sgl)
                      n1142 = To Single Precision Float(number=w2213) -> (single precision float=w2190:sgl)
                      n1143 = To Single Precision Float(number=w2199) -> (single precision float=w2191:sgl)
                      n1144 = call "表格编辑.vi"("新元素/子数组"=w2222, "活动单元格:单元格背景色"=u32 6618880, "MCListbox引用句柄"=w2219) -> ()  [unwired: 9 out]
                      n1145 = property class="Clust (严格)"(reference=w2223) -> (reference out=w2226:refnum<vi>, "Value"=w2227:T11)  [unwired: 1 in, 1 out]
                      n1146 = Equal?(x=w2192, y=w2191) -> (x = y?=w2207:bool)
                      n1147 = Equal?(x=w2190, y=w2189) -> (x = y?=w2206:bool)
                      n1148 = Equal?(x=w2188, y=w2187) -> (x = y?=w2205:bool)
                      n1149 = Equal?(x=w2186, y=w2185) -> (x = y?=w2204:bool)
                      n1150 = Equal?(x=w2184, y=w2183) -> (x = y?=w2203:bool)
                      n1151 = Equal?(x=w2182, y=w2194) -> (x = y?=w2202:bool)
                      n1152 = Equal?(x=w2181, y=w2180) -> (x = y?=w2201:bool)
                      n1153 = Replace Array Subset(array=w2178, new element=TRUE ("写入超时"), index=w2177) -> (w2179:bool[])
                      n1154 = Bundle By Name(cluster=w2227, "电压过高"=w2199, "电压过低"=w2198, "温度过高"=w2197, "温度过低"=w2196, "电压不均衡(V)"=w2195, "温度不均衡"=w2194, "SOC过低"=w2193) -> (w2225:T11)
                      n1155 = global write "EV05全局变量1.vi" "写入超时Array"(w2179) -> ()
                      n1156 = global write "EV05全局变量1.vi" "写入超时"(w2175) -> ()
                      n1157 = Compound Arithmetic op=AND(w2207, w2206, w2205, w2204, w2203, w2202, w2201) -> (w2200:bool)
                      n1158 = property class="Clust (严格)"(reference=w2226, "Value"=w2225) -> ()  [unwired: 1 in, 2 out]
                      n1159 = global write "读配置文件全局2.vi" "三级故障判定"(w2200) -> ()
                    }
                  }
                }
                frame 3 {
                  n1160 = case shown="0, 默认" w2252 {
                    tunnel: w2251 -> [_ w2256 w2326 w2345 w2381 w2396 w2407 w2448]
                    tunnel: w2250 -> [_ w2257 w2329 w2343 w2378 w2392 w2404 w2434]
                    tunnel: [_ "电池组信息1     读取成功" ("字符串") "电池包组号     读取成功" ("字符串") "充放电安时     读取成功" ("字符串") "充电次数时间     读取成功" ("字符串") "SOC     读取成功" ("字符串") "车牌号     读取成功" ("字符串") "充电参数     读取成功" ("字符串")] -> w2246
                    tunnel: [_ w2253 w2322 w2335 w2365 w2382 w2397 w2408] -> w2245
                    frame 0, Default {
                    }
                    frame 1 {
                      w2298 = ":" ("字符串")
                      w2309 = "-" ("字符串")
                      w2253 = TRUE ("写入超时")
                      n1161 = Unbundle By Name(w2257) -> ("电池组信息(从板)"=w2318:refnum<vi>)
                      n1162 = Reshape Array(w2256, 30 ("维数大小")) -> (w2319:u8[])
                      n1163 = Index Array(array=w2319) -> (element #1=w2316:u8, element #2=w2317:u8, element #3=w2266:u8, element #4=w2255:u8, element #5=w2254:u8, element #6=w2293:u8, element #7=w2292:u8, element #8=w2291:u8, element #9=w2290:u8, element #10=w2289:u8, element #11=w2288:u8, element #12=w2282:u8, element #13=w2281:u8, element #14=w2280:u8, element #15=w2279:u8, element #16=w2276:u8, element #17=w2275:u8, element #21=w2273:u8, element #22=w2272:u8, element #23=w2271:u8, element #24=w2270:u8, element #25=w2269:u8, element #26=w2268:u8)  [unwired: 26 in, 3 out]
                      n1164 = Join Numbers(hi=w2289, lo=w2288) -> ((hi.lo)=w2287:u16)
                      n1165 = Join Numbers(hi=w2316, lo=w2317) -> ((hi.lo)=w2267:u16)
                      n1166 = Join Numbers(hi=w2280, lo=w2279) -> ((hi.lo)=w2283:u16)
                      n1167 = Join Numbers(hi=w2276, lo=w2275) -> ((hi.lo)=w2274:u16)
                      n1168 = Join Numbers(hi=w2293, lo=w2292) -> ((hi.lo)=w2263:u16)
                      n1169 = Join Numbers(hi=w2291, lo=w2290) -> ((hi.lo)=w2286:u16)
                      n1170 = Join Numbers(hi=w2282, lo=w2281) -> ((hi.lo)=w2278:u16)
                      n1171 = Join Numbers(hi=w2286, lo=w2287) -> ((hi.lo)=w2285:u32)
                      n1172 = Join Numbers(hi=w2278, lo=w2283) -> ((hi.lo)=w2284:u32)
                      n1173 = To Double Precision Float(number=w2285) -> (double precision float=w2262:dbl)
                      n1174 = To Double Precision Float(number=w2284) -> (double precision float=w2261:dbl)
                      n1175 = call "输出分辨率计算.vi"("数值1"=w2263, "分辨率"=0.1, "数值 4"=w2274) -> ("输出4"=w2264:dbl, "输出1"=w2265:dbl)  [unwired: 3 in, 4 out]
                      n1176 = Number To Decimal String(number=w2273, width (-)=i16 2 ("宽度(-)")) -> (decimal integer string=w2311:string)
                      n1177 = Number To Decimal String(number=w2272, width (-)=i16 2 ("宽度(-)")) -> (decimal integer string=w2306:string)
                      n1178 = Number To Decimal String(number=w2270, width (-)=i16 2 ("宽度(-)")) -> (decimal integer string=w2299:string)
                      n1179 = Number To Decimal String(number=w2271, width (-)=i16 2 ("宽度(-)")) -> (decimal integer string=w2305:string)
                      n1180 = Number To Decimal String(number=w2269, width (-)=i16 2 ("宽度(-)")) -> (decimal integer string=w2303:string)
                      n1181 = Number To Decimal String(number=w2268, width (-)=i16 2 ("宽度(-)")) -> (decimal integer string=w2304:string)
                      n1182 = call "输出分辨率计算.vi"("分辨率"=0.001, "数值 3"=w2261, "数值 2"=w2262) -> ("输出3"=w2258:dbl, "输出2"=w2259:dbl)  [unwired: 3 in, 4 out]
                      n1183 = Concatenate Strings("20" ("字符串"), w2311, w2309, w2306, w2309, w2305) -> (w2297:string)
                      n1184 = Concatenate Strings(w2299, w2298, w2303, w2298, w2304) -> (w2296:string)
                      n1185 = call <vilib>:"Space Constant.vi"() -> ("String"=w2295:string)
                      n1186 = Concatenate Strings(w2297, w2295, w2296) -> (w2294:string)
                      n1187 = property class="Clust (严格)"(reference=w2318) -> (reference out=w2314:refnum<vi>, "Value"=w2315:T12)  [unwired: 1 in, 1 out]
                      n1188 = Bundle By Name(cluster=w2315, "串联数"=w2267, "并联数"=w2266, "电池厂家"=w2255, "电池类型"=w2254, "额定能量"=w2265, "额定容量"=w2259, "实际容量"=w2258, "额定总压"=w2264, "生产日期"=w2294) -> (w2313:T12)
                      n1189 = global write "EV05全局变量1.vi" "写入超时"(w2253) -> ()
                      n1190 = property class="Clust (严格)"(reference=w2314, "Value"=w2313) -> ()  [unwired: 1 in, 2 out]
                    }
                    frame 2 {
                      w2322 = TRUE ("写入超时")
                      n1191 = Unbundle By Name(w2329) -> ("电池组信息(从板)"=w2328:refnum<vi>)
                      n1192 = Index Array(array=w2326, index #1=0 ("索引"), index #2=1 ("索引")) -> (element #1=w2334:u8, element #2=w2333:u8)  [unwired: 1 in, 1 out]
                      n1193 = Join Numbers(hi=w2334, lo=w2333) -> ((hi.lo)=w2327:u16)
                      n1194 = property class="Clust (严格)"(reference=w2328) -> (reference out=w2331:refnum<vi>, "Value"=w2332:T12)  [unwired: 1 in, 1 out]
                      n1195 = Bundle By Name(cluster=w2332, "电池包组号"=w2327) -> (w2330:T12)
                      n1196 = global write "EV05全局变量1.vi" "写入超时"(w2322) -> ()
                      n1197 = property class="Clust (严格)"(reference=w2331, "Value"=w2330) -> ()  [unwired: 1 in, 2 out]
                    }
                    frame 3 {
                      w2335 = TRUE ("写入超时")
                      n1198 = Unbundle By Name(w2343) -> ("电池组信息(从板)"=w2342:refnum<vi>)
                      n1199 = Reshape Array(w2345, 8 ("维数大小")) -> (w2344:u8[])
                      n1200 = for {
                        N: 2 -> [_]
                        tunnel: w2344 -> [w2364]
                        tunnel: [w2349] -> w2346 mode=indexing
                        i -> [w2361]
                        n1201 = Multiply(x=w2361, y=4) -> (x*y=w2362:i32)
                        n1202 = Increment(x=w2362) -> (x+1=w2358:i32)
                        n1203 = Increment(x=w2358) -> (x+1=w2357:i32)
                        n1204 = Increment(x=w2357) -> (x+1=w2356:i32)
                        n1205 = Index Array(array=w2364, index #1=w2362, index #2=w2358, index #3=w2357, index #4=w2356) -> (element #1=w2360:u8, element #2=w2359:u8, element #3=w2355:u8, element #4=w2354:u8)
                        n1206 = Join Numbers(hi=w2360, lo=w2359) -> ((hi.lo)=w2352:u16)
                        n1207 = Join Numbers(hi=w2355, lo=w2354) -> ((hi.lo)=w2353:u16)
                        n1208 = Join Numbers(hi=w2352, lo=w2353) -> ((hi.lo)=w2350:u32)
                        n1209 = call "输出分辨率计算.vi"("分辨率"=0.001, "数值 2"=w2350) -> ("输出2"=w2349:dbl)  [unwired: 4 in, 5 out]
                      }
                      n1210 = Index Array(array=w2346) -> (element #1=w2340:dbl, element #2=w2339:dbl)  [unwired: 2 in]
                      n1211 = global write "EV05全局变量1.vi" "写入超时"(w2335) -> ()
                      n1212 = property class="Clust (严格)"(reference=w2342) -> (reference out=w2337:refnum<vi>, "Value"=w2341:T12)  [unwired: 1 in, 1 out]
                      n1213 = Bundle By Name(cluster=w2341, "充电总安时"=w2340, "放电总这时"=w2339) -> (w2338:T12)
                      n1214 = property class="Clust (严格)"(reference=w2337, "Value"=w2338) -> ()  [unwired: 1 in, 2 out]
                    }
                    frame 4 {
                      w2365 = TRUE ("写入超时")
                      n1215 = Unbundle By Name(w2378) -> ("电池组信息(从板)"=w2374:refnum<vi>)
                      n1216 = Index Array(array=w2381) -> (element #1=w2379:u8, element #2=w2380:u8, element #3=w2372:u8, element #4=w2371:u8, element #5=w2370:u8, element #6=w2369:u8)  [unwired: 6 in]
                      n1217 = Join Numbers(hi=w2372, lo=w2371) -> ((hi.lo)=w2368:u16)
                      n1218 = Join Numbers(hi=w2370, lo=w2369) -> ((hi.lo)=w2367:u16)
                      n1219 = Join Numbers(hi=w2379, lo=w2380) -> ((hi.lo)=w2373:u16)
                      n1220 = property class="Clust (严格)"(reference=w2374) -> (reference out=w2376:refnum<vi>, "Value"=w2377:T12)  [unwired: 1 in, 1 out]
                      n1221 = Bundle By Name(cluster=w2377, "放空次数"=w2373, "充满次数"=w2368, "充电次数"=w2367) -> (w2375:T12)
                      n1222 = global write "EV05全局变量1.vi" "写入超时"(w2365) -> ()
                      n1223 = property class="Clust (严格)"(reference=w2376, "Value"=w2375) -> ()  [unwired: 1 in, 2 out]
                    }
                    frame 5 {
                      w2382 = TRUE ("写入超时")
                      n1224 = Unbundle By Name(w2392) -> ("电池组信息(从板)"=w2388:refnum<vi>)
                      n1225 = Index Array(array=w2396, index #1=0 ("长度"), index #2=1 ("长度")) -> (element #1=w2384:u8, element #2=w2385:u8)
                      n1226 = Join Numbers(hi=w2384, lo=w2385) -> ((hi.lo)=w2383:u16)
                      n1227 = call "输出分辨率计算.vi"("分辨率"=0.1, "数值 2"=w2383) -> ("输出2"=w2387:dbl)  [unwired: 4 in, 5 out]
                      n1228 = global write "EV05全局变量1.vi" "写入超时"(w2382) -> ()
                      n1229 = property class="Clust (严格)"(reference=w2388) -> (reference out=w2390:refnum<vi>, "Value"=w2391:T12)  [unwired: 1 in, 1 out]
                      n1230 = Bundle By Name(cluster=w2391, "SOC"=w2387) -> (w2389:T12)
                      n1231 = property class="Clust (严格)"(reference=w2390, "Value"=w2389) -> ()  [unwired: 1 in, 2 out]
                    }
                    frame 6 {
                      w2397 = TRUE ("写入超时")
                      n1232 = Unbundle By Name(w2404) -> ("电池组信息(从板)"=w2400:refnum<vi>)
                      n1233 = Array Subset(array=w2407, length=7 ("长度")) -> (w2405:u8[])  [unwired: 1 in]
                      n1234 = Byte Array To String(unsigned byte array=w2405) -> (string=w2399:string)
                      n1235 = property class="Clust (严格)"(reference=w2400) -> (reference out=w2402:refnum<vi>, "Value"=w2403:T12)  [unwired: 1 in, 1 out]
                      n1236 = Bundle By Name(cluster=w2403, "车牌号"=w2399) -> (w2401:T12)
                      n1237 = global write "EV05全局变量1.vi" "写入超时"(w2397) -> ()
                      n1238 = property class="Clust (严格)"(reference=w2402, "Value"=w2401) -> ()  [unwired: 1 in, 2 out]
                    }
                    frame 7 {
                      w2408 = TRUE ("写入超时")
                      n1239 = Unbundle By Name(w2434) -> ("电池组信息(从板)"=w2433:refnum<vi>)
                      n1240 = Index Array(array=w2448) -> (element #1=w2446:u8, element #2=w2447:u8, element #3=w2444:u8, element #4=w2445:u8, element #5=w2426:u8, element #6=w2425:u8, element #7=w2443:u8, element #8=w2442:u8, element #9=w2418:u8, element #10=w2419:u8, element #11=w2416:u8, element #12=w2417:u8, element #13=w2415:u8, element #14=w2414:u8)  [unwired: 14 in]
                      n1241 = Join Numbers(hi=w2415, lo=w2414) -> ((hi.lo)=w2413:u16)
                      n1242 = Join Numbers(hi=w2418, lo=w2419) -> ((hi.lo)=w2410:u16)
                      n1243 = Join Numbers(hi=w2416, lo=w2417) -> ((hi.lo)=w2411:u16)
                      n1244 = Join Numbers(hi=w2446, lo=w2447) -> ((hi.lo)=w2441:u16)
                      n1245 = Join Numbers(hi=w2444, lo=w2445) -> ((hi.lo)=w2440:u16)
                      n1246 = Join Numbers(hi=w2443, lo=w2442) -> ((hi.lo)=w2437:u16)
                      n1247 = call "输出分辨率计算.vi"("分辨率"=0.001, "数值 3"=w2413, "数值 2"=w2441) -> ("输出3"=w2412:dbl, "输出2"=w2430:dbl)  [unwired: 3 in, 4 out]
                      n1248 = call "输出分辨率计算.vi"("分辨率"=0.1, "数值 2"=w2440) -> ("输出2"=w2429:dbl)  [unwired: 4 in, 5 out]
                      n1249 = call "输出分辨率计算.vi"("偏移量"=sgl 0.0, "分辨率"=0.1, "数值 3"=w2410, "数值 2"=w2437) -> ("输出3"=w2409:dbl, "输出2"=w2421:dbl)  [unwired: 2 in, 4 out]
                      n1250 = call "输出分辨率计算.vi"("偏移量"=sgl -40.0, "分辨率"=1.0, "数值 3"=w2425, "数值 2"=w2426) -> ("输出3"=w2423:dbl, "输出2"=w2424:dbl)  [unwired: 2 in, 4 out]
                      n1251 = global write "EV05全局变量1.vi" "写入超时"(w2408) -> ()
                      n1252 = property class="Clust (严格)"(reference=w2433) -> (reference out=w2422:refnum<vi>, "Value"=w2432:T12)  [unwired: 1 in, 1 out]
                      n1253 = Bundle By Name(cluster=w2432, "最大允许单体电压"=w2430, "最大允许总电压"=w2429, "最大允许温度"=w2424, "最小允许温度"=w2423, "最大允许充电电流"=w2421, "最小允许充电电流"=w2409, "电流步长"=w2411, "最小允许单体电压"=w2412) -> (w2431:T12)
                      n1254 = property class="Clust (严格)"(reference=w2422, "Value"=w2431) -> ()  [unwired: 1 in, 2 out]
                    }
                  }
                  n1255 = Build Array(w2246) -> (w2249:string[])
                  n1256 = call "表格编辑.vi"("新元素/子数组"=w2249, "活动单元格:单元格背景色"=u32 6618880, "MCListbox引用句柄"=w2247) -> ()  [unwired: 9 out]
                }
                frame 10 {
                  w2449 = TRUE ("写入超时")
                  n1257 = Array Subset(array=w2451, length=30 ("长度")) -> (w2459:u8[])  [unwired: 1 in]
                  n1258 = Byte Array To String(unsigned byte array=w2459) -> (string=w2455:string)
                  n1259 = Concatenate Strings("BNET" ("字符串"), w2455) -> (w2454:string)
                  n1260 = property class="Str"(reference="从板二维码信息", "Text.Text"=w2454) -> ()  [unwired: 1 in, 2 out]
                  n1261 = global write "EV05全局变量1.vi" "写入超时"(w2449) -> ()
                  n1262 = Build Array("二维码     读取成功" ("字符串")) -> (w2458:string[])
                  n1263 = call "表格编辑.vi"("新元素/子数组"=w2458, "活动单元格:单元格背景色"=u32 6618880, "MCListbox引用句柄"=w2450) -> ()  [unwired: 9 out]
                }
                frame 6 {
                  n1264 = case shown="0, 默认" w2468 {
                    tunnel: w2467 -> [_ w2497 w2552]
                    tunnel: w2466 -> [_ w2498 w2553]
                    tunnel: [_ "均衡阀值     读取成功" ("字符串") "充电结束电压     读取成功" ("字符串")] -> w2462
                    tunnel: [_ w2469 w2508] -> w2461
                    frame 0, Default {
                    }
                    frame 1 {
                      w2480 = 0.001 ("分辨率")
                      w2469 = TRUE ("写入超时")
                      n1265 = Reshape Array(w2497, 24 ("维数大小")) -> (w2505:u8[])
                      n1266 = Unbundle By Name(w2498) -> ("均衡参数"=w2504:refnum<vi>)
                      n1267 = Index Array(array=w2505) -> (element #1=w2502:u8, element #2=w2503:u8, element #3=w2496:u8, element #4=w2495:u8, element #5=w2494:u8, element #6=w2493:u8, element #7=w2492:u8, element #8=w2491:u8, element #9=w2490:u8, element #10=w2489:u8, element #11=w2488:u8, element #12=w2487:u8, element #13=w2486:u8, element #14=w2485:u8)  [unwired: 14 in]
                      n1268 = Join Numbers(hi=w2502, lo=w2503) -> ((hi.lo)=w2484:u16)
                      n1269 = Join Numbers(hi=w2496, lo=w2495) -> ((hi.lo)=w2483:u16)
                      n1270 = Join Numbers(hi=w2494, lo=w2493) -> ((hi.lo)=w2482:u16)
                      n1271 = Join Numbers(hi=w2492, lo=w2491) -> ((hi.lo)=w2481:u16)
                      n1272 = Join Numbers(hi=w2490, lo=w2489) -> ((hi.lo)=w2479:u16)
                      n1273 = Join Numbers(hi=w2488, lo=w2487) -> ((hi.lo)=w2478:u16)
                      n1274 = Join Numbers(hi=w2486, lo=w2485) -> ((hi.lo)=w2477:u16)
                      n1275 = call "输出分辨率计算.vi"("分辨率"=w2480, "数值 4"=w2477, "数值 3"=w2478, "数值 2"=w2479) -> ("输出4"=w2470:dbl, "输出3"=w2471:dbl, "输出2"=w2472:dbl)  [unwired: 2 in, 3 out]
                      n1276 = call "输出分辨率计算.vi"("数值1"=w2484, "分辨率"=w2480, "数值 4"=w2481, "数值 3"=w2482, "数值 2"=w2483) -> ("输出4"=w2473:dbl, "输出3"=w2474:dbl, "输出2"=w2475:dbl, "输出1"=w2476:dbl)  [unwired: 1 in, 2 out]
                      n1277 = property class="Clust (严格)"(reference=w2504) -> (reference out=w2500:refnum<vi>, "Value"=w2501:T13)  [unwired: 1 in, 1 out]
                      n1278 = Bundle By Name(cluster=w2501, "均衡计算-电压高阀值2级"=w2476, "均衡计算-电压高阀值1级"=w2475, "均衡计算-电压低阀值1级"=w2474, "均衡计算-电压低阀值2级"=w2473, "均衡计算-最低电压阀值"=w2472, "均衡停止-最低电压阀值"=w2471, "均衡计算-电压极差阀值"=w2470) -> (w2499:T13)
                      n1279 = global write "EV05全局变量1.vi" "写入超时"(w2469) -> ()
                      n1280 = property class="Clust (严格)"(reference=w2500, "Value"=w2499) -> ()  [unwired: 1 in, 2 out]
                    }
                    frame 2 {
                      w2517 = 0.001 ("分辨率")
                      w2508 = TRUE ("写入超时")
                      n1281 = Reshape Array(w2552, 22 ("维数大小")) -> (w2560:u8[])
                      n1282 = Unbundle By Name(w2553) -> ("均衡参数"=w2559:refnum<vi>)
                      n1283 = Index Array(array=w2560) -> (element #1=w2557:u8, element #2=w2558:u8, element #3=w2551:u8, element #4=w2550:u8, element #5=w2549:u8, element #6=w2548:u8, element #7=w2547:u8, element #8=w2546:u8, element #9=w2545:u8, element #10=w2544:u8, element #11=w2543:u8, element #12=w2542:u8, element #13=w2541:u8, element #14=w2540:u8, element #15=w2525:u8, element #16=w2524:u8, element #17=w2523:u8, element #18=w2522:u8, element #19=w2521:u8, element #20=w2520:u8, element #21=w2519:u8, element #22=w2518:u8)  [unwired: 22 in]
                      n1284 = Join Numbers(hi=w2557, lo=w2558) -> ((hi.lo)=w2539:u16)
                      n1285 = Join Numbers(hi=w2551, lo=w2550) -> ((hi.lo)=w2538:u16)
                      n1286 = Join Numbers(hi=w2549, lo=w2548) -> ((hi.lo)=w2537:u16)
                      n1287 = Join Numbers(hi=w2547, lo=w2546) -> ((hi.lo)=w2536:u16)
                      n1288 = Join Numbers(hi=w2545, lo=w2544) -> ((hi.lo)=w2535:u16)
                      n1289 = Join Numbers(hi=w2543, lo=w2542) -> ((hi.lo)=w2534:u16)
                      n1290 = Join Numbers(hi=w2541, lo=w2540) -> ((hi.lo)=w2533:u16)
                      n1291 = Join Numbers(hi=w2525, lo=w2524) -> ((hi.lo)=w2516:u16)
                      n1292 = Join Numbers(hi=w2523, lo=w2522) -> ((hi.lo)=w2515:u16)
                      n1293 = Join Numbers(hi=w2521, lo=w2520) -> ((hi.lo)=w2514:u16)
                      n1294 = Join Numbers(hi=w2519, lo=w2518) -> ((hi.lo)=w2513:u16)
                      n1295 = call "输出分辨率计算.vi"("数值1"=w2516, "分辨率"=w2517, "数值 4"=w2513, "数值 3"=w2514, "数值 2"=w2515) -> ("输出4"=w2509:dbl, "输出3"=w2510:dbl, "输出2"=w2511:dbl, "输出1"=w2512:dbl)  [unwired: 1 in, 2 out]
                      n1296 = call "输出分辨率计算.vi"("分辨率"=w2517, "数值 4"=w2533, "数值 3"=w2534, "数值 2"=w2535) -> ("输出4"=w2526:dbl, "输出3"=w2527:dbl, "输出2"=w2528:dbl)  [unwired: 2 in, 3 out]
                      n1297 = call "输出分辨率计算.vi"("数值1"=w2539, "分辨率"=w2517, "数值 4"=w2536, "数值 3"=w2537, "数值 2"=w2538) -> ("输出4"=w2529:dbl, "输出3"=w2530:dbl, "输出2"=w2531:dbl, "输出1"=w2532:dbl)  [unwired: 1 in, 2 out]
                      n1298 = property class="Clust (严格)"(reference=w2559) -> (reference out=w2555:refnum<vi>, "Value"=w2556:T13)  [unwired: 1 in, 1 out]
                      n1299 = Bundle By Name(cluster=w2556, "充电结束电压(90%)"=w2532, "充电结束电压(91%)"=w2531, "充电结束电压(92%)"=w2530, "充电结束电压(93%)"=w2529, "充电结束电压(94%)"=w2528, "充电结束电压(95%)"=w2527, "充电结束电压(96%)"=w2526, "充电结束电压(97%)"=w2512, "充电结束电压(98%)"=w2511, "充电结束电压(99%)"=w2510, "充电结束电压(100%)"=w2509) -> (w2554:T13)
                      n1300 = global write "EV05全局变量1.vi" "写入超时"(w2508) -> ()
                      n1301 = property class="Clust (严格)"(reference=w2555, "Value"=w2554) -> ()  [unwired: 1 in, 2 out]
                    }
                  }
                  n1302 = Build Array(w2462) -> (w2465:string[])
                  n1303 = call "表格编辑.vi"("新元素/子数组"=w2465, "活动单元格:单元格背景色"=u32 6618880, "MCListbox引用句柄"=w2463) -> ()  [unwired: 9 out]
                }
              }
            }
            frame True {
            }
          }
        }
      }
    }
  }
  "写入超时" <- w2
  n1304 = disable-structure shown="禁用" {
    frame Disabled {
      n1305 = global read "读配置文件全局2.vi" "表格"() -> (w2569:string[])
      n1306 = Array Subset(array=w2569, index=0 ("索引"), length=2 ("长度")) -> (w2566:string[])
      n1307 = for {
        tunnel: w2566 -> [w2571] mode=indexing
        tunnel: [w2570] -> w2565 mode=indexing
        n1308 = Fract/Exp String To Number(string=w2571) -> (number=w2570:dbl)  [unwired: 4 out]
      }
      n1309 = Equal?(y=w2565) -> (x = y?=w2564:bool[])  [unwired: 1 in]
      n1310 = And Array Elements(Boolean array=w2564) -> (logical AND=w2563:bool)
      n1311 = global write "读配置文件全局2.vi" "电压起始值判定"(w2563) -> ()
    }
    frame Enabled {
    }
  }
